vi "Omniax_mDrive_XYZR_MM_BR_RES_2_NC_GR_pxi.vi"() -> ()   [LabVIEW 2009]
uses:
  <vilib>/Instr/_visa.llb/VISA Configure Serial Port (Instr).vi
panel:
  out "XY Graph 2":cluster{"Y":dbl[], "Y":dbl[]}[](graph)
  out "XY Graph":cluster{"Y":dbl[], "Y":dbl[]}[](graph)
  out "X Scan Duration":dbl
  out "Y Scan Duration":dbl
  out "Z Scan Duration":dbl
  out "R Scan Duration":dbl
  out "R Backlash steps/sec":i32
  out "R Backlash":i32
  out "R Holding Current %":i32
  out "R Run Current %":i32
  out "R offset deg":dbl
  out "R deg/rev":dbl
  out "R steps/rev":u32
  out "R velocity PV step/sec":i32
  out "R MINPOS":i32=-94296
  out "R MAXPOS":i32=-34296
  out "R COM PORT":refnum<visa-resource-name>="COM5"
  in  "R Scan set":bool
  in  "R Scan Velocity SP deg/sec":dbl
  in  "R Scan Length SP deg":dbl
  in  "R Move Set":bool
  out "Reset R Motor Steps":i32
  in  "Reset R Position deg":dbl
  out "R Velocity MVdeg/sec":dbl
  in  "R Velocity SP deg/sec":dbl
  in  "R Position SP deg":dbl
  out "R Position MV deg":dbl
  out "R Scan velocity MV deg/sec":dbl format="%#_6f"
  out "R Scan length MV deg":dbl
  in  "R Scan Length SP steps":i32 min=0 max=6144000 step=100
  in  "R Scan OK":bool
  in  "R Velocity SP step/sec":i32 min=1 max=20000
  in  "R Scan Velocity SP steps/sec":i32=1 min=1 max=102400 step=1
  in  "R Go":bool
  in  "R Step SP":i32=-20000 min=-6144000 max=0 step=500
  out "R Position deg PV":dbl
  out "R Step PV":i32 max=2000
  out "R Backlash corr":bool
  out "R in Motion":bool
  out "R Scan":bool
  out "R in Range":bool
  out "Z COM PORT":refnum<visa-resource-name>="COM5"
  out "Z Backlash steps/sec":i32
  out "Z Backlash":i32
  out "Z Holding Current %":i32
  out "Z Run Current %":i32
  out "Z offset mm":dbl
  out "Z mm/rev":dbl
  out "Z steps/rev":u32
  out "Z  velocity PV step/sec":i32
  out "Z MINPOS":i32=-94296
  out "Z MAXPOS":i32=-34296
  in  "Z Scan set":bool
  in  "Z Scan Velocity SP mm/sec":dbl
  in  "Z Scan Length SP mm":dbl
  in  "Z Move Set":bool
  out "Reset Z Motor Steps":i32
  in  "Reset Z Position mm":dbl
  out "Z Velocity MV mm/sec":dbl
  in  "Z Velocity SP mm/sec":dbl
  in  "Z Position SP mm":dbl
  out "Z Position MV mm":dbl
  out "Z Scan velocity MV mm/sec":dbl format="%#_6f"
  out "Z Scan length MV mm":dbl
  in  "Z Scan Length SP steps":i32 min=0 max=2048000 step=100
  in  "Z Scan OK":bool
  in  "Z Velocity SP step/sec":i32 min=1 max=102400
  in  "Z Scan Velocity SP steps/sec":i32=1 min=1 max=102400 step=1
  in  "Z Go":bool
  in  "Z Step SP":i32=-20000 min=0 max=102400000 step=500
  out "Z Position mm PV":dbl
  out "Z Step PV":i32 max=2000
  out "Z Backlash corr":bool
  out "Z in Motion":bool
  out "Z Scan":bool
  out "Z in Range":bool
  out "Reset X Motor Steps":i32
  in  "Reset X Position mm":dbl
  out "X Backlash corr":bool
  out "X  in Motion":bool
  out "X Scan":bool
  out "X  in Range":bool
  out "X Step PV":i32 max=2000
  out "X Position mm PV":dbl
  out "X velocity PV step/sec":i32
  in  "X Scan set":bool
  in  "X Scan Velocity SP mm/sec":dbl
  in  "X Scan Length SP mm":dbl
  in  "X Move Set":bool
  out "X Velocity MV mm/sec":dbl
  in  "X Velocity SP mm/sec":dbl
  in  "X Position SP mm":dbl
  out "X Position MV mm":dbl
  out "X Scan velocity MV mm/sec":dbl format="%#_6f"
  out "X Scan length MV mm":dbl
  in  "X Scan Length SP steps":i32 min=-2304000 max=2304000 step=100
  in  "X Scan OK":bool
  in  "X Velocity SP step/sec":i32 min=1 max=25600
  in  "X Scan Velocity SP steps/sec":i32=1 min=1 max=102400 step=1
  in  "X Go":bool
  in  "X Step SP":i32=-20000 min=-2304000 max=2304000 step=500
  out "X Backlash steps/sec":i32
  out "X Backlash":i32
  out "X Holding Current %":i32
  out "X Run Current %":i32
  out "X offset mm":dbl
  out "X mm/rev":dbl
  out "X steps/rev":u32
  out "X MAXPOS":i32=-34296
  out "X MINPOS":i32=-94296
  out "X COM PORT":refnum<visa-resource-name>="COM5"
  out "Y Backlash corr":bool
  in  "Y Scan set":bool
  in  "Y Scan Velocity SP mm/sec":dbl
  in  "Y Scan Length SP mm":dbl
  in  "Y Move Set":bool
  out "Y Backlash steps/sec":i32
  out "Y Backlash":i32
  out "Y in Motion":bool
  in  "Reset":bool
  out "Reset Y Motor Steps":i32
  in  "Reset Y Position mm":dbl
  out "Y Velocity MV mm/sec":dbl
  in  "Y Velocity SP mm/sec":dbl
  in  "Y Position SP mm":dbl
  out "Y Position MV mm":dbl
  out "Y Holding Current %":i32
  out "Y Run Current %":i32
  out "Y Scan velocity MV mm/sec":dbl format="%#_6f"
  out "Y Scan length MV mm":dbl
  in  "Scan Cancel":bool
  out "Y Position mm PV":dbl
  out "Y offset mm":dbl
  out "Y mm/rev":dbl
  out "Y steps/rev":u32
  out "Y velocity PV step/sec":i32
  in  "Y Scan Length SP steps":i32 min=-2304000 max=2304000 step=100
  out "Y Scan":bool
  in  "Y Scan OK":bool
  in  "Scan Go":bool
  in  "Y Velocity SP step/sec":i32 min=1 max=25600
  in  "Y Scan Velocity SP steps/sec":i32=1 min=1 max=102400 step=1
  in  "Stop":bool
  out "Y in Range":bool
  out "Y Step PV":i32 max=2000
  in  "Y Go":bool
  in  "Y Step SP":i32=-20000 min=-2304000 max=2304000 step=500
  out "Y MINPOS":i32=-94296
  out "Y MAXPOS":i32=-34296
  out "Y COM PORT":refnum<visa-resource-name>="COM5"
  # "L"
  # "M"
  # "B"
  # "S"
  # "MX"
  # "MY"
  # "MZ"
  # "MR"
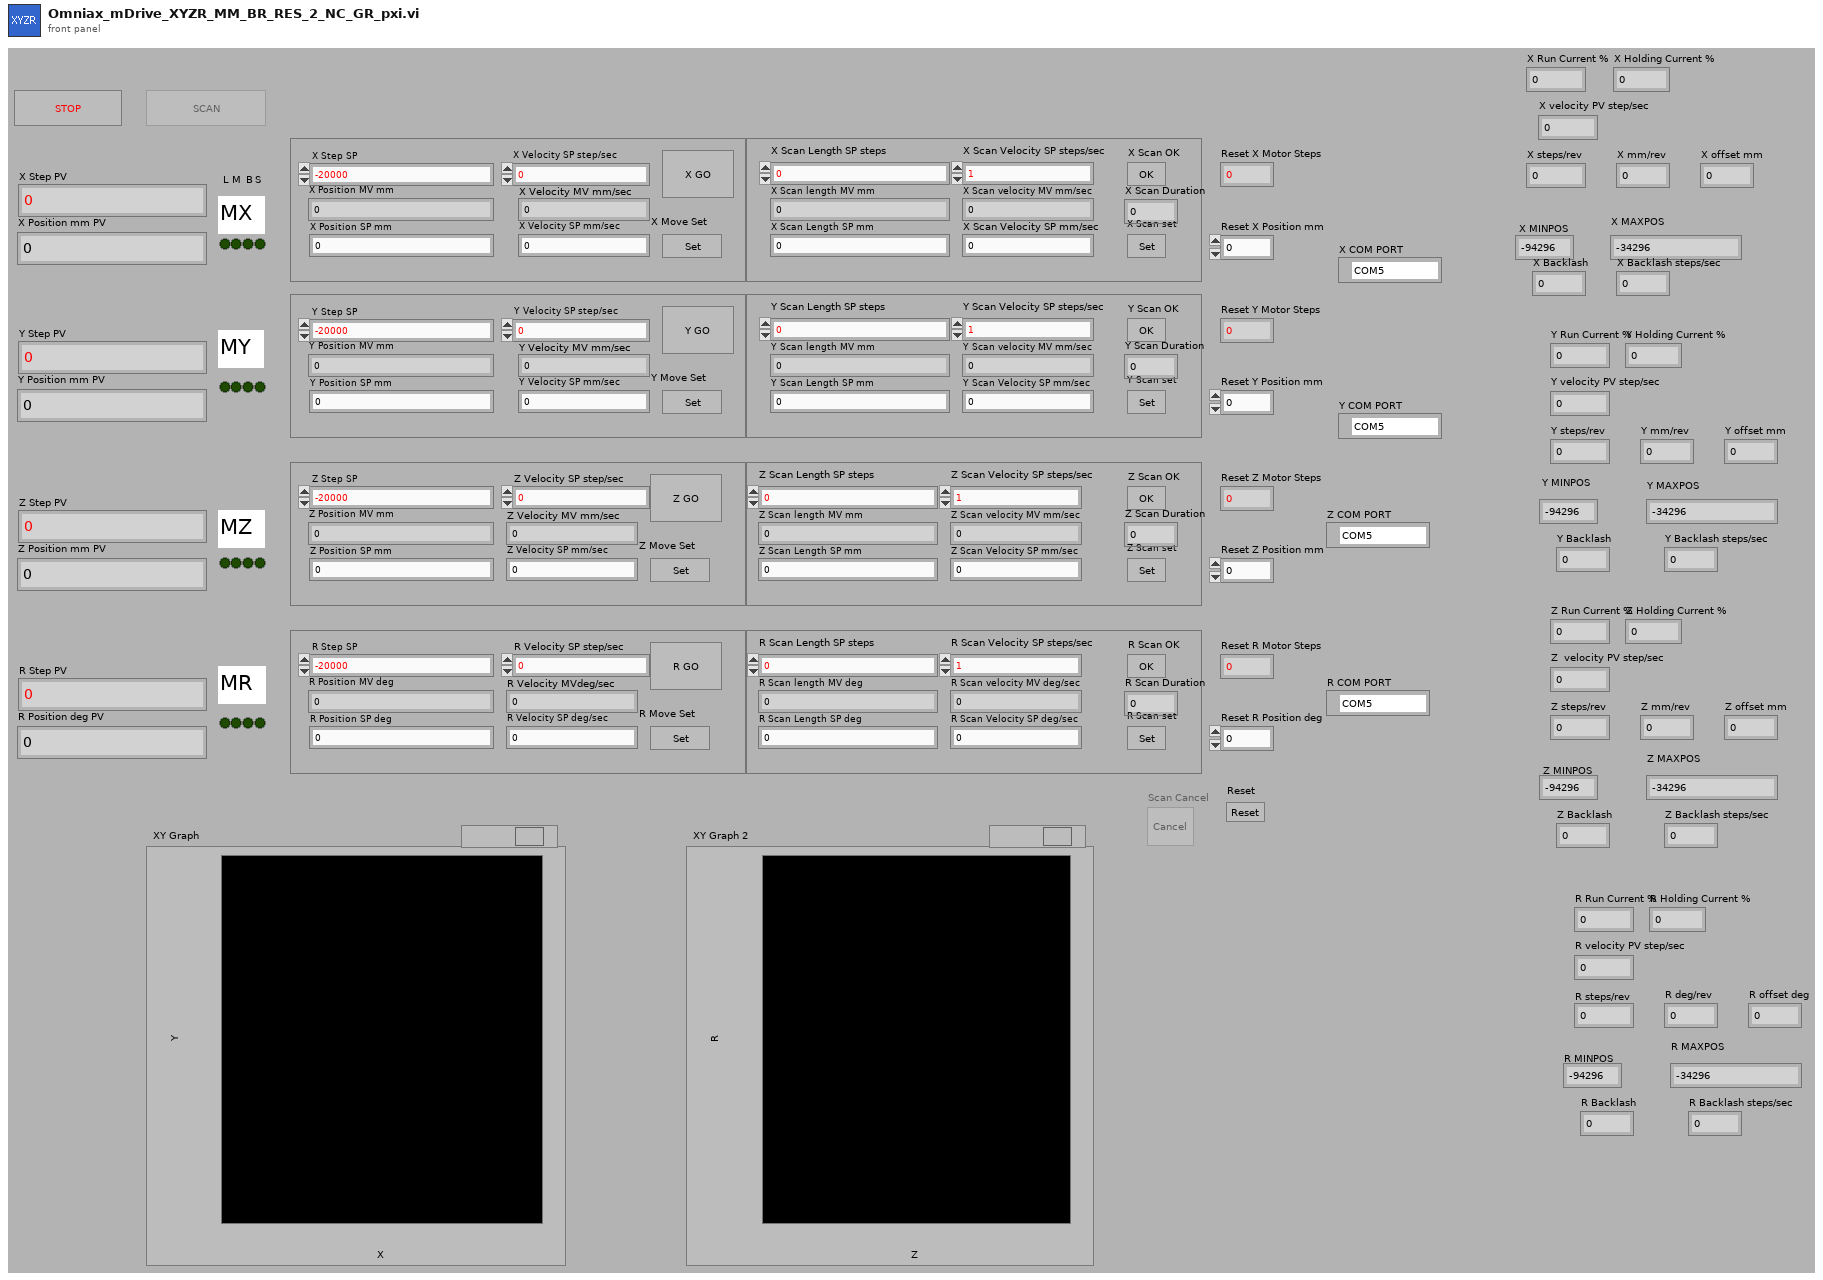
[diagram p1: front panel]
types:
  T1 = enum8{"Enabled", "Disabled", "Disabled and Grayed Out"}
  T2 = enum16{"Stop", "Reset", "Run Current", "Holding Current", "Accel Rate", "Decel Rate", "Move to Relative Position", "Move to Absolute Position", "Echo Mode", "Print Parameter", "Send String", "Microstep Resolution", "Set Current Position", "Max Velocity"}
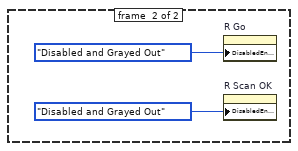
[diagram p2: hidden frame]
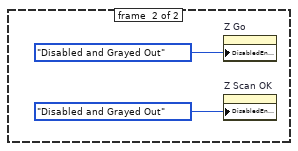
[diagram p5: hidden frame]
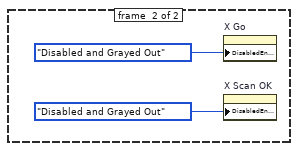
[diagram p8: hidden frame]
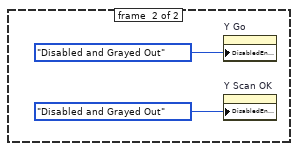
[diagram p11: hidden frame]
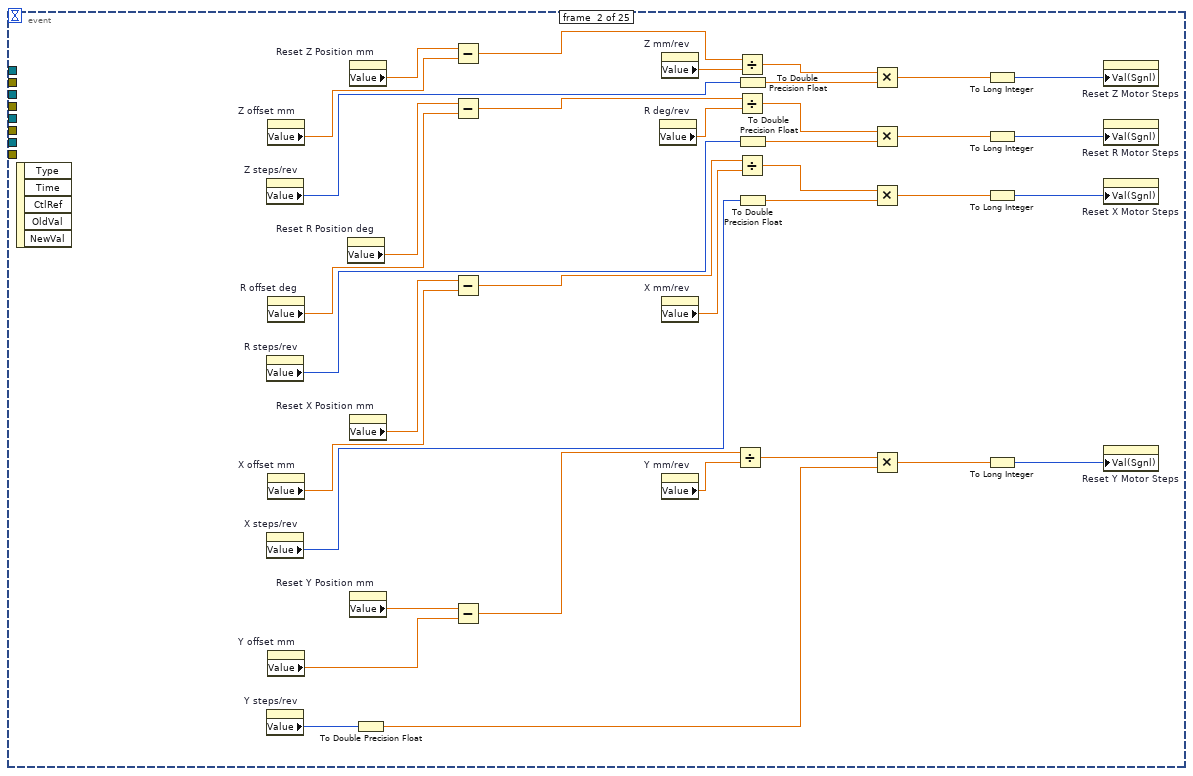
[diagram p14: hidden frame]
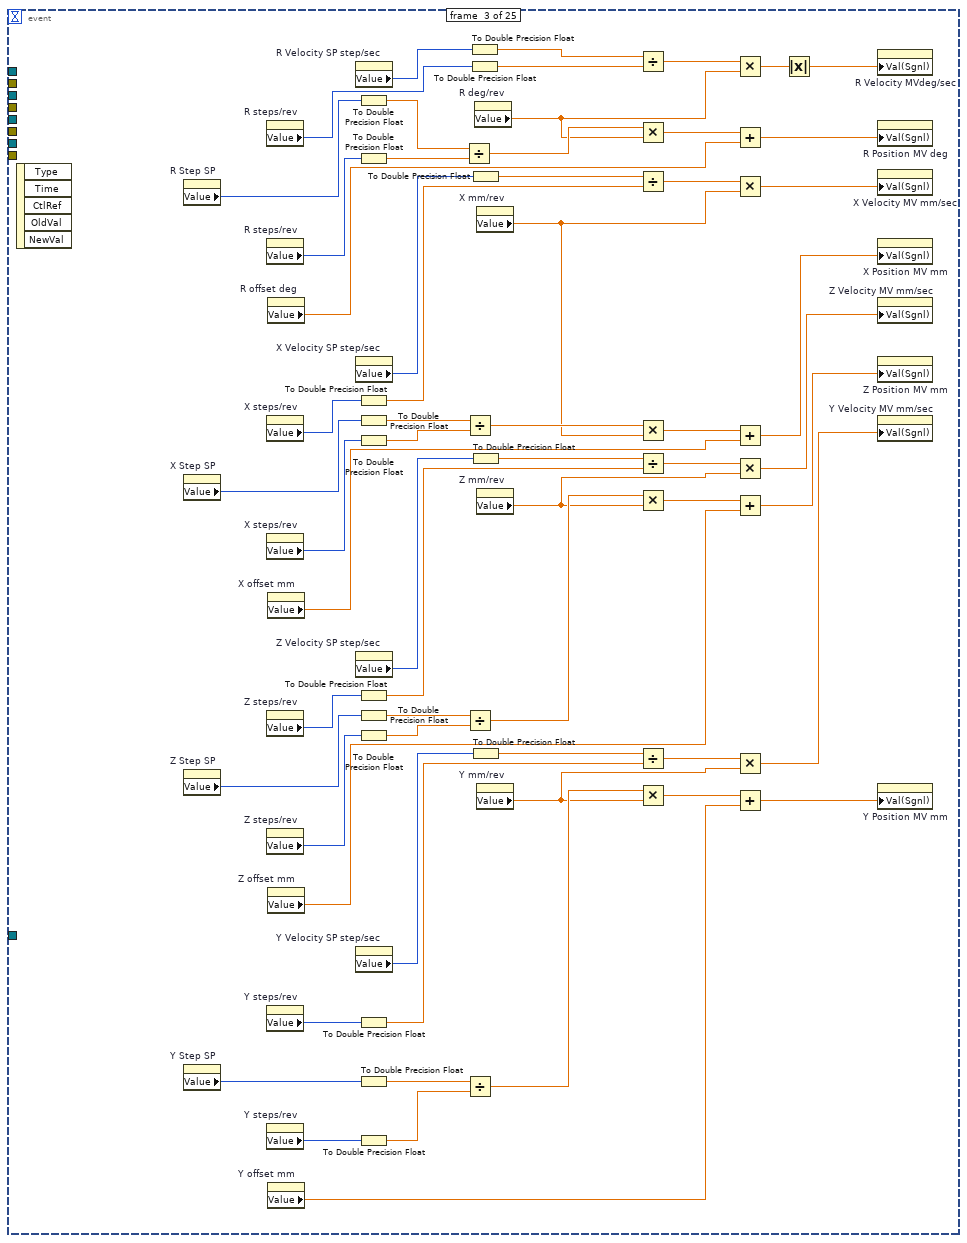
[diagram p15: hidden frame]
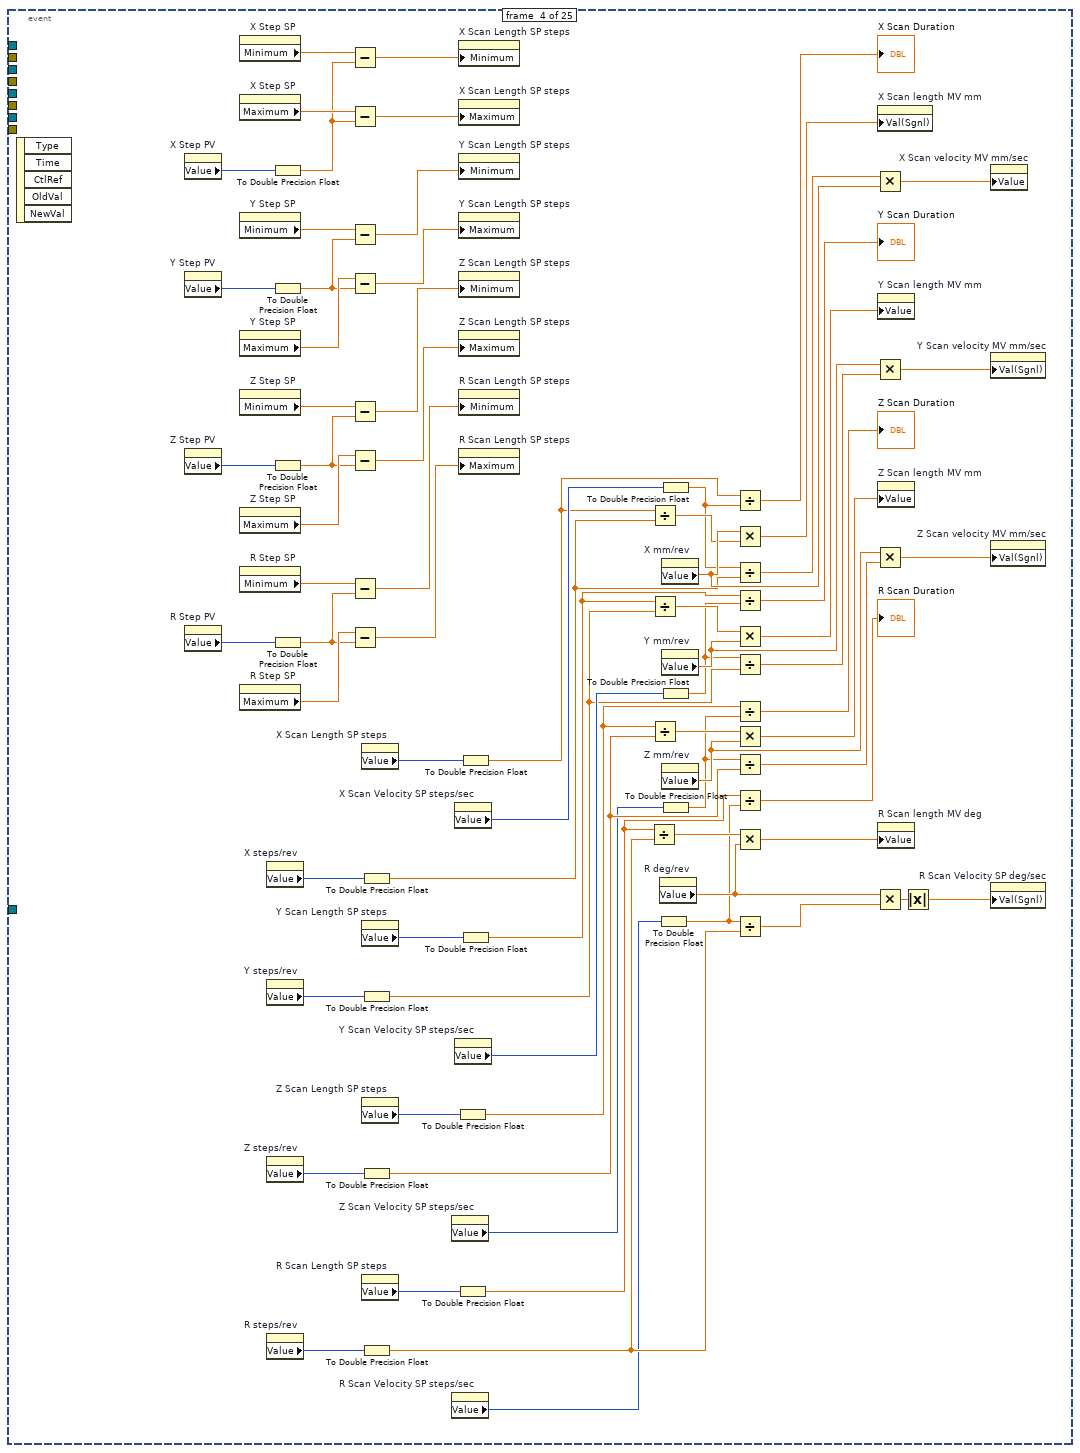
[diagram p16: hidden frame]
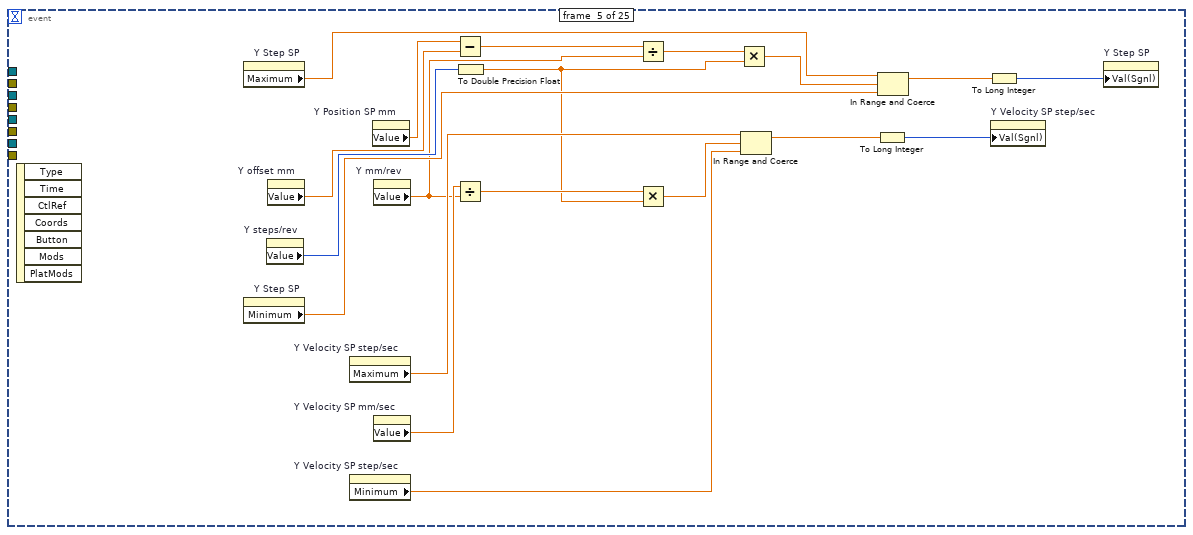
[diagram p17: hidden frame]
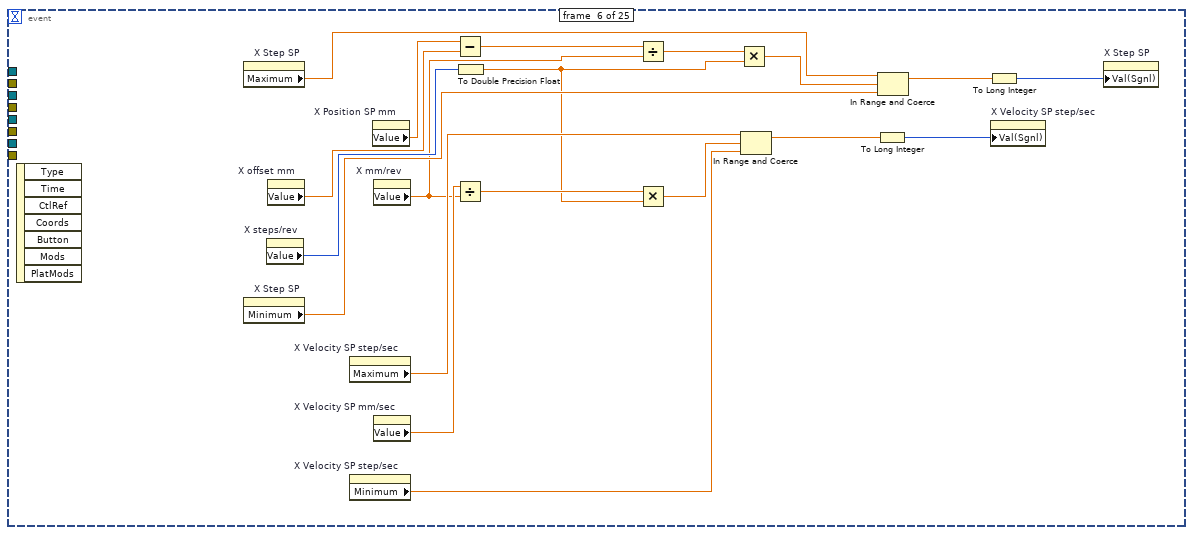
[diagram p18: hidden frame]
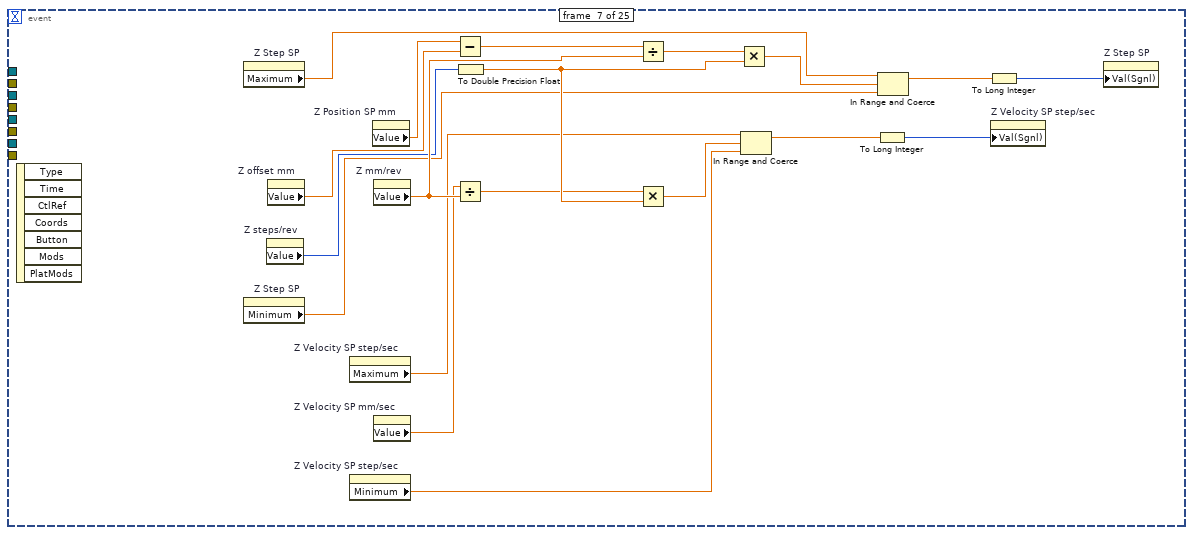
[diagram p19: hidden frame]
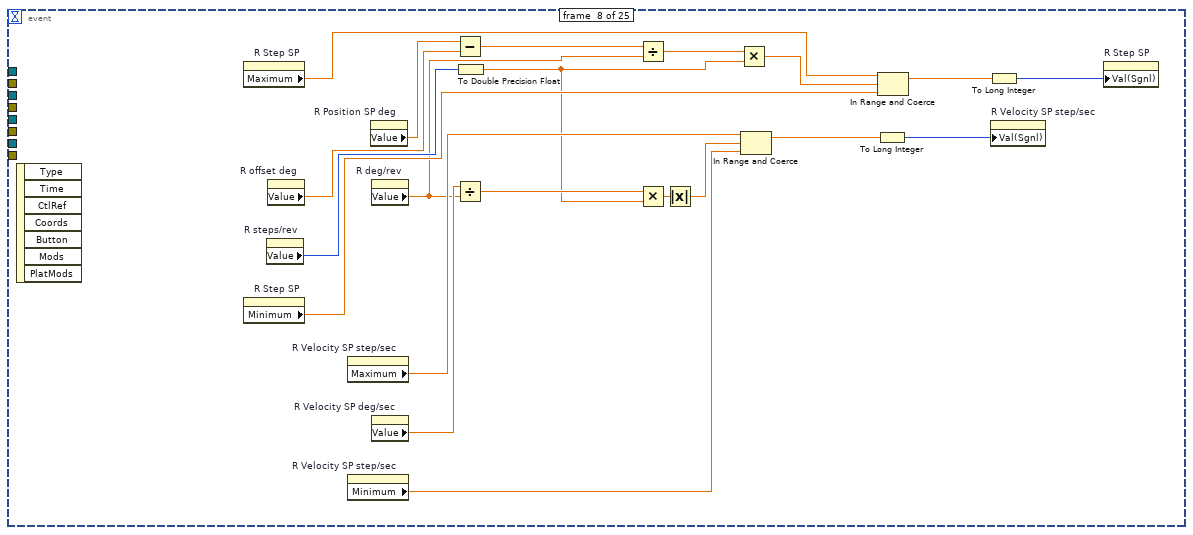
[diagram p20: hidden frame]
diagram:
  w19 = refnum<visa-resource-name> "COM7" ("COM PORT")
  w21 = u16 0 items=["None", "XON/XOFF", "RTS/CTS", "XON/XOFF & RTS/CTS", "DTR/DSR", "XON/XOFF & DTR/DSR"] ("flow control (0:none)")
  w22 = u16 10 items=["1.0"=10, "1.5"=15, "2.0"=20] ("stop bits (10: 1 bit)")
  w52 = refnum<visa-resource-name> "COM6" ("COM PORT")
  w54 = u16 0 items=["None", "XON/XOFF", "RTS/CTS", "XON/XOFF & RTS/CTS", "DTR/DSR", "XON/XOFF & DTR/DSR"] ("flow control (0:none)")
  w55 = u16 10 items=["1.0"=10, "1.5"=15, "2.0"=20] ("stop bits (10: 1 bit)")
  w65 = refnum<visa-resource-name> "COM4" ("COM PORT")
  w67 = u16 0 items=["None", "XON/XOFF", "RTS/CTS", "XON/XOFF & RTS/CTS", "DTR/DSR", "XON/XOFF & DTR/DSR"] ("flow control (0:none)")
  w68 = u16 10 items=["1.0"=10, "1.5"=15, "2.0"=20] ("stop bits (10: 1 bit)")
  w90 = refnum<visa-resource-name> "COM5" ("COM PORT")
  w92 = u16 0 items=["None", "XON/XOFF", "RTS/CTS", "XON/XOFF & RTS/CTS", "DTR/DSR", "XON/XOFF & DTR/DSR"] ("flow control (0:none)")
  w93 = u16 10 items=["1.0"=10, "1.5"=15, "2.0"=20] ("stop bits (10: 1 bit)")
  # "Stop bits"
  # "Stop bits"
  # "Stop bits"
  # "Stop bits"
  n1 = flat-sequence {
    frame #0 {
      "Z Holding Current %" <- 20 ("Z Holding Current %")
      "Z Run Current %" <- 100 ("Z Run Current %")
      "X Run Current %" <- 40 ("Run Current %")
      "X Holding Current %" <- 20 ("Holding Current %")
      "Y Run Current %" <- 40 ("Run Current %")
      "Y Holding Current %" <- 20 ("Holding Current %")
      "R Holding Current %" <- 20 ("R Holding Current %")
      "R Run Current %" <- 100 ("R Run Current %")
    }
  }
  n2 = flat-sequence {
    frame #0 {
      w110 = -3.0 ("R deg/rev")
      w108 = u32 51200 ("step/rev")
      w112 = 20000 ("Value (Signaling)")
      n3 = To Double Precision Float(number=w112) -> (double precision float=w114:dbl)
      n4 = To Double Precision Float(number=w108) -> (double precision float=w109:dbl)
      n5 = property on="R Velocity SP step/sec" class="DigNum (strict)"("Val(Sgnl)"=w112) -> ()  [unwired: 2 in, 2 out]
      n6 = property on="R Velocity SP step/sec" class="DigNum (strict)"("Minimum"=1.0 ("Data Entry Limits:Minimum")) -> ()  [unwired: 2 in, 2 out]
      n7 = Divide(x=w114, y=w109) -> (x/y=w113:dbl)
      n8 = property on="R Velocity SP step/sec" class="DigNum (strict)"("Maximum"=w114) -> ()  [unwired: 2 in, 2 out]
      n9 = Multiply(x=w113, y=w110) -> (x*y=w111:dbl)
      n10 = Absolute Value(x=w111) -> (abs(x)=w105:dbl)
      n11 = property on="R Velocity SP deg/sec" class="DigNum (strict)"("Val(Sgnl)"=w105) -> ()  [unwired: 2 in, 2 out]
      "R offset deg" <- 0.0 ("R offset deg")
      "R deg/rev" <- w110
      "R steps/rev" <- w108
    }
  }
  n12 = flat-sequence {
    frame #0 {
      w116 = 0.2 ("Z mm/rev")
      w115 = u32 51200 ("step/rev")
      w117 = 102400 ("Value (Signaling)")
      n13 = To Double Precision Float(number=w117) -> (double precision float=w121:dbl)
      n14 = To Double Precision Float(number=w115) -> (double precision float=w120:dbl)
      n15 = property on="Z Velocity SP step/sec" class="DigNum (strict)"("Val(Sgnl)"=w117) -> ()  [unwired: 2 in, 2 out]
      n16 = property on="Z Velocity SP step/sec" class="DigNum (strict)"("Minimum"=1.0 ("Data Entry Limits:Minimum")) -> ()  [unwired: 2 in, 2 out]
      n17 = Divide(x=w121, y=w120) -> (x/y=w118:dbl)
      n18 = property on="Z Velocity SP step/sec" class="DigNum (strict)"("Maximum"=w121) -> ()  [unwired: 2 in, 2 out]
      n19 = Multiply(x=w118, y=w116) -> (x*y=w119:dbl)
      n20 = property on="Z Velocity SP mm/sec" class="DigNum (strict)"("Val(Sgnl)"=w119) -> ()  [unwired: 2 in, 2 out]
      "Z offset mm" <- 0.0 ("Z offset mm")
      "Z mm/rev" <- w116
      "Z steps/rev" <- w115
    }
  }
  n21 = flat-sequence {
    frame #0 {
      n22 = property on="R Backlash corr" class="Bool (strict)"("Val(Sgnl)"=FALSE ("Value (Signaling)")) -> ()  [unwired: 2 in, 2 out]
      n23 = property on="Y Backlash corr" class="Bool (strict)"("Val(Sgnl)"=FALSE ("Value (Signaling)")) -> ()  [unwired: 2 in, 2 out]
      n24 = property on="Z Backlash corr" class="Bool (strict)"("Val(Sgnl)"=FALSE ("Value (Signaling)")) -> ()  [unwired: 2 in, 2 out]
      n25 = property on="X Backlash corr" class="Bool (strict)"("Val(Sgnl)"=FALSE ("Value (Signaling)")) -> ()  [unwired: 2 in, 2 out]
      "Z Backlash steps/sec" <- 25600 ("Z Backlash steps/sec")
      "Z Backlash" <- -12800 ("Z Backlash")
      "X Backlash steps/sec" <- 25600 ("Value (Signaling)")
      "X Backlash" <- -5120 ("Backlash2")
      "Y Backlash" <- -5120 ("Backlash2")
      "Y Backlash steps/sec" <- 25600 ("Value (Signaling)")
      "R Backlash steps/sec" <- 6400 ("R Backlash steps/sec")
      "R Backlash" <- -12800 ("R Backlash")
    }
  }
  n26 = flat-sequence {
    frame #0 {
      n27 = property on="X Scan" class="Bool (strict)"("Val(Sgnl)"=FALSE ("Value (Signaling)")) -> ()  [unwired: 2 in, 2 out]
      n28 = property on="R Velocity SP deg/sec" class="DigNum (strict)"("Val(Sgnl)"=0.1 ("Value (Signaling)")) -> ()  [unwired: 2 in, 2 out]
      n29 = property on="Y Scan Velocity SP mm/sec" class="DigNum (strict)"("Val(Sgnl)"=0.1 ("Value (Signaling)")) -> ()  [unwired: 2 in, 2 out]
      n30 = property on="Y Scan" class="Bool (strict)"("Val(Sgnl)"=FALSE ("Value (Signaling)")) -> ()  [unwired: 2 in, 2 out]
      n31 = property on="Z Scan Velocity SP mm/sec" class="DigNum (strict)"("Val(Sgnl)"=0.1 ("Value (Signaling)")) -> ()  [unwired: 2 in, 2 out]
      n32 = property on="Z Scan" class="Bool (strict)"("Val(Sgnl)"=FALSE ("Value (Signaling)")) -> ()  [unwired: 2 in, 2 out]
      n33 = property on="X Scan Velocity SP mm/sec" class="DigNum (strict)"("Val(Sgnl)"=0.1 ("Value (Signaling)")) -> ()  [unwired: 2 in, 2 out]
      n34 = property on="R Scan" class="Bool (strict)"("Val(Sgnl)"=FALSE ("Value (Signaling)")) -> ()  [unwired: 2 in, 2 out]
      n35 = property on="Scan Cancel" class="Bool"("DisabledEnum"=T1."Disabled and Grayed Out" ("Disabled")) -> ()  [unwired: 2 in, 2 out]
      n36 = property on="Scan Go" class="Bool"("DisabledEnum"=T1."Disabled and Grayed Out" ("Disabled")) -> ()  [unwired: 2 in, 2 out]
    }
  }
  n37 = flat-sequence {
    frame #0 {
      w148 = 0.2 ("MM/rev")
      w151 = u32 51200 ("step/rev")
      w146 = 25600 ("Value (Signaling)")
      n38 = To Double Precision Float(number=w146) -> (double precision float=w152:dbl)
      n39 = To Double Precision Float(number=w151) -> (double precision float=w150:dbl)
      n40 = property on="X Velocity SP step/sec" class="DigNum (strict)"("Minimum"=1.0 ("Data Entry Limits:Minimum")) -> ()  [unwired: 2 in, 2 out]
      n41 = property on="X Velocity SP step/sec" class="DigNum (strict)"("Val(Sgnl)"=w146) -> ()  [unwired: 2 in, 2 out]
      n42 = Divide(x=w152, y=w150) -> (x/y=w147:dbl)
      n43 = property on="X Velocity SP step/sec" class="DigNum (strict)"("Maximum"=w152) -> ()  [unwired: 2 in, 2 out]
      n44 = Multiply(x=w147, y=w148) -> (x*y=w149:dbl)
      n45 = property on="X Velocity SP mm/sec" class="DigNum (strict)"("Val(Sgnl)"=w149) -> ()  [unwired: 2 in, 2 out]
      "X offset mm" <- 0.0 ("offset")
      "X steps/rev" <- w151
      "X mm/rev" <- w148
    }
  }
  n46 = flat-sequence {
    frame #0 {
      w157 = 0.2 ("MM/rev")
      w160 = u32 51200 ("step/rev")
      w155 = 25600 ("Value (Signaling)")
      n47 = To Double Precision Float(number=w155) -> (double precision float=w161:dbl)
      n48 = To Double Precision Float(number=w160) -> (double precision float=w159:dbl)
      n49 = property on="Y Velocity SP step/sec" class="DigNum (strict)"("Minimum"=1.0 ("Data Entry Limits:Minimum")) -> ()  [unwired: 2 in, 2 out]
      n50 = property on="Y Velocity SP step/sec" class="DigNum (strict)"("Val(Sgnl)"=w155) -> ()  [unwired: 2 in, 2 out]
      n51 = Divide(x=w161, y=w159) -> (x/y=w156:dbl)
      n52 = property on="Y Velocity SP step/sec" class="DigNum (strict)"("Maximum"=w161) -> ()  [unwired: 2 in, 2 out]
      n53 = Multiply(x=w156, y=w157) -> (x*y=w158:dbl)
      n54 = property on="Y Velocity SP mm/sec" class="DigNum (strict)"("Val(Sgnl)"=w158) -> ()  [unwired: 2 in, 2 out]
      "Y offset mm" <- 0.0 ("offset")
      "Y steps/rev" <- w160
      "Y mm/rev" <- w157
    }
  }
  n55 = call-poly "VISA Configure Serial Port"("VISA resource name"=w90, "timeout (10sec)"=u32 10000, "baud rate (9600)"=u32 9600, "data bits (8)"=u16 8, "parity (0:none)"=enum16{"None", "Odd", "Even", "Mark", "Space"}."None", "stop bits (10: 1 bit)"=w93, "flow control (0:none)"=w92) -> ("VISA resource name out"=w83:refnum<visa-resource-name>, "error out"=w82:errorcluster)  [unwired: 7 in]
  n56 = flat-sequence {
    tunnel: w82 -> [w165]
    tunnel: w83 -> [w167]
    tunnel: [w166] -> w4
    tunnel: [w164] -> w3
    tunnel: [w173] -> w81
    tunnel: [w175] -> w79
    tunnel: w4 -> [w174]
    tunnel: w3 -> [w176]
    tunnel: w81 -> [w183]
    tunnel: [w182] -> w80
    tunnel: w79 -> [w180]
    tunnel: [w181] -> w78
    tunnel: [w193] -> w85
    tunnel: [w194] -> w84
    tunnel: w80 -> [w192]
    tunnel: w78 -> [w191]
    tunnel: w85 -> [w204]
    tunnel: w84 -> [w203]
    tunnel: [w206] -> w51
    tunnel: [w205] -> w50
    tunnel: [w200] -> w49
    tunnel: [w211] -> w88
    tunnel: [w212] -> w89
    tunnel: w51 -> [w212]
    tunnel: w50 -> [w211]
    tunnel: w49 -> [w207]
    frame #0 {
      n57 = call "mDrive Send Command.vi"("error in (no error)"=w165, "Extra"="EM=2", "Command"=T2."Send String", "VISA resource name"=w167) -> ("error out"=w164:errorcluster, "VISA resource name out"=w166:refnum<visa-resource-name>)  [unwired: 3 in, 1 out]
    }
    frame #1 {
      # "Run Current %"
      n58 = property on="Y Run Current %" class="DigNum (strict)"() -> ("Value"=w171:i32)  [unwired: 2 in, 2 out]
      n59 = Number To Decimal String(number=w171) -> (decimal integer string=w172:string)  [unwired: 1 in]
      n60 = call "mDrive Send Command.vi"("error in (no error)"=w176, "Extra"=w172, "Command"=T2."Run Current", "VISA resource name"=w174) -> ("error out"=w175:errorcluster, "VISA resource name out"=w173:refnum<visa-resource-name>)  [unwired: 3 in, 1 out]
    }
    frame #2 {
      # "Holding Current %"
      n61 = property on="Y Holding Current %" class="DigNum (strict)"() -> ("Value"=w178:i32)  [unwired: 2 in, 2 out]
      n62 = Number To Decimal String(number=w178) -> (decimal integer string=w179:string)  [unwired: 1 in]
      n63 = call "mDrive Send Command.vi"("error in (no error)"=w180, "Extra"=w179, "Command"=T2."Holding Current", "VISA resource name"=w183) -> ("error out"=w181:errorcluster, "VISA resource name out"=w182:refnum<visa-resource-name>)  [unwired: 3 in, 1 out]
    }
    frame #3 {
      # "Print Velocity Ma"
      # "Velocity Max"
      n64 = property on="Y Velocity SP step/sec" class="DigNum (strict)"() -> ("Value"=w190:i32)  [unwired: 2 in, 2 out]
      n65 = Number To Decimal String(number=w190) -> (decimal integer string=w189:string)  [unwired: 1 in]
      n66 = call "mDrive Send Command.vi"("error in (no error)"=w191, "Extra"=w189, "Command"=T2."Max Velocity", "VISA resource name"=w192) -> ("error out"=w187:errorcluster, "VISA resource name out"=w197:refnum<visa-resource-name>)  [unwired: 3 in, 1 out]
      n67 = call "mDrive Send Command.vi"("error in (no error)"=w187, "Extra"="VM", "Command"=T2."Print Parameter", "VISA resource name"=w197) -> ("error out"=w194:errorcluster, "read buffer"=w195:string, "VISA resource name out"=w193:refnum<visa-resource-name>)  [unwired: 3 in]
      n68 = Decimal String To Number(string=w195, offset=0) -> (number=w188:i32)  [unwired: 1 in, 1 out]
      n69 = property on="Y scan velocity MV step/sec" class="DigNum (strict)"("Val(Sgnl)"=w188) -> ()  [unwired: 2 in, 2 out]
    }
    frame #4 {
      # "PRINT POSITION"
      n70 = call "mDrive Send Command.vi"("error in (no error)"=w203, "Extra"="P", "Command"=T2."Print Parameter", "VISA resource name"=w204) -> ("error out"=w205:errorcluster, "read buffer"=w202:string, "VISA resource name out"=w206:refnum<visa-resource-name>)  [unwired: 3 in]
      n71 = Decimal String To Number(string=w202, offset=0) -> (number=w200:i32)  [unwired: 1 in, 1 out]
    }
    frame #5 {
      w209 = -2304000 ("lower limit")
      w210 = 2304000 ("upper limit")
      n72 = property on="Y Step SP" class="DigNum (strict)"("Val(Sgnl)"=w207) -> ()  [unwired: 2 in, 2 out]
      n73 = property on="Y Step SP" class="DigNum (strict)"("Maximum"=w210) -> ()  [unwired: 2 in, 2 out]
      n74 = property on="Y Step SP" class="DigNum (strict)"("Minimum"=w209) -> ()  [unwired: 2 in, 2 out]
      n75 = In Range and Coerce(upper limit=w210, x=w207, lower limit=w209) -> (In Range?=w208:bool)  [unwired: 1 out]
      n76 = property on="Y in Range" class="Bool (strict)"("Val(Sgnl)"=w208) -> ()  [unwired: 2 in, 2 out]
      "Y MINPOS" <- w209
      "Y MAXPOS" <- w210
    }
  }
  n77 = call-poly "VISA Configure Serial Port"("VISA resource name"=w19, "timeout (10sec)"=u32 10000, "baud rate (9600)"=u32 9600, "data bits (8)"=u16 8, "parity (0:none)"=enum16{"None", "Odd", "Even", "Mark", "Space"}."None", "stop bits (10: 1 bit)"=w22, "flow control (0:none)"=w21) -> ("VISA resource name out"=w18:refnum<visa-resource-name>, "error out"=w17:errorcluster)  [unwired: 7 in]
  n78 = call-poly "VISA Configure Serial Port"("VISA resource name"=w65, "timeout (10sec)"=u32 10000, "baud rate (9600)"=u32 9600, "data bits (8)"=u16 8, "parity (0:none)"=enum16{"None", "Odd", "Even", "Mark", "Space"}."None", "stop bits (10: 1 bit)"=w68, "flow control (0:none)"=w67) -> ("VISA resource name out"=w64:refnum<visa-resource-name>, "error out"=w63:errorcluster)  [unwired: 7 in]
  n79 = flat-sequence {
    tunnel: w17 -> [w216]
    tunnel: w18 -> [w214]
    tunnel: [w213] -> w8
    tunnel: [w215] -> w7
    tunnel: [w223] -> w34
    tunnel: [w225] -> w33
    tunnel: w8 -> [w224]
    tunnel: w7 -> [w219]
    tunnel: w34 -> [w232]
    tunnel: [w231] -> w32
    tunnel: w33 -> [w229]
    tunnel: [w230] -> w31
    tunnel: [w242] -> w30
    tunnel: [w243] -> w29
    tunnel: w32 -> [w241]
    tunnel: w31 -> [w240]
    tunnel: w30 -> [w253]
    tunnel: w29 -> [w252]
    tunnel: [w255] -> w28
    tunnel: [w254] -> w27
    tunnel: [w249] -> w26
    tunnel: [w260] -> w11
    tunnel: [w261] -> w12
    tunnel: w28 -> [w261]
    tunnel: w27 -> [w260]
    tunnel: w26 -> [w258]
    frame #0 {
      n80 = call "mDrive Send Command.vi"("error in (no error)"=w216, "Extra"="EM=2", "Command"=T2."Send String", "VISA resource name"=w214) -> ("error out"=w215:errorcluster, "VISA resource name out"=w213:refnum<visa-resource-name>)  [unwired: 3 in, 1 out]
    }
    frame #1 {
      # "Run Current %"
      n81 = property on="R Run Current %" class="DigNum (strict)"() -> ("Value"=w221:i32)  [unwired: 2 in, 2 out]
      n82 = Number To Decimal String(number=w221) -> (decimal integer string=w222:string)  [unwired: 1 in]
      n83 = call "mDrive Send Command.vi"("error in (no error)"=w219, "Extra"=w222, "Command"=T2."Run Current", "VISA resource name"=w224) -> ("error out"=w225:errorcluster, "VISA resource name out"=w223:refnum<visa-resource-name>)  [unwired: 3 in, 1 out]
    }
    frame #2 {
      # "Holding Current %"
      n84 = property on="R Holding Current %" class="DigNum (strict)"() -> ("Value"=w227:i32)  [unwired: 2 in, 2 out]
      n85 = Number To Decimal String(number=w227) -> (decimal integer string=w228:string)  [unwired: 1 in]
      n86 = call "mDrive Send Command.vi"("error in (no error)"=w229, "Extra"=w228, "Command"=T2."Holding Current", "VISA resource name"=w232) -> ("error out"=w230:errorcluster, "VISA resource name out"=w231:refnum<visa-resource-name>)  [unwired: 3 in, 1 out]
    }
    frame #3 {
      # "Print Velocity Ma"
      # "Velocity Max"
      n87 = property on="R Velocity SP step/sec" class="DigNum (strict)"() -> ("Value"=w239:i32)  [unwired: 2 in, 2 out]
      n88 = Number To Decimal String(number=w239) -> (decimal integer string=w238:string)  [unwired: 1 in]
      n89 = call "mDrive Send Command.vi"("error in (no error)"=w240, "Extra"=w238, "Command"=T2."Max Velocity", "VISA resource name"=w241) -> ("error out"=w236:errorcluster, "VISA resource name out"=w246:refnum<visa-resource-name>)  [unwired: 3 in, 1 out]
      n90 = call "mDrive Send Command.vi"("error in (no error)"=w236, "Extra"="VM", "Command"=T2."Print Parameter", "VISA resource name"=w246) -> ("error out"=w243:errorcluster, "read buffer"=w244:string, "VISA resource name out"=w242:refnum<visa-resource-name>)  [unwired: 3 in]
      n91 = Decimal String To Number(string=w244, offset=0) -> (number=w237:i32)  [unwired: 1 in, 1 out]
      n92 = property on="R velocity PV step/sec" class="DigNum (strict)"("Val(Sgnl)"=w237) -> ()  [unwired: 2 in, 2 out]
    }
    frame #4 {
      # "PRINT POSITION"
      n93 = call "mDrive Send Command.vi"("error in (no error)"=w252, "Extra"="P", "Command"=T2."Print Parameter", "VISA resource name"=w253) -> ("error out"=w254:errorcluster, "read buffer"=w251:string, "VISA resource name out"=w255:refnum<visa-resource-name>)  [unwired: 3 in]
      n94 = Decimal String To Number(string=w251, offset=0) -> (number=w249:i32)  [unwired: 1 in, 1 out]
    }
    frame #5 {
      w257 = -6144000 ("lower limit")
      w256 = 0 ("upper limit")
      n95 = property on="R Step SP" class="DigNum (strict)"("Val(Sgnl)"=w258) -> ()  [unwired: 2 in, 2 out]
      n96 = property on="R Step SP" class="DigNum (strict)"("Maximum"=w256) -> ()  [unwired: 2 in, 2 out]
      n97 = In Range and Coerce(upper limit=w256, x=w258, lower limit=w257) -> (In Range?=w259:bool)  [unwired: 1 out]
      n98 = property on="R Step SP" class="DigNum (strict)"("Minimum"=w257) -> ()  [unwired: 2 in, 2 out]
      n99 = property on="R in Range" class="Bool (strict)"("Val(Sgnl)"=w259) -> ()  [unwired: 2 in, 2 out]
      "R MINPOS" <- w257
      "R MAXPOS" <- w256
    }
  }
  n100 = flat-sequence {
    tunnel: w63 -> [w263]
    tunnel: w64 -> [w265]
    tunnel: [w264] -> w2
    tunnel: [w262] -> w1
    tunnel: [w271] -> w77
    tunnel: [w273] -> w76
    tunnel: w2 -> [w272]
    tunnel: w1 -> [w274]
    tunnel: w77 -> [w281]
    tunnel: [w280] -> w75
    tunnel: w76 -> [w278]
    tunnel: [w279] -> w74
    tunnel: [w291] -> w73
    tunnel: [w292] -> w72
    tunnel: w75 -> [w290]
    tunnel: w74 -> [w289]
    tunnel: w73 -> [w302]
    tunnel: w72 -> [w301]
    tunnel: [w304] -> w48
    tunnel: [w303] -> w47
    tunnel: [w298] -> w46
    tunnel: [w309] -> w61
    tunnel: [w310] -> w62
    tunnel: w48 -> [w310]
    tunnel: w47 -> [w309]
    tunnel: w46 -> [w305]
    frame #0 {
      n101 = call "mDrive Send Command.vi"("error in (no error)"=w263, "Extra"="EM=2", "Command"=T2."Send String", "VISA resource name"=w265) -> ("error out"=w262:errorcluster, "VISA resource name out"=w264:refnum<visa-resource-name>)  [unwired: 3 in, 1 out]
    }
    frame #1 {
      # "Run Current %"
      n102 = property on="X Run Current %" class="DigNum (strict)"() -> ("Value"=w269:i32)  [unwired: 2 in, 2 out]
      n103 = Number To Decimal String(number=w269) -> (decimal integer string=w270:string)  [unwired: 1 in]
      n104 = call "mDrive Send Command.vi"("error in (no error)"=w274, "Extra"=w270, "Command"=T2."Run Current", "VISA resource name"=w272) -> ("error out"=w273:errorcluster, "VISA resource name out"=w271:refnum<visa-resource-name>)  [unwired: 3 in, 1 out]
    }
    frame #2 {
      # "Holding Current %"
      n105 = property on="X Holding Current %" class="DigNum (strict)"() -> ("Value"=w276:i32)  [unwired: 2 in, 2 out]
      n106 = Number To Decimal String(number=w276) -> (decimal integer string=w277:string)  [unwired: 1 in]
      n107 = call "mDrive Send Command.vi"("error in (no error)"=w278, "Extra"=w277, "Command"=T2."Holding Current", "VISA resource name"=w281) -> ("error out"=w279:errorcluster, "VISA resource name out"=w280:refnum<visa-resource-name>)  [unwired: 3 in, 1 out]
    }
    frame #3 {
      # "Print Velocity Ma"
      # "Velocity Max"
      n108 = property on="X Velocity SP step/sec" class="DigNum (strict)"() -> ("Value"=w288:i32)  [unwired: 2 in, 2 out]
      n109 = Number To Decimal String(number=w288) -> (decimal integer string=w287:string)  [unwired: 1 in]
      n110 = call "mDrive Send Command.vi"("error in (no error)"=w289, "Extra"=w287, "Command"=T2."Max Velocity", "VISA resource name"=w290) -> ("error out"=w285:errorcluster, "VISA resource name out"=w295:refnum<visa-resource-name>)  [unwired: 3 in, 1 out]
      n111 = call "mDrive Send Command.vi"("error in (no error)"=w285, "Extra"="VM", "Command"=T2."Print Parameter", "VISA resource name"=w295) -> ("error out"=w292:errorcluster, "read buffer"=w293:string, "VISA resource name out"=w291:refnum<visa-resource-name>)  [unwired: 3 in]
      n112 = Decimal String To Number(string=w293, offset=0) -> (number=w286:i32)  [unwired: 1 in, 1 out]
      n113 = property on="X velocity PV step/sec" class="DigNum (strict)"("Val(Sgnl)"=w286) -> ()  [unwired: 2 in, 2 out]
    }
    frame #4 {
      # "PRINT POSITION"
      n114 = call "mDrive Send Command.vi"("error in (no error)"=w301, "Extra"="P", "Command"=T2."Print Parameter", "VISA resource name"=w302) -> ("error out"=w303:errorcluster, "read buffer"=w300:string, "VISA resource name out"=w304:refnum<visa-resource-name>)  [unwired: 3 in]
      n115 = Decimal String To Number(string=w300, offset=0) -> (number=w298:i32)  [unwired: 1 in, 1 out]
    }
    frame #5 {
      w307 = -2304000 ("lower limit")
      w308 = 2304000 ("upper limit")
      n116 = property on="X Step SP" class="DigNum (strict)"("Val(Sgnl)"=w305) -> ()  [unwired: 2 in, 2 out]
      n117 = property on="X Step SP" class="DigNum (strict)"("Maximum"=w308) -> ()  [unwired: 2 in, 2 out]
      n118 = In Range and Coerce(upper limit=w308, x=w305, lower limit=w307) -> (In Range?=w306:bool)  [unwired: 1 out]
      n119 = property on="X Step SP" class="DigNum (strict)"("Minimum"=w307) -> ()  [unwired: 2 in, 2 out]
      n120 = property on="X  in Range" class="Bool (strict)"("Val(Sgnl)"=w306) -> ()  [unwired: 2 in, 2 out]
      "X MINPOS" <- w307
      "X MAXPOS" <- w308
    }
  }
  n121 = call-poly "VISA Configure Serial Port"("VISA resource name"=w52, "timeout (10sec)"=u32 10000, "baud rate (9600)"=u32 9600, "data bits (8)"=u16 8, "parity (0:none)"=enum16{"None", "Odd", "Even", "Mark", "Space"}."None", "stop bits (10: 1 bit)"=w55, "flow control (0:none)"=w54) -> ("VISA resource name out"=w36:refnum<visa-resource-name>, "error out"=w35:errorcluster)  [unwired: 7 in]
  n122 = flat-sequence {
    tunnel: w35 -> [w311]
    tunnel: w36 -> [w314]
    tunnel: [w313] -> w6
    tunnel: [w312] -> w5
    tunnel: [w320] -> w45
    tunnel: [w322] -> w44
    tunnel: w6 -> [w321]
    tunnel: w5 -> [w323]
    tunnel: w45 -> [w330]
    tunnel: [w329] -> w43
    tunnel: w44 -> [w327]
    tunnel: [w328] -> w42
    tunnel: [w340] -> w41
    tunnel: [w341] -> w40
    tunnel: w43 -> [w339]
    tunnel: w42 -> [w338]
    tunnel: w41 -> [w351]
    tunnel: w40 -> [w350]
    tunnel: [w353] -> w39
    tunnel: [w352] -> w38
    tunnel: [w347] -> w37
    tunnel: [w358] -> w15
    tunnel: [w359] -> w16
    tunnel: w39 -> [w359]
    tunnel: w38 -> [w358]
    tunnel: w37 -> [w356]
    frame #0 {
      n123 = call "mDrive Send Command.vi"("error in (no error)"=w311, "Extra"="EM=2", "Command"=T2."Send String", "VISA resource name"=w314) -> ("error out"=w312:errorcluster, "VISA resource name out"=w313:refnum<visa-resource-name>)  [unwired: 3 in, 1 out]
    }
    frame #1 {
      # "Run Current %"
      n124 = property on="Z Run Current %" class="DigNum (strict)"() -> ("Value"=w318:i32)  [unwired: 2 in, 2 out]
      n125 = Number To Decimal String(number=w318) -> (decimal integer string=w319:string)  [unwired: 1 in]
      n126 = call "mDrive Send Command.vi"("error in (no error)"=w323, "Extra"=w319, "Command"=T2."Run Current", "VISA resource name"=w321) -> ("error out"=w322:errorcluster, "VISA resource name out"=w320:refnum<visa-resource-name>)  [unwired: 3 in, 1 out]
    }
    frame #2 {
      # "Holding Current %"
      n127 = property on="Z Run Current %" class="DigNum (strict)"() -> ("Value"=w325:i32)  [unwired: 2 in, 2 out]
      n128 = Number To Decimal String(number=w325) -> (decimal integer string=w326:string)  [unwired: 1 in]
      n129 = call "mDrive Send Command.vi"("error in (no error)"=w327, "Extra"=w326, "Command"=T2."Holding Current", "VISA resource name"=w330) -> ("error out"=w328:errorcluster, "VISA resource name out"=w329:refnum<visa-resource-name>)  [unwired: 3 in, 1 out]
    }
    frame #3 {
      # "Print Velocity Ma"
      # "Velocity Max"
      n130 = property on="Z Velocity SP step/sec" class="DigNum (strict)"() -> ("Value"=w337:i32)  [unwired: 2 in, 2 out]
      n131 = Number To Decimal String(number=w337) -> (decimal integer string=w336:string)  [unwired: 1 in]
      n132 = call "mDrive Send Command.vi"("error in (no error)"=w338, "Extra"=w336, "Command"=T2."Max Velocity", "VISA resource name"=w339) -> ("error out"=w334:errorcluster, "VISA resource name out"=w344:refnum<visa-resource-name>)  [unwired: 3 in, 1 out]
      n133 = call "mDrive Send Command.vi"("error in (no error)"=w334, "Extra"="VM", "Command"=T2."Print Parameter", "VISA resource name"=w344) -> ("error out"=w341:errorcluster, "read buffer"=w342:string, "VISA resource name out"=w340:refnum<visa-resource-name>)  [unwired: 3 in]
      n134 = Decimal String To Number(string=w342, offset=0) -> (number=w335:i32)  [unwired: 1 in, 1 out]
      n135 = property on="Z  velocity PV step/sec" class="DigNum (strict)"("Val(Sgnl)"=w335) -> ()  [unwired: 2 in, 2 out]
    }
    frame #4 {
      # "PRINT POSITION"
      n136 = call "mDrive Send Command.vi"("error in (no error)"=w350, "Extra"="P", "Command"=T2."Print Parameter", "VISA resource name"=w351) -> ("error out"=w352:errorcluster, "read buffer"=w349:string, "VISA resource name out"=w353:refnum<visa-resource-name>)  [unwired: 3 in]
      n137 = Decimal String To Number(string=w349, offset=0) -> (number=w347:i32)  [unwired: 1 in, 1 out]
    }
    frame #5 {
      w354 = 0 ("lower limit")
      w355 = 102400000 ("upper limit")
      n138 = property on="Z Step SP" class="DigNum (strict)"("Val(Sgnl)"=w356) -> ()  [unwired: 2 in, 2 out]
      n139 = property on="Z Step SP" class="DigNum (strict)"("Maximum"=w355) -> ()  [unwired: 2 in, 2 out]
      n140 = property on="Z Step SP" class="DigNum (strict)"("Minimum"=w354) -> ()  [unwired: 2 in, 2 out]
      n141 = In Range and Coerce(upper limit=w355, x=w356, lower limit=w354) -> (In Range?=w357:bool)  [unwired: 1 out]
      n142 = property on="Z in Range" class="Bool (strict)"("Val(Sgnl)"=w357) -> ()  [unwired: 2 in, 2 out]
      "Z MINPOS" <- w354
      "Z MAXPOS" <- w355
    }
  }
  n143 = while {
    tunnel: w89 -> [w375]
    tunnel: w88 -> [w378]
    tunnel: [w379] -> w86
    tunnel: [w377] -> w87
    tunnel: w62 -> [w373]
    tunnel: w61 -> [w372]
    tunnel: [w371] -> w60
    tunnel: [w370] -> w59
    tunnel: w16 -> [w369]
    tunnel: w15 -> [w368]
    tunnel: [w367] -> w14
    tunnel: [w366] -> w13
    tunnel: w12 -> [w365]
    tunnel: w11 -> [w364]
    tunnel: [w363] -> w10
    tunnel: [w362] -> w9
    stop <- w374 stop-if-true
    n144 = property on="Y COM PORT" class="VISAName"() -> ("Value"=w360:refnum<visa-resource-name>)  [unwired: 2 in, 2 out]
    n145 = property on="X COM PORT" class="VISAName"() -> ("Value"=w361:refnum<visa-resource-name>)  [unwired: 2 in, 2 out]
    n146 = flat-sequence {
      frame #0 {
      }
    }
    n147 = flat-sequence {
      frame #0 {
      }
    }
    n148 = flat-sequence {
      frame #0 {
      }
    }
    n149 = flat-sequence {
      frame #0 {
      }
    }
    n150 = flat-sequence {
      frame #0 {
      }
    }
    n151 = event shown="[0] Timeout" {
      selector: _ -> [_ _ _ _ _ _ _ _ _ _ _ _ _ _ _ _ _ _ _ _ _ _ _ _ _]
      dyn-events: _ -> [_ _ _ _ _ _ _ _ _ _ _ _ _ _ _ _ _ _ _ _ _ _ _ _ _]
      timeout: 200 -> [_ _ _ _ _ _ _ _ _ _ _ _ _ _ _ _ _ _ _ _ _ _ _ _ _]
      tunnel: w378 -> [w445 _ _ _ _ _ _ _ _ _ _ _ w1274 _ _ _ _ w1523 _ _ w1619 w1635 w1679 w1756 w2000]
      tunnel: [w444 _ _ _ _ _ _ _ _ _ _ _ w1280 _ _ _ _ w1521 _ _ w1619 w1633 w1681 w1745 w1998] -> w379
      tunnel: w375 -> [_ _ _ _ _ _ _ _ _ _ _ _ w1275 _ _ _ _ w1522 _ _ w1620 w1636 w1680 w1758 w2001]
      tunnel: [w443 _ _ _ _ _ _ _ _ _ _ _ w1281 _ _ _ _ w1518 _ _ w1620 w1634 w1682 w1746 w1999] -> w377
      tunnel: [_ _ _ _ _ _ _ _ _ _ _ _ _ _ _ _ _ _ _ _ TRUE _ _ _ _] -> w374
      tunnel: w373 -> [_ _ _ _ _ _ _ _ _ _ _ _ _ _ _ w1432 w1487 _ _ _ _ w1630 w1672 w1762 w1997]
      tunnel: w372 -> [w420 _ _ _ _ _ _ _ _ _ _ _ _ _ _ w1431 w1486 _ _ _ _ w1629 w1671 w1760 w1996]
      tunnel: [w419 _ _ _ _ _ _ _ _ _ _ _ _ _ _ w1430 w1485 _ _ _ _ w1632 w1670 w1738 w1995] -> w371
      tunnel: [w418 _ _ _ _ _ _ _ _ _ _ _ _ _ _ w1429 w1484 _ _ _ _ w1631 w1669 w1736 w1994] -> w370
      tunnel: w369 -> [w392 _ _ _ _ _ _ _ _ _ _ _ _ w1326 _ _ _ _ w1553 _ _ w1628 w1666 w1754 w1993]
      tunnel: w368 -> [w395 _ _ _ _ _ _ _ _ _ _ _ _ w1325 _ _ _ _ w1552 _ _ w1627 w1665 w1752 w1992]
      tunnel: [w394 _ _ _ _ _ _ _ _ _ _ _ _ w1323 _ _ _ _ w1550 _ _ w1626 w1664 w1744 w1989] -> w367
      tunnel: [w393 _ _ _ _ _ _ _ _ _ _ _ _ w1324 _ _ _ _ w1551 _ _ w1625 w1663 w1743 w1988] -> w366
      tunnel: w365 -> [w391 _ _ _ _ _ _ _ _ _ _ _ _ _ w1379 _ _ _ _ w1587 _ w1624 w1660 w1749 w1991]
      tunnel: w364 -> [w390 _ _ _ _ _ _ _ _ _ _ _ _ _ w1378 _ _ _ _ w1586 _ w1623 w1659 w1747 w1990]
      tunnel: [w389 _ _ _ _ _ _ _ _ _ _ _ _ _ w1376 _ _ _ _ w1585 _ w1622 w1658 w1741 w1987] -> w363
      tunnel: [w388 _ _ _ _ _ _ _ _ _ _ _ _ _ w1377 _ _ _ _ w1584 _ w1621 w1657 w1740 w1986] -> w362
      tunnel: w361 -> [w381 _ _ _ _ _ _ _ _ _ _ _ _ _ _ _ _ _ _ _ _ _ _ _ _]
      tunnel: w360 -> [w380 _ _ _ _ _ _ _ _ _ _ _ _ _ _ _ _ _ _ _ _ _ _ _ _]
      event #0 {
        n152 = event-data() -> ()  [unwired: 1 in, 2 out]
        n153 = flat-sequence {
          tunnel: [w481] -> w406
          tunnel: [w457] -> w405
          tunnel: [w470] -> w404
          tunnel: [w448] -> w403
          tunnel: w391 -> [w447]
          tunnel: w390 -> [w446]
          tunnel: w406 -> [w487]
          tunnel: [w487] -> w402
          tunnel: w405 -> [w486]
          tunnel: [w486] -> w401
          tunnel: w404 -> [w485]
          tunnel: [w485] -> w400
          tunnel: w403 -> [w482]
          tunnel: [w482] -> w399
          tunnel: w402 -> [w494]
          tunnel: [w495] -> w398
          tunnel: w401 -> [w497]
          tunnel: [w496] -> w397
          tunnel: w400 -> [w493]
          tunnel: [w492] -> w396
          tunnel: w399 -> [w492]
          tunnel: w398 -> [w507]
          tunnel: w397 -> [w508]
          tunnel: w396 -> [w510]
          tunnel: [w506] -> w388
          tunnel: [w505] -> w389
          frame #0 {
            w452 = 0.05 ("Delay Time (s)")
            n154 = property on="R Step SP" class="DigNum (strict)"() -> ("Maximum"=w472:dbl)  [unwired: 2 in, 2 out]
            n155 = property on="R Step SP" class="DigNum (strict)"() -> ("Minimum"=w474:dbl)  [unwired: 2 in, 2 out]
            n156 = property on="R steps/rev" class="DigNum (strict)"() -> ("Value"=w468:u32)  [unwired: 2 in, 2 out]
            n157 = property on="R offset deg" class="DigNum (strict)"() -> ("Value"=w464:dbl)  [unwired: 2 in, 2 out]
            n158 = To Long Integer(number=w472) -> (32bit integer=w471:i32)
            n159 = To Long Integer(number=w474) -> (32bit integer=w473:i32)
            n160 = To Double Precision Float(number=w468) -> (double precision float=w469:dbl)
            n161 = call "mDrive Send Command.vi"("error in (no error)"=w446, "Extra"="P", "Command"=T2."Print Parameter", "VISA resource name"=w447) -> ("error out"=w476:errorcluster, "read buffer"=w480:string, "VISA resource name out"=w478:refnum<visa-resource-name>)  [unwired: 3 in]
            n162 = call "Time Delay21"("error in (no error)"=w476, "Delay Time (s)"=w452) -> ("error out"=w475:errorcluster)  [unwired: 9 in]
            n163 = Decimal String To Number(string=w480, offset=0) -> (number=w460:i32)  [unwired: 1 in, 1 out]
            n164 = To Long Integer(number=w460) -> (32bit integer=w462:i32)
            n165 = property on="R Step PV" class="DigNum (strict)"("Val(Sgnl)"=w462) -> ()  [unwired: 2 in, 2 out]
            n166 = call "mDrive Send Command.vi"("error in (no error)"=w475, "Extra"="MV", "Command"=T2."Print Parameter", "VISA resource name"=w478) -> ("error out"=w477:errorcluster, "read buffer"=w458:string, "VISA resource name out"=w481:refnum<visa-resource-name>)  [unwired: 3 in]
            n167 = call "Time Delay20"("error in (no error)"=w477, "Delay Time (s)"=w452) -> ("error out"=w457:errorcluster)  [unwired: 9 in]
            n168 = In Range and Coerce(upper limit=w471, x=w462, lower limit=w473) -> (In Range?=w470:bool)  [unwired: 1 out]
            n169 = To Double Precision Float(number=w462) -> (double precision float=w463:dbl)
            n170 = Decimal String To Number(string=w458, offset=0 ("offset (0)")) -> (number=w451:i32)  [unwired: 1 in, 1 out]
            n171 = property on="R in Range" class="Bool (strict)"("Val(Sgnl)"=w470) -> ()  [unwired: 2 in, 2 out]
            n172 = Divide(x=w463, y=w469) -> (x/y=w467:dbl)
            n173 = Number To Boolean Array(number=w451) -> (Boolean array=w450:bool[])
            n174 = property on="R deg/rev" class="DigNum (strict)"() -> ("Value"=w466:dbl)  [unwired: 2 in, 2 out]
            n175 = Index Array(array=w450, index=0) -> (element=w448:bool)
            n176 = Multiply(x=w467, y=w466) -> (x*y=w465:dbl)
            n177 = property on="R in Motion" class="Bool (strict)"("Val(Sgnl)"=w448) -> ()  [unwired: 2 in, 2 out]
            n178 = Add(x=w465, y=w464) -> (x+y=w461:dbl)
            n179 = property on="R Position deg PV" class="DigNum (strict)"("Val(Sgnl)"=w461) -> ()  [unwired: 2 in, 2 out]
          }
          frame #1 {
            n180 = property on="R Scan" class="Bool (strict)"() -> ("Value"=w483:bool)  [unwired: 2 in, 2 out]
            n181 = Or(x=w482, y=w483) -> (x .or. y?=w484:bool)
            n182 = case shown="True" w484 {
              frame #0 {
                n183 = property on="R Go" class="Bool"("DisabledEnum"=T1."Enabled" ("Disabled")) -> ()  [unwired: 2 in, 2 out]
                n184 = property on="R Scan OK" class="Bool"("DisabledEnum"=T1."Enabled" ("Disabled")) -> ()  [unwired: 2 in, 2 out]
              }
              frame #1 {
                n185 = property on="R Go" class="Bool"("DisabledEnum"=T1."Disabled and Grayed Out" ("Disabled")) -> ()  [unwired: 2 in, 2 out]
                n186 = property on="R Scan OK" class="Bool"("DisabledEnum"=T1."Disabled and Grayed Out" ("Disabled")) -> ()  [unwired: 2 in, 2 out]
              }
            }
          }
          frame #2 {
            n187 = case shown="False" w493 {
              tunnel: w494 -> [w500 w504]
              tunnel: [w501 w504] -> w495
              tunnel: [w502 w503] -> w496
              tunnel: w497 -> [w499 w503]
              frame #0 {
                n188 = call "mDrive Send Command.vi"("error in (no error)"=w499, "Command"=T2."Stop", "VISA resource name"=w500) -> ("error out"=w502:errorcluster, "VISA resource name out"=w501:refnum<visa-resource-name>)  [unwired: 4 in, 1 out]
              }
              frame #1 {
              }
            }
          }
          frame #3 {
            n189 = property on="R Backlash corr" class="Bool (strict)"() -> ("Value"=w511:bool)  [unwired: 2 in, 2 out]
            n190 = Implies(1:w510, 2:w511) -> (0:w509:bool)
            n191 = case shown="False" w509 {
              tunnel: w508 -> [w518 w571]
              tunnel: w507 -> [w517 w572]
              tunnel: [w516 w571] -> w506
              tunnel: [w515 w572] -> w505
              frame #0 {
                # "Backlash"
                n192 = flat-sequence {
                  tunnel: [w533] -> w530
                  tunnel: [w535] -> w529
                  tunnel: [w534] -> w528
                  tunnel: w518 -> [w532]
                  tunnel: w517 -> [w531]
                  tunnel: w530 -> [w543]
                  tunnel: [w543] -> w527
                  tunnel: w529 -> [w542]
                  tunnel: w528 -> [w541]
                  tunnel: [w540] -> w526
                  tunnel: [w539] -> w525
                  tunnel: [w538] -> w514
                  tunnel: w527 -> [w553]
                  tunnel: w526 -> [w552]
                  tunnel: w525 -> [w550]
                  tunnel: [w551] -> w524
                  tunnel: [w550] -> w523
                  tunnel: [w549] -> w520
                  tunnel: [w548] -> w519
                  tunnel: w514 -> [w548]
                  tunnel: w524 -> [w564]
                  tunnel: w523 -> [w557]
                  tunnel: [w564] -> w522
                  tunnel: [w563] -> w521
                  tunnel: w520 -> [w563]
                  tunnel: w519 -> [w559]
                  tunnel: [w558] -> w512
                  tunnel: w522 -> [w568]
                  tunnel: w521 -> [w567]
                  tunnel: [w566] -> w516
                  tunnel: [w565] -> w513
                  tunnel: w512 -> [w565]
                  tunnel: [w570] -> w515
                  tunnel: w513 -> [w570]
                  frame #0 {
                    n193 = property on="R Backlash steps/sec" class="DigNum (strict)"() -> ("Value"=w533:i32)  [unwired: 2 in, 2 out]
                    n194 = Number To Decimal String(number=w533) -> (decimal integer string=w536:string)  [unwired: 1 in]
                    n195 = call "mDrive Send Command.vi"("error in (no error)"=w532, "Extra"=w536, "Command"=T2."Max Velocity", "VISA resource name"=w531) -> ("error out"=w534:errorcluster, "VISA resource name out"=w535:refnum<visa-resource-name>)  [unwired: 3 in, 1 out]
                  }
                  frame #1 {
                    n196 = property on="R Backlash" class="DigNum (strict)"() -> ("Value"=w538:i32)  [unwired: 2 in, 2 out]
                    n197 = Number To Decimal String(number=w538) -> (decimal integer string=w544:string)  [unwired: 1 in]
                    n198 = call "mDrive Send Command.vi"("error in (no error)"=w541, "Extra"=w544, "Command"=T2."Move to Relative Position", "VISA resource name"=w542) -> ("error out"=w540:errorcluster, "VISA resource name out"=w539:refnum<visa-resource-name>)  [unwired: 3 in, 1 out]
                  }
                  frame #2 {
                    n199 = To Double Precision Float(number=w548) -> (double precision float=w546:dbl)
                    n200 = To Double Precision Float(number=w553) -> (double precision float=w555:dbl)
                    n201 = Absolute Value(x=w546) -> (abs(x)=w547:dbl)
                    n202 = Divide(x=w547, y=w555) -> (x/y=w556:dbl)
                    n203 = Add(x=w556, y=0.3) -> (x+y=w549:dbl)
                    n204 = call "Time Delay22"("error in (no error)"=w552, "Delay Time (s)"=w549) -> ("error out"=w551:errorcluster)  [unwired: 9 in]
                  }
                  frame #3 {
                    n205 = Negate(x=w559) -> (-x=w560:i32)
                    n206 = Number To Decimal String(number=w560) -> (decimal integer string=w561:string)  [unwired: 1 in]
                    n207 = call "mDrive Send Command.vi"("Extra"=w561, "Command"=T2."Move to Relative Position", "VISA resource name"=w557) -> ("VISA resource name out"=w558:refnum<visa-resource-name>)  [unwired: 4 in, 2 out]
                  }
                  frame #4 {
                    n208 = call "Time Delay23"("error in (no error)"=w568, "Delay Time (s)"=w567) -> ("error out"=w566:errorcluster)  [unwired: 9 in]
                  }
                  frame #5 {
                    n209 = property on="R Backlash corr" class="Bool (strict)"("Val(Sgnl)"=FALSE ("Value (Signaling)")) -> ()  [unwired: 2 in, 2 out]
                  }
                }
              }
              frame #1 {
              }
            }
          }
        }
        n210 = flat-sequence {
          tunnel: w445 -> [w857]
          tunnel: w380 -> [w856]
          tunnel: [w862] -> w442
          tunnel: [w836] -> w440
          tunnel: [w849] -> w438
          tunnel: [w827] -> w436
          tunnel: w442 -> [w868]
          tunnel: [w868] -> w441
          tunnel: w440 -> [w867]
          tunnel: [w867] -> w439
          tunnel: w438 -> [w866]
          tunnel: [w866] -> w437
          tunnel: w436 -> [w863]
          tunnel: [w863] -> w432
          tunnel: w441 -> [w875]
          tunnel: [w876] -> w435
          tunnel: w439 -> [w878]
          tunnel: [w877] -> w434
          tunnel: w437 -> [w874]
          tunnel: [w873] -> w433
          tunnel: w432 -> [w873]
          tunnel: w435 -> [w888]
          tunnel: w434 -> [w889]
          tunnel: w433 -> [w891]
          tunnel: [w887] -> w444
          tunnel: [w886] -> w443
          frame #0 {
            w831 = 0.05 ("Delay Time (s)")
            n211 = property on="Y Step SP" class="DigNum (strict)"() -> ("Maximum"=w851:dbl)  [unwired: 2 in, 2 out]
            n212 = property on="Y Step SP" class="DigNum (strict)"() -> ("Minimum"=w853:dbl)  [unwired: 2 in, 2 out]
            n213 = property on="Y steps/rev" class="DigNum (strict)"() -> ("Value"=w847:u32)  [unwired: 2 in, 2 out]
            n214 = property on="Y offset mm" class="DigNum (strict)"() -> ("Value"=w843:dbl)  [unwired: 2 in, 2 out]
            n215 = To Long Integer(number=w851) -> (32bit integer=w850:i32)
            n216 = To Long Integer(number=w853) -> (32bit integer=w852:i32)
            n217 = To Double Precision Float(number=w847) -> (double precision float=w848:dbl)
            n218 = call "mDrive Send Command.vi"("error in (no error)"=w857, "Extra"="P", "Command"=T2."Print Parameter", "VISA resource name"=w856) -> ("error out"=w855:errorcluster, "read buffer"=w861:string, "VISA resource name out"=w859:refnum<visa-resource-name>)  [unwired: 3 in]
            n219 = call "Time Delay4"("error in (no error)"=w855, "Delay Time (s)"=w831) -> ("error out"=w854:errorcluster)  [unwired: 9 in]
            n220 = Decimal String To Number(string=w861, offset=0) -> (number=w839:i32)  [unwired: 1 in, 1 out]
            n221 = To Long Integer(number=w839) -> (32bit integer=w841:i32)
            n222 = property on="Y Step PV" class="DigNum (strict)"("Val(Sgnl)"=w841) -> ()  [unwired: 2 in, 2 out]
            n223 = call "mDrive Send Command.vi"("error in (no error)"=w854, "Extra"="MV", "Command"=T2."Print Parameter", "VISA resource name"=w859) -> ("error out"=w858:errorcluster, "read buffer"=w837:string, "VISA resource name out"=w862:refnum<visa-resource-name>)  [unwired: 3 in]
            n224 = call "Time Delay3"("error in (no error)"=w858, "Delay Time (s)"=w831) -> ("error out"=w836:errorcluster)  [unwired: 9 in]
            n225 = In Range and Coerce(upper limit=w850, x=w841, lower limit=w852) -> (In Range?=w849:bool)  [unwired: 1 out]
            n226 = To Double Precision Float(number=w841) -> (double precision float=w842:dbl)
            n227 = Decimal String To Number(string=w837, offset=0 ("offset (0)")) -> (number=w830:i32)  [unwired: 1 in, 1 out]
            n228 = property on="Y in Range" class="Bool (strict)"("Val(Sgnl)"=w849) -> ()  [unwired: 2 in, 2 out]
            n229 = Divide(x=w842, y=w848) -> (x/y=w846:dbl)
            n230 = Number To Boolean Array(number=w830) -> (Boolean array=w829:bool[])
            n231 = property on="Y mm/rev" class="DigNum (strict)"() -> ("Value"=w845:dbl)  [unwired: 2 in, 2 out]
            n232 = Index Array(array=w829, index=0) -> (element=w827:bool)
            n233 = Multiply(x=w846, y=w845) -> (x*y=w844:dbl)
            n234 = property on="Y in Motion" class="Bool (strict)"("Val(Sgnl)"=w827) -> ()  [unwired: 2 in, 2 out]
            n235 = Add(x=w844, y=w843) -> (x+y=w840:dbl)
            n236 = property on="Y Position mm PV" class="DigNum (strict)"("Val(Sgnl)"=w840) -> ()  [unwired: 2 in, 2 out]
          }
          frame #1 {
            n237 = property on="Y Scan" class="Bool (strict)"() -> ("Value"=w864:bool)  [unwired: 2 in, 2 out]
            n238 = Or(x=w863, y=w864) -> (x .or. y?=w865:bool)
            n239 = case shown="True" w865 {
              frame #0 {
                n240 = property on="Y Go" class="Bool"("DisabledEnum"=T1."Enabled" ("Disabled")) -> ()  [unwired: 2 in, 2 out]
                n241 = property on="Y Scan OK" class="Bool"("DisabledEnum"=T1."Enabled" ("Disabled")) -> ()  [unwired: 2 in, 2 out]
              }
              frame #1 {
                n242 = property on="Y Go" class="Bool"("DisabledEnum"=T1."Disabled and Grayed Out" ("Disabled")) -> ()  [unwired: 2 in, 2 out]
                n243 = property on="Y Scan OK" class="Bool"("DisabledEnum"=T1."Disabled and Grayed Out" ("Disabled")) -> ()  [unwired: 2 in, 2 out]
              }
            }
          }
          frame #2 {
            n244 = case shown="False" w874 {
              tunnel: w875 -> [w881 w885]
              tunnel: [w882 w885] -> w876
              tunnel: [w883 w884] -> w877
              tunnel: w878 -> [w880 w884]
              frame #0 {
                n245 = call "mDrive Send Command.vi"("error in (no error)"=w880, "Command"=T2."Stop", "VISA resource name"=w881) -> ("error out"=w883:errorcluster, "VISA resource name out"=w882:refnum<visa-resource-name>)  [unwired: 4 in, 1 out]
              }
              frame #1 {
              }
            }
          }
          frame #3 {
            n246 = property on="Y Backlash corr" class="Bool (strict)"() -> ("Value"=w892:bool)  [unwired: 2 in, 2 out]
            n247 = Implies(1:w891, 2:w892) -> (0:w890:bool)
            n248 = case shown="False" w890 {
              tunnel: w889 -> [w899 w952]
              tunnel: w888 -> [w898 w953]
              tunnel: [w897 w952] -> w887
              tunnel: [w896 w953] -> w886
              frame #0 {
                # "Backlash"
                n249 = flat-sequence {
                  tunnel: [w914] -> w911
                  tunnel: [w916] -> w910
                  tunnel: [w915] -> w909
                  tunnel: w899 -> [w913]
                  tunnel: w898 -> [w912]
                  tunnel: w911 -> [w924]
                  tunnel: [w924] -> w908
                  tunnel: w910 -> [w923]
                  tunnel: w909 -> [w922]
                  tunnel: [w921] -> w907
                  tunnel: [w920] -> w906
                  tunnel: [w919] -> w895
                  tunnel: w908 -> [w934]
                  tunnel: w907 -> [w933]
                  tunnel: w906 -> [w931]
                  tunnel: [w932] -> w905
                  tunnel: [w931] -> w904
                  tunnel: [w930] -> w901
                  tunnel: [w929] -> w900
                  tunnel: w895 -> [w929]
                  tunnel: w905 -> [w945]
                  tunnel: w904 -> [w938]
                  tunnel: [w945] -> w903
                  tunnel: [w944] -> w902
                  tunnel: w901 -> [w944]
                  tunnel: w900 -> [w940]
                  tunnel: [w939] -> w893
                  tunnel: w903 -> [w949]
                  tunnel: w902 -> [w948]
                  tunnel: [w947] -> w897
                  tunnel: [w946] -> w894
                  tunnel: w893 -> [w946]
                  tunnel: [w951] -> w896
                  tunnel: w894 -> [w951]
                  frame #0 {
                    n250 = property on="Y Backlash steps/sec" class="DigNum (strict)"() -> ("Value"=w914:i32)  [unwired: 2 in, 2 out]
                    n251 = Number To Decimal String(number=w914) -> (decimal integer string=w917:string)  [unwired: 1 in]
                    n252 = call "mDrive Send Command.vi"("error in (no error)"=w913, "Extra"=w917, "Command"=T2."Max Velocity", "VISA resource name"=w912) -> ("error out"=w915:errorcluster, "VISA resource name out"=w916:refnum<visa-resource-name>)  [unwired: 3 in, 1 out]
                  }
                  frame #1 {
                    n253 = property on="Y Backlash" class="DigNum (strict)"() -> ("Value"=w919:i32)  [unwired: 2 in, 2 out]
                    n254 = Number To Decimal String(number=w919) -> (decimal integer string=w925:string)  [unwired: 1 in]
                    n255 = call "mDrive Send Command.vi"("error in (no error)"=w922, "Extra"=w925, "Command"=T2."Move to Relative Position", "VISA resource name"=w923) -> ("error out"=w921:errorcluster, "VISA resource name out"=w920:refnum<visa-resource-name>)  [unwired: 3 in, 1 out]
                  }
                  frame #2 {
                    n256 = To Double Precision Float(number=w929) -> (double precision float=w927:dbl)
                    n257 = To Double Precision Float(number=w934) -> (double precision float=w936:dbl)
                    n258 = Absolute Value(x=w927) -> (abs(x)=w928:dbl)
                    n259 = Divide(x=w928, y=w936) -> (x/y=w937:dbl)
                    n260 = Add(x=w937, y=0.3) -> (x+y=w930:dbl)
                    n261 = call "Time Delay8"("error in (no error)"=w933, "Delay Time (s)"=w930) -> ("error out"=w932:errorcluster)  [unwired: 9 in]
                  }
                  frame #3 {
                    n262 = Negate(x=w940) -> (-x=w941:i32)
                    n263 = Number To Decimal String(number=w941) -> (decimal integer string=w942:string)  [unwired: 1 in]
                    n264 = call "mDrive Send Command.vi"("Extra"=w942, "Command"=T2."Move to Relative Position", "VISA resource name"=w938) -> ("VISA resource name out"=w939:refnum<visa-resource-name>)  [unwired: 4 in, 2 out]
                  }
                  frame #4 {
                    n265 = call "Time Delay2"("error in (no error)"=w949, "Delay Time (s)"=w948) -> ("error out"=w947:errorcluster)  [unwired: 9 in]
                  }
                  frame #5 {
                    n266 = property on="Y Backlash corr" class="Bool (strict)"("Val(Sgnl)"=FALSE ("Value (Signaling)")) -> ()  [unwired: 2 in, 2 out]
                  }
                }
              }
              frame #1 {
              }
            }
          }
        }
        n267 = flat-sequence {
          tunnel: [w608] -> w417
          tunnel: [w584] -> w416
          tunnel: [w597] -> w415
          tunnel: [w575] -> w414
          tunnel: w392 -> [w574]
          tunnel: w395 -> [w573]
          tunnel: w417 -> [w614]
          tunnel: [w614] -> w413
          tunnel: w416 -> [w613]
          tunnel: [w613] -> w412
          tunnel: w415 -> [w612]
          tunnel: [w612] -> w411
          tunnel: w414 -> [w609]
          tunnel: [w609] -> w410
          tunnel: w413 -> [w621]
          tunnel: [w622] -> w409
          tunnel: w412 -> [w624]
          tunnel: [w623] -> w408
          tunnel: w411 -> [w620]
          tunnel: [w619] -> w407
          tunnel: w410 -> [w619]
          tunnel: w409 -> [w634]
          tunnel: w408 -> [w635]
          tunnel: w407 -> [w637]
          tunnel: [w633] -> w393
          tunnel: [w632] -> w394
          frame #0 {
            w579 = 0.05 ("Delay Time (s)")
            n268 = property on="Z Step SP" class="DigNum (strict)"() -> ("Maximum"=w599:dbl)  [unwired: 2 in, 2 out]
            n269 = property on="Z Step SP" class="DigNum (strict)"() -> ("Minimum"=w601:dbl)  [unwired: 2 in, 2 out]
            n270 = property on="Z steps/rev" class="DigNum (strict)"() -> ("Value"=w595:u32)  [unwired: 2 in, 2 out]
            n271 = property on="Z offset mm" class="DigNum (strict)"() -> ("Value"=w591:dbl)  [unwired: 2 in, 2 out]
            n272 = To Long Integer(number=w599) -> (32bit integer=w598:i32)
            n273 = To Long Integer(number=w601) -> (32bit integer=w600:i32)
            n274 = To Double Precision Float(number=w595) -> (double precision float=w596:dbl)
            n275 = call "mDrive Send Command.vi"("error in (no error)"=w573, "Extra"="P", "Command"=T2."Print Parameter", "VISA resource name"=w574) -> ("error out"=w603:errorcluster, "read buffer"=w607:string, "VISA resource name out"=w605:refnum<visa-resource-name>)  [unwired: 3 in]
            n276 = call "Time Delay17"("error in (no error)"=w603, "Delay Time (s)"=w579) -> ("error out"=w602:errorcluster)  [unwired: 9 in]
            n277 = Decimal String To Number(string=w607, offset=0) -> (number=w587:i32)  [unwired: 1 in, 1 out]
            n278 = To Long Integer(number=w587) -> (32bit integer=w589:i32)
            n279 = property on="Z Step PV" class="DigNum (strict)"("Val(Sgnl)"=w589) -> ()  [unwired: 2 in, 2 out]
            n280 = call "mDrive Send Command.vi"("error in (no error)"=w602, "Extra"="MV", "Command"=T2."Print Parameter", "VISA resource name"=w605) -> ("error out"=w604:errorcluster, "read buffer"=w585:string, "VISA resource name out"=w608:refnum<visa-resource-name>)  [unwired: 3 in]
            n281 = call "Time Delay16"("error in (no error)"=w604, "Delay Time (s)"=w579) -> ("error out"=w584:errorcluster)  [unwired: 9 in]
            n282 = In Range and Coerce(upper limit=w598, x=w589, lower limit=w600) -> (In Range?=w597:bool)  [unwired: 1 out]
            n283 = To Double Precision Float(number=w589) -> (double precision float=w590:dbl)
            n284 = Decimal String To Number(string=w585, offset=0 ("offset (0)")) -> (number=w578:i32)  [unwired: 1 in, 1 out]
            n285 = property on="Z in Range" class="Bool (strict)"("Val(Sgnl)"=w597) -> ()  [unwired: 2 in, 2 out]
            n286 = Divide(x=w590, y=w596) -> (x/y=w594:dbl)
            n287 = Number To Boolean Array(number=w578) -> (Boolean array=w577:bool[])
            n288 = property on="Z mm/rev" class="DigNum (strict)"() -> ("Value"=w593:dbl)  [unwired: 2 in, 2 out]
            n289 = Index Array(array=w577, index=0) -> (element=w575:bool)
            n290 = Multiply(x=w594, y=w593) -> (x*y=w592:dbl)
            n291 = property on="Z in Motion" class="Bool (strict)"("Val(Sgnl)"=w575) -> ()  [unwired: 2 in, 2 out]
            n292 = Add(x=w592, y=w591) -> (x+y=w588:dbl)
            n293 = property on="Z Position mm PV" class="DigNum (strict)"("Val(Sgnl)"=w588) -> ()  [unwired: 2 in, 2 out]
          }
          frame #1 {
            n294 = property on="Z Scan" class="Bool (strict)"() -> ("Value"=w610:bool)  [unwired: 2 in, 2 out]
            n295 = Or(x=w609, y=w610) -> (x .or. y?=w611:bool)
            n296 = case shown="True" w611 {
              frame #0 {
                n297 = property on="Z Go" class="Bool"("DisabledEnum"=T1."Enabled" ("Disabled")) -> ()  [unwired: 2 in, 2 out]
                n298 = property on="Z Scan OK" class="Bool"("DisabledEnum"=T1."Enabled" ("Disabled")) -> ()  [unwired: 2 in, 2 out]
              }
              frame #1 {
                n299 = property on="Z Go" class="Bool"("DisabledEnum"=T1."Disabled and Grayed Out" ("Disabled")) -> ()  [unwired: 2 in, 2 out]
                n300 = property on="Z Scan OK" class="Bool"("DisabledEnum"=T1."Disabled and Grayed Out" ("Disabled")) -> ()  [unwired: 2 in, 2 out]
              }
            }
          }
          frame #2 {
            n301 = case shown="False" w620 {
              tunnel: w621 -> [w627 w631]
              tunnel: [w628 w631] -> w622
              tunnel: [w629 w630] -> w623
              tunnel: w624 -> [w626 w630]
              frame #0 {
                n302 = call "mDrive Send Command.vi"("error in (no error)"=w626, "Command"=T2."Stop", "VISA resource name"=w627) -> ("error out"=w629:errorcluster, "VISA resource name out"=w628:refnum<visa-resource-name>)  [unwired: 4 in, 1 out]
              }
              frame #1 {
              }
            }
          }
          frame #3 {
            n303 = property on="Z Backlash corr" class="Bool (strict)"() -> ("Value"=w638:bool)  [unwired: 2 in, 2 out]
            n304 = Implies(1:w637, 2:w638) -> (0:w636:bool)
            n305 = case shown="False" w636 {
              tunnel: w635 -> [w645 w698]
              tunnel: w634 -> [w644 w699]
              tunnel: [w643 w698] -> w633
              tunnel: [w642 w699] -> w632
              frame #0 {
                # "Backlash"
                n306 = flat-sequence {
                  tunnel: [w660] -> w657
                  tunnel: [w662] -> w656
                  tunnel: [w661] -> w655
                  tunnel: w645 -> [w659]
                  tunnel: w644 -> [w658]
                  tunnel: w657 -> [w670]
                  tunnel: [w670] -> w654
                  tunnel: w656 -> [w669]
                  tunnel: w655 -> [w668]
                  tunnel: [w667] -> w653
                  tunnel: [w666] -> w652
                  tunnel: [w665] -> w641
                  tunnel: w654 -> [w680]
                  tunnel: w653 -> [w679]
                  tunnel: w652 -> [w677]
                  tunnel: [w678] -> w651
                  tunnel: [w677] -> w650
                  tunnel: [w676] -> w647
                  tunnel: [w675] -> w646
                  tunnel: w641 -> [w675]
                  tunnel: w651 -> [w691]
                  tunnel: w650 -> [w684]
                  tunnel: [w691] -> w649
                  tunnel: [w690] -> w648
                  tunnel: w647 -> [w690]
                  tunnel: w646 -> [w686]
                  tunnel: [w685] -> w639
                  tunnel: w649 -> [w695]
                  tunnel: w648 -> [w694]
                  tunnel: [w693] -> w643
                  tunnel: [w692] -> w640
                  tunnel: w639 -> [w692]
                  tunnel: [w697] -> w642
                  tunnel: w640 -> [w697]
                  frame #0 {
                    n307 = property on="Z Backlash steps/sec" class="DigNum (strict)"() -> ("Value"=w660:i32)  [unwired: 2 in, 2 out]
                    n308 = Number To Decimal String(number=w660) -> (decimal integer string=w663:string)  [unwired: 1 in]
                    n309 = call "mDrive Send Command.vi"("error in (no error)"=w659, "Extra"=w663, "Command"=T2."Max Velocity", "VISA resource name"=w658) -> ("error out"=w661:errorcluster, "VISA resource name out"=w662:refnum<visa-resource-name>)  [unwired: 3 in, 1 out]
                  }
                  frame #1 {
                    n310 = property on="Z Backlash" class="DigNum (strict)"() -> ("Value"=w665:i32)  [unwired: 2 in, 2 out]
                    n311 = Number To Decimal String(number=w665) -> (decimal integer string=w671:string)  [unwired: 1 in]
                    n312 = call "mDrive Send Command.vi"("error in (no error)"=w668, "Extra"=w671, "Command"=T2."Move to Relative Position", "VISA resource name"=w669) -> ("error out"=w667:errorcluster, "VISA resource name out"=w666:refnum<visa-resource-name>)  [unwired: 3 in, 1 out]
                  }
                  frame #2 {
                    n313 = To Double Precision Float(number=w675) -> (double precision float=w673:dbl)
                    n314 = To Double Precision Float(number=w680) -> (double precision float=w682:dbl)
                    n315 = Absolute Value(x=w673) -> (abs(x)=w674:dbl)
                    n316 = Divide(x=w674, y=w682) -> (x/y=w683:dbl)
                    n317 = Add(x=w683, y=0.5) -> (x+y=w676:dbl)
                    n318 = call "Time Delay18"("error in (no error)"=w679, "Delay Time (s)"=w676) -> ("error out"=w678:errorcluster)  [unwired: 9 in]
                  }
                  frame #3 {
                    n319 = Negate(x=w686) -> (-x=w687:i32)
                    n320 = Number To Decimal String(number=w687) -> (decimal integer string=w688:string)  [unwired: 1 in]
                    n321 = call "mDrive Send Command.vi"("Extra"=w688, "Command"=T2."Move to Relative Position", "VISA resource name"=w684) -> ("VISA resource name out"=w685:refnum<visa-resource-name>)  [unwired: 4 in, 2 out]
                  }
                  frame #4 {
                    n322 = call "Time Delay19"("error in (no error)"=w695, "Delay Time (s)"=w694) -> ("error out"=w693:errorcluster)  [unwired: 9 in]
                  }
                  frame #5 {
                    n323 = property on="Z Backlash corr" class="Bool (strict)"("Val(Sgnl)"=FALSE ("Value (Signaling)")) -> ()  [unwired: 2 in, 2 out]
                  }
                }
              }
              frame #1 {
              }
            }
          }
        }
        n324 = flat-sequence {
          tunnel: [w735] -> w431
          tunnel: [w711] -> w430
          tunnel: [w724] -> w429
          tunnel: [w702] -> w428
          tunnel: w381 -> [w701]
          tunnel: w420 -> [w700]
          tunnel: w431 -> [w741]
          tunnel: [w741] -> w427
          tunnel: w430 -> [w740]
          tunnel: [w740] -> w426
          tunnel: w429 -> [w739]
          tunnel: [w739] -> w425
          tunnel: w428 -> [w736]
          tunnel: [w736] -> w424
          tunnel: w427 -> [w748]
          tunnel: [w749] -> w423
          tunnel: w426 -> [w751]
          tunnel: [w750] -> w422
          tunnel: w425 -> [w747]
          tunnel: [w746] -> w421
          tunnel: w424 -> [w746]
          tunnel: w423 -> [w761]
          tunnel: w422 -> [w762]
          tunnel: w421 -> [w764]
          tunnel: [w760] -> w418
          tunnel: [w759] -> w419
          frame #0 {
            w706 = 0.05 ("Delay Time (s)")
            n325 = property on="X Step SP" class="DigNum (strict)"() -> ("Maximum"=w726:dbl)  [unwired: 2 in, 2 out]
            n326 = property on="X Step SP" class="DigNum (strict)"() -> ("Minimum"=w728:dbl)  [unwired: 2 in, 2 out]
            n327 = property on="X steps/rev" class="DigNum (strict)"() -> ("Value"=w722:u32)  [unwired: 2 in, 2 out]
            n328 = property on="X offset mm" class="DigNum (strict)"() -> ("Value"=w718:dbl)  [unwired: 2 in, 2 out]
            n329 = To Long Integer(number=w726) -> (32bit integer=w725:i32)
            n330 = To Long Integer(number=w728) -> (32bit integer=w727:i32)
            n331 = To Double Precision Float(number=w722) -> (double precision float=w723:dbl)
            n332 = call "mDrive Send Command.vi"("error in (no error)"=w700, "Extra"="P", "Command"=T2."Print Parameter", "VISA resource name"=w701) -> ("error out"=w730:errorcluster, "read buffer"=w734:string, "VISA resource name out"=w732:refnum<visa-resource-name>)  [unwired: 3 in]
            n333 = call "Time Delay12"("error in (no error)"=w730, "Delay Time (s)"=w706) -> ("error out"=w729:errorcluster)  [unwired: 9 in]
            n334 = Decimal String To Number(string=w734, offset=0) -> (number=w714:i32)  [unwired: 1 in, 1 out]
            n335 = To Long Integer(number=w714) -> (32bit integer=w716:i32)
            n336 = property on="X Step PV" class="DigNum (strict)"("Val(Sgnl)"=w716) -> ()  [unwired: 2 in, 2 out]
            n337 = call "mDrive Send Command.vi"("error in (no error)"=w729, "Extra"="MV", "Command"=T2."Print Parameter", "VISA resource name"=w732) -> ("error out"=w731:errorcluster, "read buffer"=w712:string, "VISA resource name out"=w735:refnum<visa-resource-name>)  [unwired: 3 in]
            n338 = call "Time Delay11"("error in (no error)"=w731, "Delay Time (s)"=w706) -> ("error out"=w711:errorcluster)  [unwired: 9 in]
            n339 = In Range and Coerce(upper limit=w725, x=w716, lower limit=w727) -> (In Range?=w724:bool)  [unwired: 1 out]
            n340 = To Double Precision Float(number=w716) -> (double precision float=w717:dbl)
            n341 = Decimal String To Number(string=w712, offset=0 ("offset (0)")) -> (number=w705:i32)  [unwired: 1 in, 1 out]
            n342 = Divide(x=w717, y=w723) -> (x/y=w721:dbl)
            n343 = Number To Boolean Array(number=w705) -> (Boolean array=w704:bool[])
            n344 = property on="X  in Range" class="Bool (strict)"("Val(Sgnl)"=w724) -> ()  [unwired: 2 in, 2 out]
            n345 = property on="X mm/rev" class="DigNum (strict)"() -> ("Value"=w720:dbl)  [unwired: 2 in, 2 out]
            n346 = Index Array(array=w704, index=0) -> (element=w702:bool)
            n347 = Multiply(x=w721, y=w720) -> (x*y=w719:dbl)
            n348 = property on="X  in Motion" class="Bool (strict)"("Val(Sgnl)"=w702) -> ()  [unwired: 2 in, 2 out]
            n349 = Add(x=w719, y=w718) -> (x+y=w715:dbl)
            n350 = property on="X Position mm PV" class="DigNum (strict)"("Val(Sgnl)"=w715) -> ()  [unwired: 2 in, 2 out]
          }
          frame #1 {
            n351 = property on="X Scan" class="Bool (strict)"() -> ("Value"=w737:bool)  [unwired: 2 in, 2 out]
            n352 = Or(x=w736, y=w737) -> (x .or. y?=w738:bool)
            n353 = case shown="True" w738 {
              frame #0 {
                n354 = property on="X Go" class="Bool"("DisabledEnum"=T1."Enabled" ("Disabled")) -> ()  [unwired: 2 in, 2 out]
                n355 = property on="X Scan OK" class="Bool"("DisabledEnum"=T1."Enabled" ("Disabled")) -> ()  [unwired: 2 in, 2 out]
              }
              frame #1 {
                n356 = property on="X Go" class="Bool"("DisabledEnum"=T1."Disabled and Grayed Out" ("Disabled")) -> ()  [unwired: 2 in, 2 out]
                n357 = property on="X Scan OK" class="Bool"("DisabledEnum"=T1."Disabled and Grayed Out" ("Disabled")) -> ()  [unwired: 2 in, 2 out]
              }
            }
          }
          frame #2 {
            n358 = case shown="False" w747 {
              tunnel: w748 -> [w754 w758]
              tunnel: [w755 w758] -> w749
              tunnel: [w756 w757] -> w750
              tunnel: w751 -> [w753 w757]
              frame #0 {
                n359 = call "mDrive Send Command.vi"("error in (no error)"=w753, "Command"=T2."Stop", "VISA resource name"=w754) -> ("error out"=w756:errorcluster, "VISA resource name out"=w755:refnum<visa-resource-name>)  [unwired: 4 in, 1 out]
              }
              frame #1 {
              }
            }
          }
          frame #3 {
            n360 = property on="X Backlash corr" class="Bool (strict)"() -> ("Value"=w765:bool)  [unwired: 2 in, 2 out]
            n361 = Implies(1:w764, 2:w765) -> (0:w763:bool)
            n362 = case shown="False" w763 {
              tunnel: w762 -> [w772 w825]
              tunnel: w761 -> [w771 w826]
              tunnel: [w770 w825] -> w760
              tunnel: [w769 w826] -> w759
              frame #0 {
                # "Backlash"
                n363 = flat-sequence {
                  tunnel: [w787] -> w784
                  tunnel: [w789] -> w783
                  tunnel: [w788] -> w782
                  tunnel: w772 -> [w786]
                  tunnel: w771 -> [w785]
                  tunnel: w784 -> [w797]
                  tunnel: [w797] -> w781
                  tunnel: w783 -> [w796]
                  tunnel: w782 -> [w795]
                  tunnel: [w794] -> w780
                  tunnel: [w793] -> w779
                  tunnel: [w792] -> w768
                  tunnel: w781 -> [w807]
                  tunnel: w780 -> [w806]
                  tunnel: w779 -> [w804]
                  tunnel: [w805] -> w778
                  tunnel: [w804] -> w777
                  tunnel: [w803] -> w774
                  tunnel: [w802] -> w773
                  tunnel: w768 -> [w802]
                  tunnel: w778 -> [w818]
                  tunnel: w777 -> [w811]
                  tunnel: [w818] -> w776
                  tunnel: [w817] -> w775
                  tunnel: w774 -> [w817]
                  tunnel: w773 -> [w813]
                  tunnel: [w812] -> w766
                  tunnel: w776 -> [w822]
                  tunnel: w775 -> [w821]
                  tunnel: [w820] -> w770
                  tunnel: [w819] -> w767
                  tunnel: w766 -> [w819]
                  tunnel: [w824] -> w769
                  tunnel: w767 -> [w824]
                  frame #0 {
                    n364 = property on="X Backlash steps/sec" class="DigNum (strict)"() -> ("Value"=w787:i32)  [unwired: 2 in, 2 out]
                    n365 = Number To Decimal String(number=w787) -> (decimal integer string=w790:string)  [unwired: 1 in]
                    n366 = call "mDrive Send Command.vi"("error in (no error)"=w786, "Extra"=w790, "Command"=T2."Max Velocity", "VISA resource name"=w785) -> ("error out"=w788:errorcluster, "VISA resource name out"=w789:refnum<visa-resource-name>)  [unwired: 3 in, 1 out]
                  }
                  frame #1 {
                    n367 = property on="X Backlash" class="DigNum (strict)"() -> ("Value"=w792:i32)  [unwired: 2 in, 2 out]
                    n368 = Number To Decimal String(number=w792) -> (decimal integer string=w798:string)  [unwired: 1 in]
                    n369 = call "mDrive Send Command.vi"("error in (no error)"=w795, "Extra"=w798, "Command"=T2."Move to Relative Position", "VISA resource name"=w796) -> ("error out"=w794:errorcluster, "VISA resource name out"=w793:refnum<visa-resource-name>)  [unwired: 3 in, 1 out]
                  }
                  frame #2 {
                    n370 = To Double Precision Float(number=w802) -> (double precision float=w800:dbl)
                    n371 = To Double Precision Float(number=w807) -> (double precision float=w809:dbl)
                    n372 = Absolute Value(x=w800) -> (abs(x)=w801:dbl)
                    n373 = Divide(x=w801, y=w809) -> (x/y=w810:dbl)
                    n374 = Add(x=w810, y=0.3) -> (x+y=w803:dbl)
                    n375 = call "Time Delay13"("error in (no error)"=w806, "Delay Time (s)"=w803) -> ("error out"=w805:errorcluster)  [unwired: 9 in]
                  }
                  frame #3 {
                    n376 = Negate(x=w813) -> (-x=w814:i32)
                    n377 = Number To Decimal String(number=w814) -> (decimal integer string=w815:string)  [unwired: 1 in]
                    n378 = call "mDrive Send Command.vi"("Extra"=w815, "Command"=T2."Move to Relative Position", "VISA resource name"=w811) -> ("VISA resource name out"=w812:refnum<visa-resource-name>)  [unwired: 4 in, 2 out]
                  }
                  frame #4 {
                    n379 = call "Time Delay14"("error in (no error)"=w822, "Delay Time (s)"=w821) -> ("error out"=w820:errorcluster)  [unwired: 9 in]
                  }
                  frame #5 {
                    n380 = property on="X Backlash corr" class="Bool (strict)"("Val(Sgnl)"=FALSE ("Value (Signaling)")) -> ()  [unwired: 2 in, 2 out]
                  }
                }
              }
              frame #1 {
              }
            }
          }
        }
        n381 = property on="X Position mm PV" class="DigNum (strict)"() -> ("Value"=w383:dbl)  [unwired: 2 in, 2 out]
        n382 = property on="Y Position mm PV" class="DigNum (strict)"() -> ("Value"=w385:dbl)  [unwired: 2 in, 2 out]
        n383 = property on="Z Position mm PV" class="DigNum (strict)"() -> ("Value"=w382:dbl)  [unwired: 2 in, 2 out]
        n384 = property on="R Position deg PV" class="DigNum (strict)"() -> ("Value"=w384:dbl)  [unwired: 2 in, 2 out]
        n385 = call "Build XY Graph"("Y Input"=w385, "X Input"=w383) -> ("XY Graph"=→"XY Graph":cluster{"Y":dbl[], "Y":dbl[]}[])  [unwired: 8 in, 1 out]
        n386 = call "Build XY Graph2"("Y Input"=w384, "X Input"=w382) -> ("XY Graph"=→"XY Graph 2":cluster{"Y":dbl[], "Y":dbl[]}[])  [unwired: 8 in, 1 out]
      }
      event #1 {
        n387 = event-data() -> ()  [unwired: 1 in, 5 out]
        n388 = property on="Z steps/rev" class="DigNum (strict)"() -> ("Value"=w965:u32)  [unwired: 2 in, 2 out]
        n389 = property on="R steps/rev" class="DigNum (strict)"() -> ("Value"=w956:u32)  [unwired: 2 in, 2 out]
        n390 = property on="X steps/rev" class="DigNum (strict)"() -> ("Value"=w974:u32)  [unwired: 2 in, 2 out]
        n391 = property on="Y steps/rev" class="DigNum (strict)"() -> ("Value"=w983:u32)  [unwired: 2 in, 2 out]
        n392 = property on="Z offset mm" class="DigNum (strict)"() -> ("Value"=w963:dbl)  [unwired: 2 in, 2 out]
        n393 = property on="R offset deg" class="DigNum (strict)"() -> ("Value"=w954:dbl)  [unwired: 2 in, 2 out]
        n394 = property on="X offset mm" class="DigNum (strict)"() -> ("Value"=w972:dbl)  [unwired: 2 in, 2 out]
        n395 = property on="Y offset mm" class="DigNum (strict)"() -> ("Value"=w981:dbl)  [unwired: 2 in, 2 out]
        n396 = property on="Reset R Position deg" class="DigNum (strict)"() -> ("Value"=w962:dbl)  [unwired: 2 in, 2 out]
        n397 = property on="Reset Z Position mm" class="DigNum (strict)"() -> ("Value"=w971:dbl)  [unwired: 2 in, 2 out]
        n398 = property on="Reset X Position mm" class="DigNum (strict)"() -> ("Value"=w980:dbl)  [unwired: 2 in, 2 out]
        n399 = property on="Reset Y Position mm" class="DigNum (strict)"() -> ("Value"=w989:dbl)  [unwired: 2 in, 2 out]
        n400 = To Double Precision Float(number=w983) -> (double precision float=w986:dbl)
        n401 = Subtract(x=w971, y=w963) -> (x-y=w970:dbl)
        n402 = Subtract(x=w962, y=w954) -> (x-y=w961:dbl)
        n403 = Subtract(x=w980, y=w972) -> (x-y=w979:dbl)
        n404 = Subtract(x=w989, y=w981) -> (x-y=w988:dbl)
        n405 = property on="R deg/rev" class="DigNum (strict)"() -> ("Value"=w955:dbl)  [unwired: 2 in, 2 out]
        n406 = property on="Z mm/rev" class="DigNum (strict)"() -> ("Value"=w964:dbl)  [unwired: 2 in, 2 out]
        n407 = property on="X mm/rev" class="DigNum (strict)"() -> ("Value"=w973:dbl)  [unwired: 2 in, 2 out]
        n408 = property on="Y mm/rev" class="DigNum (strict)"() -> ("Value"=w982:dbl)  [unwired: 2 in, 2 out]
        n409 = Divide(x=w988, y=w982) -> (x/y=w987:dbl)
        n410 = Divide(x=w970, y=w964) -> (x/y=w969:dbl)
        n411 = Divide(x=w961, y=w955) -> (x/y=w960:dbl)
        n412 = Divide(x=w979, y=w973) -> (x/y=w978:dbl)
        n413 = To Double Precision Float(number=w965) -> (double precision float=w968:dbl)
        n414 = To Double Precision Float(number=w956) -> (double precision float=w959:dbl)
        n415 = To Double Precision Float(number=w974) -> (double precision float=w977:dbl)
        n416 = Multiply(x=w969, y=w968) -> (x*y=w967:dbl)
        n417 = Multiply(x=w960, y=w959) -> (x*y=w958:dbl)
        n418 = Multiply(x=w978, y=w977) -> (x*y=w976:dbl)
        n419 = Multiply(x=w987, y=w986) -> (x*y=w985:dbl)
        n420 = To Long Integer(number=w967) -> (32bit integer=w966:i32)
        n421 = To Long Integer(number=w958) -> (32bit integer=w957:i32)
        n422 = To Long Integer(number=w976) -> (32bit integer=w975:i32)
        n423 = To Long Integer(number=w985) -> (32bit integer=w984:i32)
        n424 = property on="Reset Z Motor Steps" class="DigNum (strict)"("Val(Sgnl)"=w966) -> ()  [unwired: 2 in, 2 out]
        n425 = property on="Reset R Motor Steps" class="DigNum (strict)"("Val(Sgnl)"=w957) -> ()  [unwired: 2 in, 2 out]
        n426 = property on="Reset X Motor Steps" class="DigNum (strict)"("Val(Sgnl)"=w975) -> ()  [unwired: 2 in, 2 out]
        n427 = property on="Reset Y Motor Steps" class="DigNum (strict)"("Val(Sgnl)"=w984) -> ()  [unwired: 2 in, 2 out]
      }
      event #2 {
        n428 = event-data() -> ()  [unwired: 1 in, 5 out]
        n429 = property on="R Step SP" class="DigNum (strict)"() -> ("Value"=w998:i32)  [unwired: 2 in, 2 out]
        n430 = property on="X Step SP" class="DigNum (strict)"() -> ("Value"=w1014:i32)  [unwired: 2 in, 2 out]
        n431 = property on="Z Step SP" class="DigNum (strict)"() -> ("Value"=w1006:i32)  [unwired: 2 in, 2 out]
        n432 = property on="Y Step SP" class="DigNum (strict)"() -> ("Value"=w1022:i32)  [unwired: 2 in, 2 out]
        n433 = property on="R steps/rev" class="DigNum (strict)"() -> ("Value"=w1027:u32)  [unwired: 2 in, 2 out]
        n434 = property on="R steps/rev" class="DigNum (strict)"() -> ("Value"=w996:u32)  [unwired: 2 in, 2 out]
        n435 = property on="X steps/rev" class="DigNum (strict)"() -> ("Value"=w1039:u32)  [unwired: 2 in, 2 out]
        n436 = property on="X steps/rev" class="DigNum (strict)"() -> ("Value"=w1012:u32)  [unwired: 2 in, 2 out]
        n437 = property on="Z steps/rev" class="DigNum (strict)"() -> ("Value"=w1033:u32)  [unwired: 2 in, 2 out]
        n438 = property on="Z steps/rev" class="DigNum (strict)"() -> ("Value"=w1004:u32)  [unwired: 2 in, 2 out]
        n439 = property on="Y steps/rev" class="DigNum (strict)"() -> ("Value"=w1045:u32)  [unwired: 2 in, 2 out]
        n440 = property on="Y steps/rev" class="DigNum (strict)"() -> ("Value"=w1020:u32)  [unwired: 2 in, 2 out]
        n441 = property on="R offset deg" class="DigNum (strict)"() -> ("Value"=w995:dbl)  [unwired: 2 in, 2 out]
        n442 = property on="X offset mm" class="DigNum (strict)"() -> ("Value"=w1011:dbl)  [unwired: 2 in, 2 out]
        n443 = property on="Z offset mm" class="DigNum (strict)"() -> ("Value"=w1003:dbl)  [unwired: 2 in, 2 out]
        n444 = property on="Y offset mm" class="DigNum (strict)"() -> ("Value"=w1019:dbl)  [unwired: 2 in, 2 out]
        n445 = property on="R Velocity SP step/sec" class="DigNum (strict)"() -> ("Value"=w1029:i32)  [unwired: 2 in, 2 out]
        n446 = property on="X Velocity SP step/sec" class="DigNum (strict)"() -> ("Value"=w1041:i32)  [unwired: 2 in, 2 out]
        n447 = property on="Z Velocity SP step/sec" class="DigNum (strict)"() -> ("Value"=w1035:i32)  [unwired: 2 in, 2 out]
        n448 = property on="Y Velocity SP step/sec" class="DigNum (strict)"() -> ("Value"=w1047:i32)  [unwired: 2 in, 2 out]
        n449 = To Double Precision Float(number=w998) -> (double precision float=w999:dbl)
        n450 = To Double Precision Float(number=w996) -> (double precision float=w1002:dbl)
        n451 = To Double Precision Float(number=w1039) -> (double precision float=w1044:dbl)
        n452 = To Double Precision Float(number=w1014) -> (double precision float=w1015:dbl)
        n453 = To Double Precision Float(number=w1012) -> (double precision float=w1018:dbl)
        n454 = To Double Precision Float(number=w1033) -> (double precision float=w1038:dbl)
        n455 = To Double Precision Float(number=w1006) -> (double precision float=w1007:dbl)
        n456 = To Double Precision Float(number=w1004) -> (double precision float=w1010:dbl)
        n457 = To Double Precision Float(number=w1045) -> (double precision float=w1050:dbl)
        n458 = To Double Precision Float(number=w1022) -> (double precision float=w1023:dbl)
        n459 = To Double Precision Float(number=w1020) -> (double precision float=w1026:dbl)
        n460 = Divide(x=w999, y=w1002) -> (x/y=w1001:dbl)
        n461 = Divide(x=w1015, y=w1018) -> (x/y=w1017:dbl)
        n462 = Divide(x=w1007, y=w1010) -> (x/y=w1009:dbl)
        n463 = Divide(x=w1023, y=w1026) -> (x/y=w1025:dbl)
        n464 = To Double Precision Float(number=w1029) -> (double precision float=w1030:dbl)
        n465 = To Double Precision Float(number=w1027) -> (double precision float=w1032:dbl)
        n466 = To Double Precision Float(number=w1041) -> (double precision float=w1042:dbl)
        n467 = To Double Precision Float(number=w1035) -> (double precision float=w1036:dbl)
        n468 = To Double Precision Float(number=w1047) -> (double precision float=w1048:dbl)
        n469 = property on="R deg/rev" class="DigNum (strict)"() -> ("Value"=w994:dbl)  [unwired: 2 in, 2 out]
        n470 = property on="X mm/rev" class="DigNum (strict)"() -> ("Value"=w992:dbl)  [unwired: 2 in, 2 out]
        n471 = property on="Z mm/rev" class="DigNum (strict)"() -> ("Value"=w993:dbl)  [unwired: 2 in, 2 out]
        n472 = property on="Y mm/rev" class="DigNum (strict)"() -> ("Value"=w991:dbl)  [unwired: 2 in, 2 out]
        n473 = Divide(x=w1030, y=w1032) -> (x/y=w1031:dbl)
        n474 = Multiply(x=w1001, y=w994) -> (x*y=w1000:dbl)
        n475 = Divide(x=w1042, y=w1044) -> (x/y=w1043:dbl)
        n476 = Multiply(x=w1017, y=w992) -> (x*y=w1016:dbl)
        n477 = Divide(x=w1036, y=w1038) -> (x/y=w1037:dbl)
        n478 = Multiply(x=w1009, y=w993) -> (x*y=w1008:dbl)
        n479 = Divide(x=w1048, y=w1050) -> (x/y=w1049:dbl)
        n480 = Multiply(x=w1025, y=w991) -> (x*y=w1024:dbl)
        n481 = Multiply(x=w1031, y=w994) -> (x*y=w1028:dbl)
        n482 = Add(x=w1000, y=w995) -> (x+y=w997:dbl)
        n483 = Multiply(x=w1043, y=w992) -> (x*y=w1040:dbl)
        n484 = Add(x=w1016, y=w1011) -> (x+y=w1013:dbl)
        n485 = Multiply(x=w1037, y=w993) -> (x*y=w1034:dbl)
        n486 = Add(x=w1008, y=w1003) -> (x+y=w1005:dbl)
        n487 = Multiply(x=w1049, y=w991) -> (x*y=w1046:dbl)
        n488 = Add(x=w1024, y=w1019) -> (x+y=w1021:dbl)
        n489 = Absolute Value(x=w1028) -> (abs(x)=w990:dbl)
        n490 = property on="R Velocity MVdeg/sec" class="DigNum (strict)"("Val(Sgnl)"=w990) -> ()  [unwired: 2 in, 2 out]
        n491 = property on="R Position MV deg" class="DigNum (strict)"("Val(Sgnl)"=w997) -> ()  [unwired: 2 in, 2 out]
        n492 = property on="X Velocity MV mm/sec" class="DigNum (strict)"("Val(Sgnl)"=w1040) -> ()  [unwired: 2 in, 2 out]
        n493 = property on="X Position MV mm" class="DigNum (strict)"("Val(Sgnl)"=w1013) -> ()  [unwired: 2 in, 2 out]
        n494 = property on="Z Velocity MV mm/sec" class="DigNum (strict)"("Val(Sgnl)"=w1034) -> ()  [unwired: 2 in, 2 out]
        n495 = property on="Z Position MV mm" class="DigNum (strict)"("Val(Sgnl)"=w1005) -> ()  [unwired: 2 in, 2 out]
        n496 = property on="Y Velocity MV mm/sec" class="DigNum (strict)"("Val(Sgnl)"=w1046) -> ()  [unwired: 2 in, 2 out]
        n497 = property on="Y Position MV mm" class="DigNum (strict)"("Val(Sgnl)"=w1021) -> ()  [unwired: 2 in, 2 out]
      }
      event #3 {
        n498 = event-data() -> ()  [unwired: 1 in, 5 out]
        n499 = property on="X Step PV" class="DigNum (strict)"() -> ("Value"=w1115:i32)  [unwired: 2 in, 2 out]
        n500 = property on="Y Step PV" class="DigNum (strict)"() -> ("Value"=w1101:i32)  [unwired: 2 in, 2 out]
        n501 = property on="Z Step PV" class="DigNum (strict)"() -> ("Value"=w1088:i32)  [unwired: 2 in, 2 out]
        n502 = property on="R Step PV" class="DigNum (strict)"() -> ("Value"=w1074:i32)  [unwired: 2 in, 2 out]
        n503 = property on="X Step SP" class="DigNum (strict)"() -> ("Minimum"=w1122:dbl)  [unwired: 2 in, 2 out]
        n504 = property on="X Step SP" class="DigNum (strict)"() -> ("Maximum"=w1121:dbl)  [unwired: 2 in, 2 out]
        n505 = property on="Y Step SP" class="DigNum (strict)"() -> ("Minimum"=w1108:dbl)  [unwired: 2 in, 2 out]
        n506 = property on="Y Step SP" class="DigNum (strict)"() -> ("Maximum"=w1107:dbl)  [unwired: 2 in, 2 out]
        n507 = property on="Z Step SP" class="DigNum (strict)"() -> ("Minimum"=w1095:dbl)  [unwired: 2 in, 2 out]
        n508 = property on="Z Step SP" class="DigNum (strict)"() -> ("Maximum"=w1094:dbl)  [unwired: 2 in, 2 out]
        n509 = property on="R Step SP" class="DigNum (strict)"() -> ("Minimum"=w1079:dbl)  [unwired: 2 in, 2 out]
        n510 = property on="R Step SP" class="DigNum (strict)"() -> ("Maximum"=w1082:dbl)  [unwired: 2 in, 2 out]
        n511 = property on="X steps/rev" class="DigNum (strict)"() -> ("Value"=w1117:u32)  [unwired: 2 in, 2 out]
        n512 = property on="Y steps/rev" class="DigNum (strict)"() -> ("Value"=w1103:u32)  [unwired: 2 in, 2 out]
        n513 = property on="Z steps/rev" class="DigNum (strict)"() -> ("Value"=w1090:u32)  [unwired: 2 in, 2 out]
        n514 = property on="R steps/rev" class="DigNum (strict)"() -> ("Value"=w1076:u32)  [unwired: 2 in, 2 out]
        n515 = To Double Precision Float(number=w1115) -> (double precision float=w1068:dbl)
        n516 = To Double Precision Float(number=w1101) -> (double precision float=w1067:dbl)
        n517 = To Double Precision Float(number=w1088) -> (double precision float=w1066:dbl)
        n518 = To Double Precision Float(number=w1074) -> (double precision float=w1065:dbl)
        n519 = Subtract(x=w1122, y=w1068) -> (x-y=w1123:dbl)
        n520 = Subtract(x=w1121, y=w1068) -> (x-y=w1120:dbl)
        n521 = Subtract(x=w1108, y=w1067) -> (x-y=w1109:dbl)
        n522 = Subtract(x=w1107, y=w1067) -> (x-y=w1106:dbl)
        n523 = Subtract(x=w1095, y=w1066) -> (x-y=w1096:dbl)
        n524 = Subtract(x=w1094, y=w1066) -> (x-y=w1093:dbl)
        n525 = Subtract(x=w1079, y=w1065) -> (x-y=w1080:dbl)
        n526 = Subtract(x=w1082, y=w1065) -> (x-y=w1081:dbl)
        n527 = property on="X Scan Length SP steps" class="DigNum (strict)"() -> ("Value"=w1113:i32)  [unwired: 2 in, 2 out]
        n528 = To Double Precision Float(number=w1117) -> (double precision float=w1114:dbl)
        n529 = property on="Y Scan Length SP steps" class="DigNum (strict)"() -> ("Value"=w1104:i32)  [unwired: 2 in, 2 out]
        n530 = To Double Precision Float(number=w1103) -> (double precision float=w1058:dbl)
        n531 = property on="Z Scan Length SP steps" class="DigNum (strict)"() -> ("Value"=w1091:i32)  [unwired: 2 in, 2 out]
        n532 = To Double Precision Float(number=w1090) -> (double precision float=w1087:dbl)
        n533 = property on="R Scan Length SP steps" class="DigNum (strict)"() -> ("Value"=w1077:i32)  [unwired: 2 in, 2 out]
        n534 = To Double Precision Float(number=w1076) -> (double precision float=w1073:dbl)
        n535 = property on="Z Scan Velocity SP steps/sec" class="DigNum (strict)"() -> ("Value"=w1086:i32)  [unwired: 2 in, 2 out]
        n536 = property on="R Scan Velocity SP steps/sec" class="DigNum (strict)"() -> ("Value"=w1072:i32)  [unwired: 2 in, 2 out]
        n537 = property on="X Scan Velocity SP steps/sec" class="DigNum (strict)"() -> ("Value"=w1118:i32)  [unwired: 2 in, 2 out]
        n538 = property on="Y Scan Velocity SP steps/sec" class="DigNum (strict)"() -> ("Value"=w1100:i32)  [unwired: 2 in, 2 out]
        n539 = To Double Precision Float(number=w1091) -> (double precision float=w1064:dbl)
        n540 = To Double Precision Float(number=w1077) -> (double precision float=w1062:dbl)
        n541 = property on="X Scan Length SP steps" class="DigNum (strict)"("Minimum"=w1123) -> ()  [unwired: 2 in, 2 out]
        n542 = property on="X Scan Length SP steps" class="DigNum (strict)"("Maximum"=w1120) -> ()  [unwired: 2 in, 2 out]
        n543 = property on="Y Scan Length SP steps" class="DigNum (strict)"("Minimum"=w1109) -> ()  [unwired: 2 in, 2 out]
        n544 = property on="Y Scan Length SP steps" class="DigNum (strict)"("Maximum"=w1106) -> ()  [unwired: 2 in, 2 out]
        n545 = property on="Z Scan Length SP steps" class="DigNum (strict)"("Minimum"=w1096) -> ()  [unwired: 2 in, 2 out]
        n546 = property on="Z Scan Length SP steps" class="DigNum (strict)"("Maximum"=w1093) -> ()  [unwired: 2 in, 2 out]
        n547 = property on="R Scan Length SP steps" class="DigNum (strict)"("Minimum"=w1080) -> ()  [unwired: 2 in, 2 out]
        n548 = property on="R Scan Length SP steps" class="DigNum (strict)"("Maximum"=w1081) -> ()  [unwired: 2 in, 2 out]
        n549 = To Double Precision Float(number=w1113) -> (double precision float=w1053:dbl)
        n550 = To Double Precision Float(number=w1104) -> (double precision float=w1057:dbl)
        n551 = Divide(x=w1062, y=w1073) -> (x/y=w1078:dbl)
        n552 = Divide(x=w1053, y=w1114) -> (x/y=w1112:dbl)
        n553 = Divide(x=w1057, y=w1058) -> (x/y=w1105:dbl)
        n554 = Divide(x=w1064, y=w1087) -> (x/y=w1092:dbl)
        n555 = To Double Precision Float(number=w1072) -> (double precision float=w1061:dbl)
        n556 = property on="R deg/rev" class="DigNum (strict)"() -> ("Value"=w1075:dbl)  [unwired: 2 in, 2 out]
        n557 = To Double Precision Float(number=w1118) -> (double precision float=w1052:dbl)
        n558 = To Double Precision Float(number=w1100) -> (double precision float=w1056:dbl)
        n559 = To Double Precision Float(number=w1086) -> (double precision float=w1063:dbl)
        n560 = property on="X mm/rev" class="DigNum (strict)"() -> ("Value"=w1116:dbl)  [unwired: 2 in, 2 out]
        n561 = property on="Y mm/rev" class="DigNum (strict)"() -> ("Value"=w1102:dbl)  [unwired: 2 in, 2 out]
        n562 = property on="Z mm/rev" class="DigNum (strict)"() -> ("Value"=w1089:dbl)  [unwired: 2 in, 2 out]
        n563 = Divide(x=w1053, y=w1052) -> (x/y=→"X Scan Duration":dbl)
        n564 = Multiply(x=w1116, y=w1112) -> (x*y=w1110:dbl)
        n565 = Divide(x=w1052, y=w1114) -> (x/y=w1119:dbl)
        n566 = Divide(x=w1057, y=w1056) -> (x/y=→"Y Scan Duration":dbl)
        n567 = Multiply(x=w1105, y=w1102) -> (x*y=w1098:dbl)
        n568 = Divide(x=w1056, y=w1058) -> (x/y=w1099:dbl)
        n569 = Divide(x=w1064, y=w1063) -> (x/y=→"Z Scan Duration":dbl)
        n570 = Multiply(x=w1092, y=w1089) -> (x*y=w1084:dbl)
        n571 = Divide(x=w1063, y=w1087) -> (x/y=w1085:dbl)
        n572 = Divide(x=w1062, y=w1061) -> (x/y=→"R Scan Duration":dbl)
        n573 = Multiply(x=w1078, y=w1075) -> (x*y=w1070:dbl)
        n574 = Divide(x=w1061, y=w1073) -> (x/y=w1071:dbl)
        n575 = Multiply(x=w1119, y=w1116) -> (x*y=w1111:dbl)
        n576 = Multiply(x=w1102, y=w1099) -> (x*y=w1097:dbl)
        n577 = Multiply(x=w1089, y=w1085) -> (x*y=w1083:dbl)
        n578 = Multiply(x=w1075, y=w1071) -> (x*y=w1069:dbl)
        n579 = property on="X Scan length MV mm" class="DigNum (strict)"("Val(Sgnl)"=w1110) -> ()  [unwired: 2 in, 2 out]
        n580 = property on="Y Scan length MV mm" class="DigNum (strict)"("Value"=w1098) -> ()  [unwired: 2 in, 2 out]
        n581 = property on="Z Scan length MV mm" class="DigNum (strict)"("Value"=w1084) -> ()  [unwired: 2 in, 2 out]
        n582 = property on="R Scan length MV deg" class="DigNum (strict)"("Value"=w1070) -> ()  [unwired: 2 in, 2 out]
        n583 = Absolute Value(x=w1069) -> (abs(x)=w1051:dbl)
        n584 = property on="X Scan velocity MV mm/sec" class="DigNum (strict)"("Value"=w1111) -> ()  [unwired: 2 in, 2 out]
        n585 = property on="Y Scan velocity MV mm/sec" class="DigNum (strict)"("Val(Sgnl)"=w1097) -> ()  [unwired: 2 in, 2 out]
        n586 = property on="Z Scan velocity MV mm/sec" class="DigNum (strict)"("Val(Sgnl)"=w1083) -> ()  [unwired: 2 in, 2 out]
        n587 = property on="R Scan Velocity SP deg/sec" class="DigNum (strict)"("Val(Sgnl)"=w1051) -> ()  [unwired: 2 in, 2 out]
      }
      event #4 {
        n588 = event-data() -> ()  [unwired: 1 in, 7 out]
        n589 = property on="Y Step SP" class="DigNum (strict)"() -> ("Maximum"=w1134:dbl)  [unwired: 2 in, 2 out]
        n590 = property on="Y Step SP" class="DigNum (strict)"() -> ("Minimum"=w1133:dbl)  [unwired: 2 in, 2 out]
        n591 = property on="Y steps/rev" class="DigNum (strict)"() -> ("Value"=w1140:u32)  [unwired: 2 in, 2 out]
        n592 = property on="Y offset mm" class="DigNum (strict)"() -> ("Value"=w1138:dbl)  [unwired: 2 in, 2 out]
        n593 = property on="Y Velocity SP step/sec" class="DigNum (strict)"() -> ("Maximum"=w1127:dbl)  [unwired: 2 in, 2 out]
        n594 = property on="Y Velocity SP step/sec" class="DigNum (strict)"() -> ("Minimum"=w1126:dbl)  [unwired: 2 in, 2 out]
        n595 = property on="Y Position SP mm" class="DigNum (strict)"() -> ("Value"=w1137:dbl)  [unwired: 2 in, 2 out]
        n596 = property on="Y mm/rev" class="DigNum (strict)"() -> ("Value"=w1124:dbl)  [unwired: 2 in, 2 out]
        n597 = property on="Y Velocity SP mm/sec" class="DigNum (strict)"() -> ("Value"=w1131:dbl)  [unwired: 2 in, 2 out]
        n598 = Subtract(x=w1137, y=w1138) -> (x-y=w1141:dbl)
        n599 = Divide(x=w1131, y=w1124) -> (x/y=w1132:dbl)
        n600 = To Double Precision Float(number=w1140) -> (double precision float=w1125:dbl)
        n601 = Divide(x=w1141, y=w1124) -> (x/y=w1142:dbl)
        n602 = Multiply(x=w1132, y=w1125) -> (x*y=w1129:dbl)
        n603 = Multiply(x=w1142, y=w1125) -> (x*y=w1136:dbl)
        n604 = In Range and Coerce(upper limit=w1127, x=w1129, lower limit=w1126) -> (coerced(x)=w1128:dbl)  [unwired: 1 out]
        n605 = To Long Integer(number=w1128) -> (32bit integer=w1130:i32)
        n606 = In Range and Coerce(upper limit=w1134, x=w1136, lower limit=w1133) -> (coerced(x)=w1135:dbl)  [unwired: 1 out]
        n607 = To Long Integer(number=w1135) -> (32bit integer=w1139:i32)
        n608 = property on="Y Velocity SP step/sec" class="DigNum (strict)"("Val(Sgnl)"=w1130) -> ()  [unwired: 2 in, 2 out]
        n609 = property on="Y Step SP" class="DigNum (strict)"("Val(Sgnl)"=w1139) -> ()  [unwired: 2 in, 2 out]
      }
      event #5 {
        n610 = event-data() -> ()  [unwired: 1 in, 7 out]
        n611 = property on="X Step SP" class="DigNum (strict)"() -> ("Maximum"=w1153:dbl)  [unwired: 2 in, 2 out]
        n612 = property on="X Step SP" class="DigNum (strict)"() -> ("Minimum"=w1152:dbl)  [unwired: 2 in, 2 out]
        n613 = property on="X steps/rev" class="DigNum (strict)"() -> ("Value"=w1159:u32)  [unwired: 2 in, 2 out]
        n614 = property on="X offset mm" class="DigNum (strict)"() -> ("Value"=w1157:dbl)  [unwired: 2 in, 2 out]
        n615 = property on="X Velocity SP step/sec" class="DigNum (strict)"() -> ("Maximum"=w1146:dbl)  [unwired: 2 in, 2 out]
        n616 = property on="X Velocity SP step/sec" class="DigNum (strict)"() -> ("Minimum"=w1145:dbl)  [unwired: 2 in, 2 out]
        n617 = property on="X Position SP mm" class="DigNum (strict)"() -> ("Value"=w1156:dbl)  [unwired: 2 in, 2 out]
        n618 = property on="X mm/rev" class="DigNum (strict)"() -> ("Value"=w1143:dbl)  [unwired: 2 in, 2 out]
        n619 = property on="X Velocity SP mm/sec" class="DigNum (strict)"() -> ("Value"=w1150:dbl)  [unwired: 2 in, 2 out]
        n620 = Subtract(x=w1156, y=w1157) -> (x-y=w1160:dbl)
        n621 = Divide(x=w1150, y=w1143) -> (x/y=w1151:dbl)
        n622 = To Double Precision Float(number=w1159) -> (double precision float=w1144:dbl)
        n623 = Divide(x=w1160, y=w1143) -> (x/y=w1161:dbl)
        n624 = Multiply(x=w1151, y=w1144) -> (x*y=w1148:dbl)
        n625 = Multiply(x=w1161, y=w1144) -> (x*y=w1155:dbl)
        n626 = In Range and Coerce(upper limit=w1146, x=w1148, lower limit=w1145) -> (coerced(x)=w1147:dbl)  [unwired: 1 out]
        n627 = To Long Integer(number=w1147) -> (32bit integer=w1149:i32)
        n628 = In Range and Coerce(upper limit=w1153, x=w1155, lower limit=w1152) -> (coerced(x)=w1154:dbl)  [unwired: 1 out]
        n629 = To Long Integer(number=w1154) -> (32bit integer=w1158:i32)
        n630 = property on="X Velocity SP step/sec" class="DigNum (strict)"("Val(Sgnl)"=w1149) -> ()  [unwired: 2 in, 2 out]
        n631 = property on="X Step SP" class="DigNum (strict)"("Val(Sgnl)"=w1158) -> ()  [unwired: 2 in, 2 out]
      }
      event #6 {
        n632 = event-data() -> ()  [unwired: 1 in, 7 out]
        n633 = property on="Z Step SP" class="DigNum (strict)"() -> ("Maximum"=w1170:dbl)  [unwired: 2 in, 2 out]
        n634 = property on="Z Step SP" class="DigNum (strict)"() -> ("Minimum"=w1169:dbl)  [unwired: 2 in, 2 out]
        n635 = property on="Z steps/rev" class="DigNum (strict)"() -> ("Value"=w1176:u32)  [unwired: 2 in, 2 out]
        n636 = property on="Z offset mm" class="DigNum (strict)"() -> ("Value"=w1174:dbl)  [unwired: 2 in, 2 out]
        n637 = property on="Z Velocity SP step/sec" class="DigNum (strict)"() -> ("Maximum"=w1163:dbl)  [unwired: 2 in, 2 out]
        n638 = property on="Z Velocity SP step/sec" class="DigNum (strict)"() -> ("Minimum"=w1162:dbl)  [unwired: 2 in, 2 out]
        n639 = property on="Z Position SP mm" class="DigNum (strict)"() -> ("Value"=w1173:dbl)  [unwired: 2 in, 2 out]
        n640 = property on="Z mm/rev" class="DigNum (strict)"() -> ("Value"=w1179:dbl)  [unwired: 2 in, 2 out]
        n641 = property on="Z Velocity SP mm/sec" class="DigNum (strict)"() -> ("Value"=w1167:dbl)  [unwired: 2 in, 2 out]
        n642 = Subtract(x=w1173, y=w1174) -> (x-y=w1177:dbl)
        n643 = Divide(x=w1167, y=w1179) -> (x/y=w1168:dbl)
        n644 = To Double Precision Float(number=w1176) -> (double precision float=w1180:dbl)
        n645 = Divide(x=w1177, y=w1179) -> (x/y=w1178:dbl)
        n646 = Multiply(x=w1168, y=w1180) -> (x*y=w1165:dbl)
        n647 = Multiply(x=w1178, y=w1180) -> (x*y=w1172:dbl)
        n648 = In Range and Coerce(upper limit=w1163, x=w1165, lower limit=w1162) -> (coerced(x)=w1164:dbl)  [unwired: 1 out]
        n649 = To Long Integer(number=w1164) -> (32bit integer=w1166:i32)
        n650 = In Range and Coerce(upper limit=w1170, x=w1172, lower limit=w1169) -> (coerced(x)=w1171:dbl)  [unwired: 1 out]
        n651 = To Long Integer(number=w1171) -> (32bit integer=w1175:i32)
        n652 = property on="Z Velocity SP step/sec" class="DigNum (strict)"("Val(Sgnl)"=w1166) -> ()  [unwired: 2 in, 2 out]
        n653 = property on="Z Step SP" class="DigNum (strict)"("Val(Sgnl)"=w1175) -> ()  [unwired: 2 in, 2 out]
      }
      event #7 {
        n654 = event-data() -> ()  [unwired: 1 in, 7 out]
        n655 = property on="R Step SP" class="DigNum (strict)"() -> ("Maximum"=w1192:dbl)  [unwired: 2 in, 2 out]
        n656 = property on="R Step SP" class="DigNum (strict)"() -> ("Minimum"=w1191:dbl)  [unwired: 2 in, 2 out]
        n657 = property on="R steps/rev" class="DigNum (strict)"() -> ("Value"=w1198:u32)  [unwired: 2 in, 2 out]
        n658 = property on="R offset deg" class="DigNum (strict)"() -> ("Value"=w1196:dbl)  [unwired: 2 in, 2 out]
        n659 = property on="R Velocity SP step/sec" class="DigNum (strict)"() -> ("Maximum"=w1185:dbl)  [unwired: 2 in, 2 out]
        n660 = property on="R Velocity SP step/sec" class="DigNum (strict)"() -> ("Minimum"=w1184:dbl)  [unwired: 2 in, 2 out]
        n661 = property on="R Position SP deg" class="DigNum (strict)"() -> ("Value"=w1195:dbl)  [unwired: 2 in, 2 out]
        n662 = property on="R deg/rev" class="DigNum (strict)"() -> ("Value"=w1182:dbl)  [unwired: 2 in, 2 out]
        n663 = property on="R Velocity SP deg/sec" class="DigNum (strict)"() -> ("Value"=w1189:dbl)  [unwired: 2 in, 2 out]
        n664 = Subtract(x=w1195, y=w1196) -> (x-y=w1199:dbl)
        n665 = Divide(x=w1189, y=w1182) -> (x/y=w1190:dbl)
        n666 = To Double Precision Float(number=w1198) -> (double precision float=w1183:dbl)
        n667 = Divide(x=w1199, y=w1182) -> (x/y=w1200:dbl)
        n668 = Multiply(x=w1190, y=w1183) -> (x*y=w1187:dbl)
        n669 = Absolute Value(x=w1187) -> (abs(x)=w1181:dbl)
        n670 = Multiply(x=w1200, y=w1183) -> (x*y=w1194:dbl)
        n671 = In Range and Coerce(upper limit=w1185, x=w1181, lower limit=w1184) -> (coerced(x)=w1186:dbl)  [unwired: 1 out]
        n672 = To Long Integer(number=w1186) -> (32bit integer=w1188:i32)
        n673 = In Range and Coerce(upper limit=w1192, x=w1194, lower limit=w1191) -> (coerced(x)=w1193:dbl)  [unwired: 1 out]
        n674 = To Long Integer(number=w1193) -> (32bit integer=w1197:i32)
        n675 = property on="R Velocity SP step/sec" class="DigNum (strict)"("Val(Sgnl)"=w1188) -> ()  [unwired: 2 in, 2 out]
        n676 = property on="R Step SP" class="DigNum (strict)"("Val(Sgnl)"=w1197) -> ()  [unwired: 2 in, 2 out]
      }
      event #8 {
        n677 = event-data() -> ()  [unwired: 1 in, 7 out]
        n678 = property on="Y Step SP" class="DigNum (strict)"() -> ("Maximum"=w1210:dbl)  [unwired: 2 in, 2 out]
        n679 = property on="Y Step SP" class="DigNum (strict)"() -> ("Minimum"=w1211:dbl)  [unwired: 2 in, 2 out]
        n680 = property on="Y steps/rev" class="DigNum (strict)"() -> ("Value"=w1216:u32)  [unwired: 2 in, 2 out]
        n681 = property on="Y Scan Length SP mm" class="DigNum (strict)"() -> ("Value"=w1214:dbl)  [unwired: 2 in, 2 out]
        n682 = property on="Y mm/rev" class="DigNum (strict)"() -> ("Value"=w1201:dbl)  [unwired: 2 in, 2 out]
        n683 = property on="Y Scan Velocity SP steps/sec" class="DigNum (strict)"() -> ("Maximum"=w1204:dbl)  [unwired: 2 in, 2 out]
        n684 = property on="Y Scan Velocity SP steps/sec" class="DigNum (strict)"() -> ("Minimum"=w1203:dbl)  [unwired: 2 in, 2 out]
        n685 = property on="Y Scan Velocity SP mm/sec" class="DigNum (strict)"() -> ("Value"=w1208:dbl)  [unwired: 2 in, 2 out]
        n686 = Divide(x=w1214, y=w1201) -> (x/y=w1217:dbl)
        n687 = To Double Precision Float(number=w1216) -> (double precision float=w1202:dbl)
        n688 = Multiply(x=w1217, y=w1202) -> (x*y=w1213:dbl)
        n689 = Divide(x=w1208, y=w1201) -> (x/y=w1209:dbl)
        n690 = Multiply(x=w1209, y=w1202) -> (x*y=w1206:dbl)
        n691 = In Range and Coerce(upper limit=w1210, x=w1213, lower limit=w1211) -> (coerced(x)=w1212:dbl)  [unwired: 1 out]
        n692 = To Long Integer(number=w1212) -> (32bit integer=w1215:i32)
        n693 = In Range and Coerce(upper limit=w1204, x=w1206, lower limit=w1203) -> (coerced(x)=w1205:dbl)  [unwired: 1 out]
        n694 = To Long Integer(number=w1205) -> (32bit integer=w1207:i32)
        n695 = property on="Y Scan Length SP steps" class="DigNum (strict)"("Val(Sgnl)"=w1215) -> ()  [unwired: 2 in, 2 out]
        n696 = property on="Y Scan Velocity SP steps/sec" class="DigNum (strict)"("Val(Sgnl)"=w1207) -> ()  [unwired: 2 in, 2 out]
      }
      event #9 {
        n697 = event-data() -> ()  [unwired: 1 in, 7 out]
        n698 = property on="X Step SP" class="DigNum (strict)"() -> ("Maximum"=w1227:dbl)  [unwired: 2 in, 2 out]
        n699 = property on="X Step SP" class="DigNum (strict)"() -> ("Minimum"=w1228:dbl)  [unwired: 2 in, 2 out]
        n700 = property on="X steps/rev" class="DigNum (strict)"() -> ("Value"=w1233:u32)  [unwired: 2 in, 2 out]
        n701 = property on="X Scan Length SP mm" class="DigNum (strict)"() -> ("Value"=w1231:dbl)  [unwired: 2 in, 2 out]
        n702 = property on="X mm/rev" class="DigNum (strict)"() -> ("Value"=w1218:dbl)  [unwired: 2 in, 2 out]
        n703 = property on="X Scan Velocity SP steps/sec" class="DigNum (strict)"() -> ("Maximum"=w1221:dbl)  [unwired: 2 in, 2 out]
        n704 = property on="X Scan Velocity SP steps/sec" class="DigNum (strict)"() -> ("Minimum"=w1220:dbl)  [unwired: 2 in, 2 out]
        n705 = property on="X Scan Velocity SP mm/sec" class="DigNum (strict)"() -> ("Value"=w1225:dbl)  [unwired: 2 in, 2 out]
        n706 = Divide(x=w1231, y=w1218) -> (x/y=w1234:dbl)
        n707 = To Double Precision Float(number=w1233) -> (double precision float=w1219:dbl)
        n708 = Multiply(x=w1234, y=w1219) -> (x*y=w1230:dbl)
        n709 = Divide(x=w1225, y=w1218) -> (x/y=w1226:dbl)
        n710 = Multiply(x=w1226, y=w1219) -> (x*y=w1223:dbl)
        n711 = In Range and Coerce(upper limit=w1227, x=w1230, lower limit=w1228) -> (coerced(x)=w1229:dbl)  [unwired: 1 out]
        n712 = To Long Integer(number=w1229) -> (32bit integer=w1232:i32)
        n713 = In Range and Coerce(upper limit=w1221, x=w1223, lower limit=w1220) -> (coerced(x)=w1222:dbl)  [unwired: 1 out]
        n714 = To Long Integer(number=w1222) -> (32bit integer=w1224:i32)
        n715 = property on="X Scan Length SP steps" class="DigNum (strict)"("Val(Sgnl)"=w1232) -> ()  [unwired: 2 in, 2 out]
        n716 = property on="X Scan Velocity SP steps/sec" class="DigNum (strict)"("Val(Sgnl)"=w1224) -> ()  [unwired: 2 in, 2 out]
      }
      event #10 {
        n717 = event-data() -> ()  [unwired: 1 in, 7 out]
        n718 = property on="Z Step SP" class="DigNum (strict)"() -> ("Maximum"=w1244:dbl)  [unwired: 2 in, 2 out]
        n719 = property on="Z Step SP" class="DigNum (strict)"() -> ("Minimum"=w1245:dbl)  [unwired: 2 in, 2 out]
        n720 = property on="Z steps/rev" class="DigNum (strict)"() -> ("Value"=w1250:u32)  [unwired: 2 in, 2 out]
        n721 = property on="Z Scan Length SP mm" class="DigNum (strict)"() -> ("Value"=w1248:dbl)  [unwired: 2 in, 2 out]
        n722 = property on="Z mm/rev" class="DigNum (strict)"() -> ("Value"=w1235:dbl)  [unwired: 2 in, 2 out]
        n723 = property on="Z Scan Velocity SP steps/sec" class="DigNum (strict)"() -> ("Maximum"=w1238:dbl)  [unwired: 2 in, 2 out]
        n724 = property on="Z Scan Velocity SP steps/sec" class="DigNum (strict)"() -> ("Minimum"=w1237:dbl)  [unwired: 2 in, 2 out]
        n725 = property on="Z Scan Velocity SP mm/sec" class="DigNum (strict)"() -> ("Value"=w1242:dbl)  [unwired: 2 in, 2 out]
        n726 = Divide(x=w1248, y=w1235) -> (x/y=w1251:dbl)
        n727 = To Double Precision Float(number=w1250) -> (double precision float=w1236:dbl)
        n728 = Multiply(x=w1251, y=w1236) -> (x*y=w1247:dbl)
        n729 = Divide(x=w1242, y=w1235) -> (x/y=w1243:dbl)
        n730 = Multiply(x=w1243, y=w1236) -> (x*y=w1240:dbl)
        n731 = In Range and Coerce(upper limit=w1244, x=w1247, lower limit=w1245) -> (coerced(x)=w1246:dbl)  [unwired: 1 out]
        n732 = To Long Integer(number=w1246) -> (32bit integer=w1249:i32)
        n733 = In Range and Coerce(upper limit=w1238, x=w1240, lower limit=w1237) -> (coerced(x)=w1239:dbl)  [unwired: 1 out]
        n734 = To Long Integer(number=w1239) -> (32bit integer=w1241:i32)
        n735 = property on="Z Scan Length SP steps" class="DigNum (strict)"("Val(Sgnl)"=w1249) -> ()  [unwired: 2 in, 2 out]
        n736 = property on="Z Scan Velocity SP steps/sec" class="DigNum (strict)"("Val(Sgnl)"=w1241) -> ()  [unwired: 2 in, 2 out]
      }
      event #11 {
        n737 = event-data() -> ()  [unwired: 1 in, 7 out]
        n738 = property on="R Step SP" class="DigNum (strict)"() -> ("Maximum"=w1262:dbl)  [unwired: 2 in, 2 out]
        n739 = property on="R Step SP" class="DigNum (strict)"() -> ("Minimum"=w1263:dbl)  [unwired: 2 in, 2 out]
        n740 = property on="R steps/rev" class="DigNum (strict)"() -> ("Value"=w1268:u32)  [unwired: 2 in, 2 out]
        n741 = property on="R Velocity SP step/sec" class="DigNum (strict)"() -> ("Maximum"=w1256:dbl)  [unwired: 2 in, 2 out]
        n742 = property on="R Scan Length SP deg" class="DigNum (strict)"() -> ("Value"=w1266:dbl)  [unwired: 2 in, 2 out]
        n743 = property on="R deg/rev" class="DigNum (strict)"() -> ("Value"=w1253:dbl)  [unwired: 2 in, 2 out]
        n744 = property on="R Scan Velocity SP steps/sec" class="DigNum (strict)"() -> ("Minimum"=w1255:dbl)  [unwired: 2 in, 2 out]
        n745 = property on="R Scan Velocity SP deg/sec" class="DigNum (strict)"() -> ("Value"=w1260:dbl)  [unwired: 2 in, 2 out]
        n746 = Divide(x=w1266, y=w1253) -> (x/y=w1269:dbl)
        n747 = To Double Precision Float(number=w1268) -> (double precision float=w1254:dbl)
        n748 = Multiply(x=w1269, y=w1254) -> (x*y=w1265:dbl)
        n749 = Divide(x=w1260, y=w1253) -> (x/y=w1261:dbl)
        n750 = Multiply(x=w1261, y=w1254) -> (x*y=w1258:dbl)
        n751 = In Range and Coerce(upper limit=w1262, x=w1265, lower limit=w1263) -> (coerced(x)=w1264:dbl)  [unwired: 1 out]
        n752 = Absolute Value(x=w1258) -> (abs(x)=w1252:dbl)
        n753 = To Long Integer(number=w1264) -> (32bit integer=w1267:i32)
        n754 = In Range and Coerce(upper limit=w1256, x=w1252, lower limit=w1255) -> (coerced(x)=w1257:dbl)  [unwired: 1 out]
        n755 = To Long Integer(number=w1257) -> (32bit integer=w1259:i32)
        n756 = property on="R Scan Length SP steps" class="DigNum (strict)"("Val(Sgnl)"=w1267) -> ()  [unwired: 2 in, 2 out]
        n757 = property on="R Scan Velocity SP steps/sec" class="DigNum (strict)"("Val(Sgnl)"=w1259) -> ()  [unwired: 2 in, 2 out]
      }
      event #12 {
        n758 = event-data() -> ()  [unwired: 1 in, 7 out]
        n759 = flat-sequence {
          tunnel: w1274 -> [w1284]
          tunnel: w1275 -> [w1285]
          tunnel: [w1285] -> w1271
          tunnel: [w1284] -> w1270
          tunnel: [w1288] -> w1273
          tunnel: [w1287] -> w1272
          tunnel: w1271 -> [w1290]
          tunnel: w1270 -> [w1289]
          tunnel: [w1308] -> w1277
          tunnel: [w1307] -> w1276
          tunnel: w1273 -> [w1306]
          tunnel: w1272 -> [w1305]
          tunnel: [w1315] -> w1279
          tunnel: [w1314] -> w1278
          tunnel: w1277 -> [w1313]
          tunnel: w1276 -> [w1312]
          tunnel: [w1321] -> w1280
          tunnel: [w1322] -> w1281
          tunnel: w1279 -> [w1322]
          tunnel: w1278 -> [w1320]
          frame #0 {
            n760 = property on="Y Go" class="Bool"("DisabledEnum"=T1."Disabled and Grayed Out" ("Disabled")) -> ()  [unwired: 2 in, 2 out]
            n761 = property on="Scan Go" class="Bool"("DisabledEnum"=T1."Disabled and Grayed Out" ("Disabled")) -> ()  [unwired: 2 in, 2 out]
          }
          frame #1 {
            n762 = property on="Y Step SP" class="DigNum (strict)"() -> ("Value"=w1298:i32)  [unwired: 2 in, 2 out]
            n763 = property on="Y Step PV" class="DigNum (strict)"() -> ("Value"=w1297:i32)  [unwired: 2 in, 2 out]
            n764 = property on="Y Backlash" class="DigNum (strict)"() -> ("Value"=w1286:i32)  [unwired: 2 in, 2 out]
            n765 = Subtract(x=w1298, y=w1297) -> (x-y=w1296:i32)
            n766 = Sign(1:w1286) -> (0:w1294:i32)
            n767 = Sign(1:w1296) -> (0:w1295:i32)
            n768 = Multiply(x=w1295, y=w1294) -> (x*y=w1293:i32)
            n769 = Equal?(x=w1293, y=1) -> (x = y?=w1291:bool)
            n770 = case shown="False" w1291 {
              tunnel: w1290 -> [w1301 w1303]
              tunnel: w1289 -> [w1300 w1302]
              tunnel: [w1300 w1302] -> w1288
              tunnel: [w1301 w1303] -> w1287
              frame #0 {
                n771 = property on="Y Backlash corr" class="Bool (strict)"("Val(Sgnl)"=FALSE ("Value (Signaling)")) -> ()  [unwired: 2 in, 2 out]
              }
              frame #1 {
                n772 = property on="Y Backlash corr" class="Bool (strict)"("Val(Sgnl)"=TRUE ("Value (Signaling)")) -> ()  [unwired: 2 in, 2 out]
              }
            }
          }
          frame #2 {
            # "Velocity Setting"
            n773 = property on="Y Velocity SP step/sec" class="DigNum (strict)"() -> ("Value"=w1309:i32)  [unwired: 2 in, 2 out]
            n774 = Number To Decimal String(number=w1309) -> (decimal integer string=w1310:string)  [unwired: 1 in]
            n775 = call "mDrive Send Command.vi"("error in (no error)"=w1306, "Extra"=w1310, "Command"=T2."Max Velocity", "VISA resource name"=w1305) -> ("error out"=w1307:errorcluster, "VISA resource name out"=w1308:refnum<visa-resource-name>)  [unwired: 3 in, 1 out]
          }
          frame #3 {
            # "Move to Abs Position"
            n776 = property on="Y Step SP" class="DigNum (strict)"() -> ("Value"=w1318:i32)  [unwired: 2 in, 2 out]
            n777 = Number To Decimal String(number=w1318) -> (decimal integer string=w1317:string)  [unwired: 1 in]
            n778 = call "mDrive Send Command.vi"("error in (no error)"=w1312, "Extra"=w1317, "Command"=T2."Move to Absolute Position", "VISA resource name"=w1313) -> ("error out"=w1314:errorcluster, "VISA resource name out"=w1315:refnum<visa-resource-name>)  [unwired: 3 in, 1 out]
          }
          frame #4 {
            n779 = call "Time Delay"("error in (no error)"=w1320, "Delay Time (s)"=0.1) -> ("error out"=w1321:errorcluster)  [unwired: 9 in]
          }
        }
      }
      event #13 {
        n780 = event-data() -> ()  [unwired: 1 in, 7 out]
        n781 = flat-sequence {
          tunnel: w1325 -> [w1337]
          tunnel: w1326 -> [w1338]
          tunnel: [w1338] -> w1328
          tunnel: [w1337] -> w1327
          tunnel: [w1341] -> w1330
          tunnel: [w1340] -> w1329
          tunnel: w1328 -> [w1343]
          tunnel: w1327 -> [w1342]
          tunnel: [w1361] -> w1332
          tunnel: [w1360] -> w1331
          tunnel: w1330 -> [w1359]
          tunnel: w1329 -> [w1358]
          tunnel: [w1368] -> w1334
          tunnel: [w1367] -> w1333
          tunnel: w1332 -> [w1366]
          tunnel: w1331 -> [w1365]
          tunnel: [w1374] -> w1324
          tunnel: [w1375] -> w1323
          tunnel: w1334 -> [w1375]
          tunnel: w1333 -> [w1373]
          frame #0 {
            n782 = property on="Z Go" class="Bool"("DisabledEnum"=T1."Disabled and Grayed Out" ("Disabled")) -> ()  [unwired: 2 in, 2 out]
            n783 = property on="Scan Go" class="Bool"("DisabledEnum"=T1."Disabled and Grayed Out" ("Disabled")) -> ()  [unwired: 2 in, 2 out]
          }
          frame #1 {
            n784 = property on="Z Step SP" class="DigNum (strict)"() -> ("Value"=w1351:i32)  [unwired: 2 in, 2 out]
            n785 = property on="Z Step PV" class="DigNum (strict)"() -> ("Value"=w1350:i32)  [unwired: 2 in, 2 out]
            n786 = property on="Z Backlash" class="DigNum (strict)"() -> ("Value"=w1339:i32)  [unwired: 2 in, 2 out]
            n787 = Subtract(x=w1351, y=w1350) -> (x-y=w1349:i32)
            n788 = Sign(1:w1339) -> (0:w1347:i32)
            n789 = Sign(1:w1349) -> (0:w1348:i32)
            n790 = Multiply(x=w1348, y=w1347) -> (x*y=w1346:i32)
            n791 = Equal?(x=w1346, y=1) -> (x = y?=w1344:bool)
            n792 = case shown="True" w1344 {
              tunnel: w1343 -> [w1354 w1356]
              tunnel: w1342 -> [w1353 w1355]
              tunnel: [w1353 w1355] -> w1341
              tunnel: [w1354 w1356] -> w1340
              frame #0 {
                n793 = property on="Z Backlash corr" class="Bool (strict)"("Val(Sgnl)"=FALSE ("Value (Signaling)")) -> ()  [unwired: 2 in, 2 out]
              }
              frame #1 {
                n794 = property on="Z Backlash corr" class="Bool (strict)"("Val(Sgnl)"=TRUE ("Value (Signaling)")) -> ()  [unwired: 2 in, 2 out]
              }
            }
          }
          frame #2 {
            # "Velocity Setting"
            n795 = property on="Z Velocity SP step/sec" class="DigNum (strict)"() -> ("Value"=w1362:i32)  [unwired: 2 in, 2 out]
            n796 = Number To Decimal String(number=w1362) -> (decimal integer string=w1363:string)  [unwired: 1 in]
            n797 = call "mDrive Send Command.vi"("error in (no error)"=w1359, "Extra"=w1363, "Command"=T2."Max Velocity", "VISA resource name"=w1358) -> ("error out"=w1360:errorcluster, "VISA resource name out"=w1361:refnum<visa-resource-name>)  [unwired: 3 in, 1 out]
          }
          frame #3 {
            # "Move to Abs Position"
            n798 = property on="Z Step SP" class="DigNum (strict)"() -> ("Value"=w1371:i32)  [unwired: 2 in, 2 out]
            n799 = Number To Decimal String(number=w1371) -> (decimal integer string=w1370:string)  [unwired: 1 in]
            n800 = call "mDrive Send Command.vi"("error in (no error)"=w1365, "Extra"=w1370, "Command"=T2."Move to Absolute Position", "VISA resource name"=w1366) -> ("error out"=w1367:errorcluster, "VISA resource name out"=w1368:refnum<visa-resource-name>)  [unwired: 3 in, 1 out]
          }
          frame #4 {
            n801 = call "Time Delay28"("error in (no error)"=w1373, "Delay Time (s)"=0.1) -> ("error out"=w1374:errorcluster)  [unwired: 9 in]
          }
        }
      }
      event #14 {
        n802 = event-data() -> ()  [unwired: 1 in, 7 out]
        n803 = flat-sequence {
          tunnel: w1378 -> [w1390]
          tunnel: w1379 -> [w1391]
          tunnel: [w1391] -> w1381
          tunnel: [w1390] -> w1380
          tunnel: [w1394] -> w1383
          tunnel: [w1393] -> w1382
          tunnel: w1381 -> [w1396]
          tunnel: w1380 -> [w1395]
          tunnel: [w1414] -> w1385
          tunnel: [w1413] -> w1384
          tunnel: w1383 -> [w1412]
          tunnel: w1382 -> [w1411]
          tunnel: [w1421] -> w1387
          tunnel: [w1420] -> w1386
          tunnel: w1385 -> [w1419]
          tunnel: w1384 -> [w1418]
          tunnel: [w1427] -> w1377
          tunnel: [w1428] -> w1376
          tunnel: w1387 -> [w1428]
          tunnel: w1386 -> [w1426]
          frame #0 {
            n804 = property on="R Go" class="Bool"("DisabledEnum"=T1."Disabled and Grayed Out" ("Disabled")) -> ()  [unwired: 2 in, 2 out]
            n805 = property on="Scan Go" class="Bool"("DisabledEnum"=T1."Disabled and Grayed Out" ("Disabled")) -> ()  [unwired: 2 in, 2 out]
          }
          frame #1 {
            n806 = property on="R Step SP" class="DigNum (strict)"() -> ("Value"=w1404:i32)  [unwired: 2 in, 2 out]
            n807 = property on="R Step PV" class="DigNum (strict)"() -> ("Value"=w1403:i32)  [unwired: 2 in, 2 out]
            n808 = property on="R Backlash" class="DigNum (strict)"() -> ("Value"=w1392:i32)  [unwired: 2 in, 2 out]
            n809 = Subtract(x=w1404, y=w1403) -> (x-y=w1402:i32)
            n810 = Sign(1:w1392) -> (0:w1400:i32)
            n811 = Sign(1:w1402) -> (0:w1401:i32)
            n812 = Multiply(x=w1401, y=w1400) -> (x*y=w1399:i32)
            n813 = Equal?(x=w1399, y=1) -> (x = y?=w1397:bool)
            n814 = case shown="True" w1397 {
              tunnel: w1396 -> [w1407 w1409]
              tunnel: w1395 -> [w1406 w1408]
              tunnel: [w1406 w1408] -> w1394
              tunnel: [w1407 w1409] -> w1393
              frame #0 {
                n815 = property on="R Backlash corr" class="Bool (strict)"("Val(Sgnl)"=FALSE ("Value (Signaling)")) -> ()  [unwired: 2 in, 2 out]
              }
              frame #1 {
                n816 = property on="R Backlash corr" class="Bool (strict)"("Val(Sgnl)"=TRUE ("Value (Signaling)")) -> ()  [unwired: 2 in, 2 out]
              }
            }
          }
          frame #2 {
            # "Velocity Setting"
            n817 = property on="R Velocity SP step/sec" class="DigNum (strict)"() -> ("Value"=w1415:i32)  [unwired: 2 in, 2 out]
            n818 = Number To Decimal String(number=w1415) -> (decimal integer string=w1416:string)  [unwired: 1 in]
            n819 = call "mDrive Send Command.vi"("error in (no error)"=w1412, "Extra"=w1416, "Command"=T2."Max Velocity", "VISA resource name"=w1411) -> ("error out"=w1413:errorcluster, "VISA resource name out"=w1414:refnum<visa-resource-name>)  [unwired: 3 in, 1 out]
          }
          frame #3 {
            # "Move to Abs Position"
            n820 = property on="R Step SP" class="DigNum (strict)"() -> ("Value"=w1424:i32)  [unwired: 2 in, 2 out]
            n821 = Number To Decimal String(number=w1424) -> (decimal integer string=w1423:string)  [unwired: 1 in]
            n822 = call "mDrive Send Command.vi"("error in (no error)"=w1418, "Extra"=w1423, "Command"=T2."Move to Absolute Position", "VISA resource name"=w1419) -> ("error out"=w1420:errorcluster, "VISA resource name out"=w1421:refnum<visa-resource-name>)  [unwired: 3 in, 1 out]
          }
          frame #4 {
            n823 = call "Time Delay29"("error in (no error)"=w1426, "Delay Time (s)"=0.1) -> ("error out"=w1427:errorcluster)  [unwired: 9 in]
          }
        }
      }
      event #15 {
        n824 = event-data() -> ()  [unwired: 1 in, 7 out]
        n825 = flat-sequence {
          tunnel: [w1442] -> w1434
          tunnel: [w1441] -> w1433
          tunnel: w1432 -> [w1442]
          tunnel: w1431 -> [w1441]
          tunnel: [w1447] -> w1436
          tunnel: [w1446] -> w1435
          tunnel: w1434 -> [w1449]
          tunnel: w1433 -> [w1448]
          tunnel: [w1467] -> w1438
          tunnel: [w1466] -> w1437
          tunnel: w1436 -> [w1465]
          tunnel: w1435 -> [w1464]
          tunnel: [w1474] -> w1440
          tunnel: [w1473] -> w1439
          tunnel: w1438 -> [w1472]
          tunnel: w1437 -> [w1471]
          tunnel: [w1480] -> w1429
          tunnel: [w1481] -> w1430
          tunnel: w1440 -> [w1481]
          tunnel: w1439 -> [w1479]
          frame #0 {
            n826 = property on="X Go" class="Bool"("DisabledEnum"=T1."Disabled and Grayed Out" ("Disabled")) -> ()  [unwired: 2 in, 2 out]
            n827 = property on="Scan Go" class="Bool"("DisabledEnum"=T1."Disabled and Grayed Out" ("Disabled")) -> ()  [unwired: 2 in, 2 out]
          }
          frame #1 {
            n828 = property on="X Step SP" class="DigNum (strict)"() -> ("Value"=w1457:i32)  [unwired: 2 in, 2 out]
            n829 = property on="X Step PV" class="DigNum (strict)"() -> ("Value"=w1456:i32)  [unwired: 2 in, 2 out]
            n830 = property on="X Backlash" class="DigNum (strict)"() -> ("Value"=w1445:i32)  [unwired: 2 in, 2 out]
            n831 = Subtract(x=w1457, y=w1456) -> (x-y=w1455:i32)
            n832 = Sign(1:w1445) -> (0:w1453:i32)
            n833 = Sign(1:w1455) -> (0:w1454:i32)
            n834 = Multiply(x=w1454, y=w1453) -> (x*y=w1452:i32)
            n835 = Equal?(x=w1452, y=1) -> (x = y?=w1450:bool)
            n836 = case shown="True" w1450 {
              tunnel: w1449 -> [w1460 w1462]
              tunnel: w1448 -> [w1459 w1461]
              tunnel: [w1459 w1461] -> w1447
              tunnel: [w1460 w1462] -> w1446
              frame #0 {
                n837 = property on="X Backlash corr" class="Bool (strict)"("Val(Sgnl)"=FALSE ("Value (Signaling)")) -> ()  [unwired: 2 in, 2 out]
              }
              frame #1 {
                n838 = property on="X Backlash corr" class="Bool (strict)"("Val(Sgnl)"=TRUE ("Value (Signaling)")) -> ()  [unwired: 2 in, 2 out]
              }
            }
          }
          frame #2 {
            # "Velocity Setting"
            n839 = property on="X Velocity SP step/sec" class="DigNum (strict)"() -> ("Value"=w1468:i32)  [unwired: 2 in, 2 out]
            n840 = Number To Decimal String(number=w1468) -> (decimal integer string=w1469:string)  [unwired: 1 in]
            n841 = call "mDrive Send Command.vi"("error in (no error)"=w1465, "Extra"=w1469, "Command"=T2."Max Velocity", "VISA resource name"=w1464) -> ("error out"=w1466:errorcluster, "VISA resource name out"=w1467:refnum<visa-resource-name>)  [unwired: 3 in, 1 out]
          }
          frame #3 {
            # "Move to Abs Position"
            n842 = property on="X Step SP" class="DigNum (strict)"() -> ("Value"=w1477:i32)  [unwired: 2 in, 2 out]
            n843 = Number To Decimal String(number=w1477) -> (decimal integer string=w1476:string)  [unwired: 1 in]
            n844 = call "mDrive Send Command.vi"("error in (no error)"=w1471, "Extra"=w1476, "Command"=T2."Move to Absolute Position", "VISA resource name"=w1472) -> ("error out"=w1473:errorcluster, "VISA resource name out"=w1474:refnum<visa-resource-name>)  [unwired: 3 in, 1 out]
          }
          frame #4 {
            n845 = call "Time Delay15"("error in (no error)"=w1479, "Delay Time (s)"=0.1) -> ("error out"=w1480:errorcluster)  [unwired: 9 in]
          }
        }
      }
      event #16 {
        n846 = event-data() -> ()  [unwired: 1 in, 7 out]
        n847 = flat-sequence {
          tunnel: [w1497] -> w1489
          tunnel: [w1495] -> w1488
          tunnel: w1487 -> [w1491]
          tunnel: w1486 -> [w1490]
          tunnel: w1489 -> [w1512]
          tunnel: w1488 -> [w1511]
          tunnel: [w1512] -> w1483
          tunnel: [w1511] -> w1482
          tunnel: [w1514] -> w1484
          tunnel: [w1515] -> w1485
          tunnel: w1483 -> [w1515]
          tunnel: w1482 -> [w1514]
          frame #0 {
            # "VELOCITY"
            n848 = property on="X Scan Velocity SP steps/sec" class="DigNum (strict)"() -> ("Value"=w1498:i32)  [unwired: 2 in, 2 out]
            n849 = Number To Decimal String(number=w1498) -> (decimal integer string=w1499:string)  [unwired: 1 in]
            n850 = call "mDrive Send Command.vi"("error in (no error)"=w1490, "Extra"=w1499, "Command"=T2."Max Velocity", "VISA resource name"=w1491) -> ("error out"=w1500:errorcluster, "VISA resource name out"=w1505:refnum<visa-resource-name>)  [unwired: 3 in, 1 out]
            n851 = call "Time Delay9"("error in (no error)"=w1500) -> ("error out"=w1503:errorcluster)  [unwired: 10 in]
            n852 = call "mDrive Send Command.vi"("error in (no error)"=w1503, "Extra"="VM", "Command"=T2."Print Parameter", "VISA resource name"=w1505) -> ("error out"=w1496:errorcluster, "read buffer"=w1501:string, "VISA resource name out"=w1497:refnum<visa-resource-name>)  [unwired: 3 in]
            n853 = call "Time Delay10"("error in (no error)"=w1496) -> ("error out"=w1495:errorcluster)  [unwired: 10 in]
            n854 = Decimal String To Number(string=w1501, offset=0) -> (number=w1504:i32)  [unwired: 1 in, 1 out]
            n855 = property on="X velocity PV step/sec" class="DigNum (strict)"("Val(Sgnl)"=w1504) -> ()  [unwired: 2 in, 2 out]
          }
          frame #1 {
            n856 = property on="X Scan" class="Bool (strict)"("Val(Sgnl)"=TRUE ("Slew Ready 2")) -> ()  [unwired: 2 in, 2 out]
            n857 = property on="Scan Go" class="Bool"("DisabledEnum"=T1."Enabled" ("Disabled")) -> ()  [unwired: 2 in, 2 out]
            n858 = property on="Scan Cancel" class="Bool"("DisabledEnum"=T1."Enabled" ("Disabled")) -> ()  [unwired: 2 in, 2 out]
            n859 = property on="X Scan Length SP steps" class="DigNum (strict)"("DisabledEnum"=T1."Disabled and Grayed Out" ("Disabled")) -> ()  [unwired: 2 in, 2 out]
            n860 = property on="X Scan Velocity SP steps/sec" class="DigNum (strict)"("DisabledEnum"=T1."Disabled and Grayed Out" ("Disabled")) -> ()  [unwired: 2 in, 2 out]
          }
          frame #2 {
            n861 = property on="X Go" class="Bool"("DisabledEnum"=T1."Disabled and Grayed Out" ("Disabled")) -> ()  [unwired: 2 in, 2 out]
          }
        }
      }
      event #17 {
        n862 = event-data() -> ()  [unwired: 1 in, 7 out]
        n863 = flat-sequence {
          tunnel: w1523 -> [w1533]
          tunnel: w1522 -> [w1532]
          tunnel: [w1529] -> w1520
          tunnel: [w1527] -> w1519
          tunnel: w1520 -> [w1546]
          tunnel: w1519 -> [w1545]
          tunnel: [w1546] -> w1517
          tunnel: [w1545] -> w1516
          tunnel: [w1548] -> w1521
          tunnel: [w1549] -> w1518
          tunnel: w1517 -> [w1549]
          tunnel: w1516 -> [w1548]
          frame #0 {
            # "VELOCITY"
            n864 = property on="Y Scan Velocity SP steps/sec" class="DigNum (strict)"() -> ("Value"=w1530:i32)  [unwired: 2 in, 2 out]
            n865 = Number To Decimal String(number=w1530) -> (decimal integer string=w1531:string)  [unwired: 1 in]
            n866 = call "mDrive Send Command.vi"("error in (no error)"=w1533, "Extra"=w1531, "Command"=T2."Max Velocity", "VISA resource name"=w1532) -> ("error out"=w1534:errorcluster, "VISA resource name out"=w1539:refnum<visa-resource-name>)  [unwired: 3 in, 1 out]
            n867 = call "Time Delay5"("error in (no error)"=w1534) -> ("error out"=w1537:errorcluster)  [unwired: 10 in]
            n868 = call "mDrive Send Command.vi"("error in (no error)"=w1537, "Extra"="VM", "Command"=T2."Print Parameter", "VISA resource name"=w1539) -> ("error out"=w1528:errorcluster, "read buffer"=w1535:string, "VISA resource name out"=w1529:refnum<visa-resource-name>)  [unwired: 3 in]
            n869 = Decimal String To Number(string=w1535, offset=0) -> (number=w1538:i32)  [unwired: 1 in, 1 out]
            n870 = property on="Y velocity PV step/sec" class="DigNum (strict)"("Val(Sgnl)"=w1538) -> ()  [unwired: 2 in, 2 out]
            n871 = call "Time Delay6"("error in (no error)"=w1528) -> ("error out"=w1527:errorcluster)  [unwired: 10 in]
          }
          frame #1 {
            n872 = property on="Y Scan" class="Bool (strict)"("Val(Sgnl)"=TRUE ("Slew Ready 2")) -> ()  [unwired: 2 in, 2 out]
            n873 = property on="Scan Go" class="Bool"("DisabledEnum"=T1."Enabled" ("Disabled")) -> ()  [unwired: 2 in, 2 out]
            n874 = property on="Scan Cancel" class="Bool"("DisabledEnum"=T1."Enabled" ("Disabled")) -> ()  [unwired: 2 in, 2 out]
            n875 = property on="Y Scan Length SP steps" class="DigNum (strict)"("DisabledEnum"=T1."Disabled and Grayed Out" ("Disabled")) -> ()  [unwired: 2 in, 2 out]
            n876 = property on="Y Scan Velocity SP steps/sec" class="DigNum (strict)"("DisabledEnum"=T1."Disabled and Grayed Out" ("Disabled")) -> ()  [unwired: 2 in, 2 out]
          }
          frame #2 {
            n877 = property on="Y Go" class="Bool"("DisabledEnum"=T1."Disabled and Grayed Out" ("Disabled")) -> ()  [unwired: 2 in, 2 out]
          }
        }
      }
      event #18 {
        n878 = event-data() -> ()  [unwired: 1 in, 7 out]
        n879 = flat-sequence {
          tunnel: [w1565] -> w1557
          tunnel: [w1563] -> w1556
          tunnel: w1553 -> [w1559]
          tunnel: w1552 -> [w1558]
          tunnel: w1557 -> [w1580]
          tunnel: w1556 -> [w1579]
          tunnel: [w1580] -> w1555
          tunnel: [w1579] -> w1554
          tunnel: [w1582] -> w1551
          tunnel: [w1583] -> w1550
          tunnel: w1555 -> [w1583]
          tunnel: w1554 -> [w1582]
          frame #0 {
            # "VELOCITY"
            n880 = property on="Z Scan Velocity SP steps/sec" class="DigNum (strict)"() -> ("Value"=w1566:i32)  [unwired: 2 in, 2 out]
            n881 = Number To Decimal String(number=w1566) -> (decimal integer string=w1567:string)  [unwired: 1 in]
            n882 = call "mDrive Send Command.vi"("error in (no error)"=w1558, "Extra"=w1567, "Command"=T2."Max Velocity", "VISA resource name"=w1559) -> ("error out"=w1568:errorcluster, "VISA resource name out"=w1573:refnum<visa-resource-name>)  [unwired: 3 in, 1 out]
            n883 = call "Time Delay24"("error in (no error)"=w1568) -> ("error out"=w1571:errorcluster)  [unwired: 10 in]
            n884 = call "mDrive Send Command.vi"("error in (no error)"=w1571, "Extra"="VM", "Command"=T2."Print Parameter", "VISA resource name"=w1573) -> ("error out"=w1564:errorcluster, "read buffer"=w1569:string, "VISA resource name out"=w1565:refnum<visa-resource-name>)  [unwired: 3 in]
            n885 = Decimal String To Number(string=w1569, offset=0) -> (number=w1572:i32)  [unwired: 1 in, 1 out]
            n886 = property on="Z  velocity PV step/sec" class="DigNum (strict)"("Val(Sgnl)"=w1572) -> ()  [unwired: 2 in, 2 out]
            n887 = call "Time Delay25"("error in (no error)"=w1564) -> ("error out"=w1563:errorcluster)  [unwired: 10 in]
          }
          frame #1 {
            n888 = property on="Z Scan" class="Bool (strict)"("Val(Sgnl)"=TRUE ("Slew Ready 2")) -> ()  [unwired: 2 in, 2 out]
            n889 = property on="Scan Go" class="Bool"("DisabledEnum"=T1."Enabled" ("Disabled")) -> ()  [unwired: 2 in, 2 out]
            n890 = property on="Scan Cancel" class="Bool"("DisabledEnum"=T1."Enabled" ("Disabled")) -> ()  [unwired: 2 in, 2 out]
            n891 = property on="Z Scan Length SP steps" class="DigNum (strict)"("DisabledEnum"=T1."Disabled and Grayed Out" ("Disabled")) -> ()  [unwired: 2 in, 2 out]
            n892 = property on="Z Scan Velocity SP steps/sec" class="DigNum (strict)"("DisabledEnum"=T1."Disabled and Grayed Out" ("Disabled")) -> ()  [unwired: 2 in, 2 out]
          }
          frame #2 {
            n893 = property on="Z Go" class="Bool"("DisabledEnum"=T1."Disabled and Grayed Out" ("Disabled")) -> ()  [unwired: 2 in, 2 out]
          }
        }
      }
      event #19 {
        n894 = event-data() -> ()  [unwired: 1 in, 7 out]
        n895 = flat-sequence {
          tunnel: [w1599] -> w1591
          tunnel: [w1597] -> w1590
          tunnel: w1587 -> [w1593]
          tunnel: w1586 -> [w1592]
          tunnel: w1591 -> [w1614]
          tunnel: w1590 -> [w1613]
          tunnel: [w1614] -> w1589
          tunnel: [w1613] -> w1588
          tunnel: [w1616] -> w1584
          tunnel: [w1617] -> w1585
          tunnel: w1589 -> [w1617]
          tunnel: w1588 -> [w1616]
          frame #0 {
            # "VELOCITY"
            n896 = property on="R Scan Velocity SP steps/sec" class="DigNum (strict)"() -> ("Value"=w1600:i32)  [unwired: 2 in, 2 out]
            n897 = Number To Decimal String(number=w1600) -> (decimal integer string=w1601:string)  [unwired: 1 in]
            n898 = call "mDrive Send Command.vi"("error in (no error)"=w1592, "Extra"=w1601, "Command"=T2."Max Velocity", "VISA resource name"=w1593) -> ("error out"=w1602:errorcluster, "VISA resource name out"=w1607:refnum<visa-resource-name>)  [unwired: 3 in, 1 out]
            n899 = call "Time Delay26"("error in (no error)"=w1602) -> ("error out"=w1605:errorcluster)  [unwired: 10 in]
            n900 = call "mDrive Send Command.vi"("error in (no error)"=w1605, "Extra"="VM", "Command"=T2."Print Parameter", "VISA resource name"=w1607) -> ("error out"=w1598:errorcluster, "read buffer"=w1603:string, "VISA resource name out"=w1599:refnum<visa-resource-name>)  [unwired: 3 in]
            n901 = Decimal String To Number(string=w1603, offset=0) -> (number=w1606:i32)  [unwired: 1 in, 1 out]
            n902 = property on="R velocity PV step/sec" class="DigNum (strict)"("Val(Sgnl)"=w1606) -> ()  [unwired: 2 in, 2 out]
            n903 = call "Time Delay27"("error in (no error)"=w1598) -> ("error out"=w1597:errorcluster)  [unwired: 10 in]
          }
          frame #1 {
            n904 = property on="R Scan" class="Bool (strict)"("Val(Sgnl)"=TRUE ("Slew Ready 2")) -> ()  [unwired: 2 in, 2 out]
            n905 = property on="Scan Go" class="Bool"("DisabledEnum"=T1."Enabled" ("Disabled")) -> ()  [unwired: 2 in, 2 out]
            n906 = property on="Scan Cancel" class="Bool"("DisabledEnum"=T1."Enabled" ("Disabled")) -> ()  [unwired: 2 in, 2 out]
            n907 = property on="R Scan Length SP steps" class="DigNum (strict)"("DisabledEnum"=T1."Disabled and Grayed Out" ("Disabled")) -> ()  [unwired: 2 in, 2 out]
            n908 = property on="R Scan Velocity SP steps/sec" class="DigNum (strict)"("DisabledEnum"=T1."Disabled and Grayed Out" ("Disabled")) -> ()  [unwired: 2 in, 2 out]
          }
          frame #2 {
            n909 = property on="R Go" class="Bool"("DisabledEnum"=T1."Disabled and Grayed Out" ("Disabled")) -> ()  [unwired: 2 in, 2 out]
          }
        }
      }
      event #20 {
        n910 = event-data() -> ()  [unwired: 1 in, 4 out]
        n911 = event-data() -> ()  [unwired: 3 in, 1 out]
      }
      event #21 {
        n912 = event-data() -> ()  [unwired: 1 in, 7 out]
        n913 = flat-sequence {
          tunnel: w1624 -> [w1641]
          tunnel: w1623 -> [w1640]
          tunnel: [w1639] -> w1622
          tunnel: [w1637] -> _
          tunnel: [w1637] -> w1621
          frame #0 {
            n914 = call "mDrive Send Command.vi"("error in (no error)"=w1640, "Command"=T2."Stop", "VISA resource name"=w1641) -> ("error out"=w1637:errorcluster, "VISA resource name out"=w1639:refnum<visa-resource-name>)  [unwired: 4 in, 1 out]
          }
        }
        n915 = flat-sequence {
          tunnel: w1636 -> [w1656]
          tunnel: w1635 -> [w1655]
          tunnel: [w1654] -> w1634
          tunnel: [w1653] -> w1633
          frame #0 {
            n916 = call "mDrive Send Command.vi"("error in (no error)"=w1655, "Command"=T2."Stop", "VISA resource name"=w1656) -> ("error out"=w1653:errorcluster, "VISA resource name out"=w1654:refnum<visa-resource-name>)  [unwired: 4 in, 1 out]
          }
        }
        n917 = flat-sequence {
          tunnel: [w1645] -> w1626
          tunnel: [w1644] -> w1625
          tunnel: w1628 -> [w1643]
          tunnel: w1627 -> [w1642]
          frame #0 {
            n918 = call "mDrive Send Command.vi"("error in (no error)"=w1642, "Command"=T2."Stop", "VISA resource name"=w1643) -> ("error out"=w1644:errorcluster, "VISA resource name out"=w1645:refnum<visa-resource-name>)  [unwired: 4 in, 1 out]
          }
        }
        n919 = flat-sequence {
          tunnel: [w1650] -> w1632
          tunnel: [w1649] -> w1631
          tunnel: w1630 -> [w1648]
          tunnel: w1629 -> [w1647]
          frame #0 {
            n920 = call "mDrive Send Command.vi"("error in (no error)"=w1647, "Command"=T2."Stop", "VISA resource name"=w1648) -> ("error out"=w1649:errorcluster, "VISA resource name out"=w1650:refnum<visa-resource-name>)  [unwired: 4 in, 1 out]
          }
        }
      }
      event #22 {
        n921 = event-data() -> ()  [unwired: 1 in, 7 out]
        n922 = flat-sequence {
          tunnel: [w1687] -> w1662
          tunnel: [w1686] -> w1661
          tunnel: w1660 -> [w1684]
          tunnel: w1659 -> [w1683]
          tunnel: [w1694] -> w1657
          tunnel: [w1695] -> w1658
          tunnel: w1662 -> [w1695]
          tunnel: w1661 -> [w1694]
          frame #0 {
            n923 = call "mDrive Send Command.vi"("error in (no error)"=w1683, "Command"=T2."Stop", "VISA resource name"=w1684) -> ("error out"=w1686:errorcluster, "VISA resource name out"=w1687:refnum<visa-resource-name>)  [unwired: 4 in, 1 out]
          }
          frame #1 {
            n924 = property on="R Scan" class="Bool (strict)"("Value"=FALSE ("Slew Ready")) -> ()  [unwired: 2 in, 2 out]
            n925 = property on="R Scan OK" class="Bool"("DisabledEnum"=T1."Enabled" ("Disabled")) -> ()  [unwired: 2 in, 2 out]
            n926 = property on="R Scan Length SP steps" class="DigNum (strict)"("DisabledEnum"=T1."Enabled" ("Disabled")) -> ()  [unwired: 2 in, 2 out]
            n927 = property on="R Scan set" class="Bool"("DisabledEnum"=T1."Enabled" ("Disabled")) -> ()  [unwired: 2 in, 2 out]
            n928 = property on="R Scan Velocity SP steps/sec" class="DigNum (strict)"("DisabledEnum"=T1."Enabled" ("Disabled")) -> ()  [unwired: 2 in, 2 out]
            n929 = property on="R Go" class="Bool"("DisabledEnum"=T1."Enabled" ("Disabled")) -> ()  [unwired: 2 in, 2 out]
          }
        }
        n930 = flat-sequence {
          tunnel: w1680 -> [w1724]
          tunnel: w1679 -> [w1723]
          tunnel: [w1726] -> w1676
          tunnel: [w1725] -> w1675
          tunnel: [w1733] -> w1681
          tunnel: [w1734] -> w1682
          tunnel: w1676 -> [w1734]
          tunnel: w1675 -> [w1733]
          frame #0 {
            n931 = call "mDrive Send Command.vi"("error in (no error)"=w1723, "Command"=T2."Stop", "VISA resource name"=w1724) -> ("error out"=w1725:errorcluster, "VISA resource name out"=w1726:refnum<visa-resource-name>)  [unwired: 4 in, 1 out]
          }
          frame #1 {
            n932 = property on="Y Scan" class="Bool (strict)"("Value"=FALSE ("Slew Ready")) -> ()  [unwired: 2 in, 2 out]
            n933 = property on="Y Scan Velocity SP steps/sec" class="DigNum (strict)"("DisabledEnum"=T1."Enabled" ("Disabled")) -> ()  [unwired: 2 in, 2 out]
            n934 = property on="Y Go" class="Bool"("DisabledEnum"=T1."Enabled" ("Disabled")) -> ()  [unwired: 2 in, 2 out]
            n935 = property on="Y Scan OK" class="Bool"("DisabledEnum"=T1."Enabled" ("Disabled")) -> ()  [unwired: 2 in, 2 out]
            n936 = property on="Y Scan Length SP steps" class="DigNum (strict)"("DisabledEnum"=T1."Enabled" ("Disabled")) -> ()  [unwired: 2 in, 2 out]
            n937 = property on="Y Scan set" class="Bool"("DisabledEnum"=T1."Enabled" ("Disabled")) -> ()  [unwired: 2 in, 2 out]
          }
        }
        n938 = flat-sequence {
          tunnel: [w1700] -> w1668
          tunnel: [w1699] -> w1667
          tunnel: w1666 -> [w1697]
          tunnel: w1665 -> [w1696]
          tunnel: [w1707] -> w1663
          tunnel: [w1708] -> w1664
          tunnel: w1668 -> [w1708]
          tunnel: w1667 -> [w1707]
          frame #0 {
            n939 = call "mDrive Send Command.vi"("error in (no error)"=w1696, "Command"=T2."Stop", "VISA resource name"=w1697) -> ("error out"=w1699:errorcluster, "VISA resource name out"=w1700:refnum<visa-resource-name>)  [unwired: 4 in, 1 out]
          }
          frame #1 {
            n940 = property on="Z Scan" class="Bool (strict)"("Value"=FALSE ("Slew Ready")) -> ()  [unwired: 2 in, 2 out]
            n941 = property on="Z Scan set" class="Bool"("DisabledEnum"=T1."Enabled" ("Disabled")) -> ()  [unwired: 2 in, 2 out]
            n942 = property on="Z Scan Velocity SP steps/sec" class="DigNum (strict)"("DisabledEnum"=T1."Enabled" ("Disabled")) -> ()  [unwired: 2 in, 2 out]
            n943 = property on="Z Scan Length SP steps" class="DigNum (strict)"("DisabledEnum"=T1."Enabled" ("Disabled")) -> ()  [unwired: 2 in, 2 out]
            n944 = property on="Z Go" class="Bool"("DisabledEnum"=T1."Enabled" ("Disabled")) -> ()  [unwired: 2 in, 2 out]
            n945 = property on="Z Scan OK" class="Bool"("DisabledEnum"=T1."Enabled" ("Disabled")) -> ()  [unwired: 2 in, 2 out]
          }
        }
        n946 = flat-sequence {
          tunnel: w1672 -> [w1711]
          tunnel: w1671 -> [w1710]
          tunnel: [w1713] -> w1674
          tunnel: [w1712] -> w1673
          tunnel: [w1720] -> w1669
          tunnel: [w1721] -> w1670
          tunnel: w1674 -> [w1721]
          tunnel: w1673 -> [w1720]
          frame #0 {
            n947 = call "mDrive Send Command.vi"("error in (no error)"=w1710, "Command"=T2."Stop", "VISA resource name"=w1711) -> ("error out"=w1712:errorcluster, "VISA resource name out"=w1713:refnum<visa-resource-name>)  [unwired: 4 in, 1 out]
          }
          frame #1 {
            n948 = property on="X Scan" class="Bool (strict)"("Value"=FALSE ("Slew Ready")) -> ()  [unwired: 2 in, 2 out]
            n949 = property on="X Scan set" class="Bool"("DisabledEnum"=T1."Enabled" ("Disabled")) -> ()  [unwired: 2 in, 2 out]
            n950 = property on="X Scan Velocity SP steps/sec" class="DigNum (strict)"("DisabledEnum"=T1."Enabled" ("Disabled")) -> ()  [unwired: 2 in, 2 out]
            n951 = property on="X Scan Length SP steps" class="DigNum (strict)"("DisabledEnum"=T1."Enabled" ("Disabled")) -> ()  [unwired: 2 in, 2 out]
            n952 = property on="X Go" class="Bool"("DisabledEnum"=T1."Enabled" ("Disabled")) -> ()  [unwired: 2 in, 2 out]
            n953 = property on="X Scan OK" class="Bool"("DisabledEnum"=T1."Enabled" ("Disabled")) -> ()  [unwired: 2 in, 2 out]
          }
        }
        n954 = property on="Scan Go" class="Bool"("DisabledEnum"=T1."Disabled and Grayed Out" ("Disabled")) -> ()  [unwired: 2 in, 2 out]
        n955 = property on="Scan Cancel" class="Bool"("DisabledEnum"=T1."Disabled and Grayed Out" ("Disabled")) -> ()  [unwired: 2 in, 2 out]
      }
      event #23 {
        n956 = event-data() -> ()  [unwired: 1 in, 7 out]
        n957 = flat-sequence {
          tunnel: [w1814] -> w1798
          tunnel: [w1812] -> w1791
          tunnel: [w1813] -> w1788
          tunnel: [w1807] -> w1787
          tunnel: [w1811] -> w1786
          tunnel: [w1810] -> w1785
          tunnel: [w1809] -> w1784
          tunnel: [w1808] -> w1783
          tunnel: w1762 -> [w1806]
          tunnel: [w1806] -> w1761
          tunnel: w1760 -> [w1805]
          tunnel: [w1805] -> w1759
          tunnel: w1758 -> [w1804]
          tunnel: [w1804] -> w1757
          tunnel: w1756 -> [w1803]
          tunnel: [w1803] -> w1755
          tunnel: w1754 -> [w1802]
          tunnel: [w1802] -> w1753
          tunnel: w1752 -> [w1801]
          tunnel: [w1801] -> w1751
          tunnel: [w1800] -> w1750
          tunnel: w1749 -> [w1800]
          tunnel: [w1799] -> w1748
          tunnel: w1747 -> [w1799]
          tunnel: [w1866] -> w1795
          tunnel: [w1865] -> w1793
          tunnel: w1798 -> [w1864]
          tunnel: w1791 -> [w1863]
          tunnel: [w1863] -> w1789
          tunnel: w1788 -> [w1862]
          tunnel: w1787 -> [w1851]
          tunnel: w1786 -> [w1861]
          tunnel: w1785 -> [w1857]
          tunnel: w1784 -> [w1854]
          tunnel: w1783 -> [w1860]
          tunnel: [w1859] -> w1781
          tunnel: [w1858] -> w1779
          tunnel: [w1857] -> w1776
          tunnel: [w1856] -> w1774
          tunnel: [w1855] -> w1772
          tunnel: [w1854] -> w1770
          tunnel: [w1853] -> w1768
          tunnel: [w1852] -> w1766
          tunnel: [w1851] -> w1765
          tunnel: w1761 -> [w1850]
          tunnel: w1759 -> [w1849]
          tunnel: w1757 -> [w1848]
          tunnel: w1755 -> [w1847]
          tunnel: w1753 -> [w1846]
          tunnel: w1751 -> [w1845]
          tunnel: w1750 -> [w1844]
          tunnel: w1748 -> [w1843]
          tunnel: w1795 -> [w1907]
          tunnel: [w1907] -> w1794
          tunnel: w1793 -> [w1906]
          tunnel: [w1906] -> w1792
          tunnel: [w1904] -> w1790
          tunnel: w1789 -> [w1904]
          tunnel: [w1903] -> w1782
          tunnel: w1781 -> [w1903]
          tunnel: [w1902] -> w1780
          tunnel: w1779 -> [w1902]
          tunnel: [w1901] -> w1778
          tunnel: [w1900] -> w1777
          tunnel: w1776 -> [w1900]
          tunnel: [w1899] -> w1775
          tunnel: w1774 -> [w1899]
          tunnel: [w1898] -> w1773
          tunnel: w1772 -> [w1898]
          tunnel: [w1897] -> w1771
          tunnel: w1770 -> [w1897]
          tunnel: [w1896] -> w1769
          tunnel: w1768 -> [w1896]
          tunnel: [w1895] -> w1767
          tunnel: w1766 -> [w1895]
          tunnel: w1765 -> [w1901]
          tunnel: w1794 -> [w1927]
          tunnel: [w1925] -> w1797
          tunnel: w1792 -> [w1926]
          tunnel: [w1924] -> w1796
          tunnel: w1790 -> [w1923]
          tunnel: w1782 -> [w1922]
          tunnel: w1780 -> [w1921]
          tunnel: w1778 -> [w1920]
          tunnel: w1777 -> [w1919]
          tunnel: w1775 -> [w1918]
          tunnel: w1773 -> [w1917]
          tunnel: w1771 -> [w1916]
          tunnel: w1769 -> [w1915]
          tunnel: w1767 -> [w1914]
          tunnel: [w1913] -> w1764
          tunnel: [w1912] -> w1763
          tunnel: [w1911] -> w1742
          tunnel: [w1910] -> w1739
          tunnel: [w1909] -> w1737
          tunnel: [w1908] -> w1735
          tunnel: w1797 -> [w1985]
          tunnel: w1796 -> [w1984]
          tunnel: [w1985] -> w1746
          tunnel: [w1984] -> w1745
          tunnel: [w1978] -> w1744
          tunnel: w1764 -> [w1978]
          tunnel: [w1977] -> w1743
          tunnel: w1763 -> [w1977]
          tunnel: w1742 -> [w1967]
          tunnel: [w1967] -> w1741
          tunnel: [w1966] -> w1740
          tunnel: w1739 -> [w1966]
          tunnel: [w1965] -> w1738
          tunnel: w1737 -> [w1965]
          tunnel: [w1964] -> w1736
          tunnel: w1735 -> [w1964]
          frame #0 {
            n958 = property on="R Scan" class="Bool (strict)"() -> ("Value"=w1810:bool)  [unwired: 2 in, 2 out]
            n959 = property on="Y Scan" class="Bool (strict)"() -> ("Value"=w1812:bool)  [unwired: 2 in, 2 out]
            n960 = property on="Z Scan" class="Bool (strict)"() -> ("Value"=w1809:bool)  [unwired: 2 in, 2 out]
            n961 = property on="X Scan" class="Bool (strict)"() -> ("Value"=w1807:bool)  [unwired: 2 in, 2 out]
            n962 = case shown="True" w1810 {
              tunnel: ["" w1816] -> w1808
              frame #0 {
              }
              frame #1 {
                n963 = property on="R Scan Length SP steps" class="DigNum (strict)"() -> ("Value"=w1821:i32)  [unwired: 2 in, 2 out]
                n964 = Number To Decimal String(number=w1821) -> (decimal integer string=w1818:string)  [unwired: 1 in]
                n965 = call <vilib>:"Space Constant.vi"() -> ("String"=w1819:string)
                n966 = Concatenate Strings("MR", w1819, w1818, "\r") -> (w1816:string)
              }
            }
            n967 = case shown="True" w1812 {
              tunnel: ["" w1837] -> w1814
              frame #0 {
              }
              frame #1 {
                n968 = property on="Y Scan Length SP steps" class="DigNum (strict)"() -> ("Value"=w1842:i32)  [unwired: 2 in, 2 out]
                n969 = Number To Decimal String(number=w1842) -> (decimal integer string=w1839:string)  [unwired: 1 in]
                n970 = call <vilib>:"Space Constant.vi"() -> ("String"=w1840:string)
                n971 = Concatenate Strings("MR", w1840, w1839, "\r") -> (w1837:string)
              }
            }
            n972 = case shown="True" w1809 {
              tunnel: ["" w1823] -> w1811
              frame #0 {
              }
              frame #1 {
                n973 = property on="Z Scan Length SP steps" class="DigNum (strict)"() -> ("Value"=w1828:i32)  [unwired: 2 in, 2 out]
                n974 = Number To Decimal String(number=w1828) -> (decimal integer string=w1825:string)  [unwired: 1 in]
                n975 = call <vilib>:"Space Constant.vi"() -> ("String"=w1826:string)
                n976 = Concatenate Strings("MR", w1826, w1825, "\r") -> (w1823:string)
              }
            }
            n977 = case shown="True" w1807 {
              tunnel: ["" w1830] -> w1813
              frame #0 {
              }
              frame #1 {
                n978 = property on="X Scan Length SP steps" class="DigNum (strict)"() -> ("Value"=w1835:i32)  [unwired: 2 in, 2 out]
                n979 = Number To Decimal String(number=w1835) -> (decimal integer string=w1832:string)  [unwired: 1 in]
                n980 = call <vilib>:"Space Constant.vi"() -> ("String"=w1833:string)
                n981 = Concatenate Strings("MR", w1833, w1832, "\r") -> (w1830:string)
              }
            }
          }
          frame #1 {
            n982 = case shown="False" w1857 {
              tunnel: [w1868 w1873] -> w1856
              tunnel: [w1867 w1872] -> w1855
              tunnel: w1860 -> [_ w1871]
              tunnel: w1844 -> [w1868 w1870]
              tunnel: w1843 -> [w1867 w1869]
              frame #0 {
              }
              frame #1 {
                n983 = VISA Write(VISA resource name=w1870, write buffer=w1871, error in (no error)=w1869) -> (VISA resource name out=w1873:refnum<visa-resource-name>, error out=w1872:errorcluster)  [unwired: 1 out]
              }
            }
            n984 = case shown="False" w1863 {
              tunnel: [w1889 w1894] -> w1866
              tunnel: [w1888 w1893] -> w1865
              tunnel: w1864 -> [_ w1892]
              tunnel: w1848 -> [w1889 w1891]
              tunnel: w1847 -> [w1888 w1890]
              frame #0 {
              }
              frame #1 {
                n985 = VISA Write(VISA resource name=w1891, write buffer=w1892, error in (no error)=w1890) -> (VISA resource name out=w1894:refnum<visa-resource-name>, error out=w1893:errorcluster)  [unwired: 1 out]
              }
            }
            n986 = case shown="False" w1854 {
              tunnel: [w1875 w1880] -> w1853
              tunnel: [w1874 w1879] -> w1852
              tunnel: w1861 -> [_ w1878]
              tunnel: w1846 -> [w1875 w1877]
              tunnel: w1845 -> [w1874 w1876]
              frame #0 {
              }
              frame #1 {
                n987 = VISA Write(VISA resource name=w1877, write buffer=w1878, error in (no error)=w1876) -> (VISA resource name out=w1880:refnum<visa-resource-name>, error out=w1879:errorcluster)  [unwired: 1 out]
              }
            }
            n988 = case shown="False" w1851 {
              tunnel: [w1882 w1887] -> w1859
              tunnel: [w1881 w1886] -> w1858
              tunnel: w1862 -> [_ w1885]
              tunnel: w1850 -> [w1882 w1884]
              tunnel: w1849 -> [w1881 w1883]
              frame #0 {
              }
              frame #1 {
                n989 = VISA Write(VISA resource name=w1884, write buffer=w1885, error in (no error)=w1883) -> (VISA resource name out=w1887:refnum<visa-resource-name>, error out=w1886:errorcluster)  [unwired: 1 out]
              }
            }
          }
          frame #2 {
            n990 = call "Time Delay7"("Delay Time (s)"=0.1) -> ()  [unwired: 10 in, 1 out]
          }
          frame #3 {
            n991 = case shown="True" w1919 {
              tunnel: w1918 -> [w1938 w1942]
              tunnel: w1917 -> [w1937 w1941]
              tunnel: [w1938 w1940] -> w1911
              tunnel: [w1937 w1939] -> w1910
              frame #0 {
              }
              frame #1 {
                n992 = property class="Instr"(reference=w1942, error in=w1941) -> (reference out=w1944:refnum<visa-resource-name>, error out=w1943:errorcluster, "Serial Settings:Number of Bytes at Serial Port"=w1945:u32)
                n993 = VISA Read(VISA resource name=w1944, byte count=w1945, error in (no error)=w1943) -> (VISA resource name out=w1940:refnum<visa-resource-name>, error out=w1939:errorcluster)  [unwired: 2 out]
              }
            }
            n994 = case shown="True" w1923 {
              tunnel: w1927 -> [w1956 w1960]
              tunnel: w1926 -> [w1955 w1959]
              tunnel: [w1956 w1958] -> w1925
              tunnel: [w1955 w1957] -> w1924
              frame #0 {
              }
              frame #1 {
                n995 = property class="Instr"(reference=w1960, error in=w1959) -> (reference out=w1962:refnum<visa-resource-name>, error out=w1961:errorcluster, "Serial Settings:Number of Bytes at Serial Port"=w1963:u32)
                n996 = VISA Read(VISA resource name=w1962, byte count=w1963, error in (no error)=w1961) -> (VISA resource name out=w1958:refnum<visa-resource-name>, error out=w1957:errorcluster)  [unwired: 2 out]
              }
            }
            n997 = case shown="True" w1916 {
              tunnel: w1915 -> [w1929 w1933]
              tunnel: w1914 -> [w1928 w1932]
              tunnel: [w1929 w1931] -> w1913
              tunnel: [w1928 w1930] -> w1912
              frame #0 {
              }
              frame #1 {
                n998 = property class="Instr"(reference=w1933, error in=w1932) -> (reference out=w1935:refnum<visa-resource-name>, error out=w1934:errorcluster, "Serial Settings:Number of Bytes at Serial Port"=w1936:u32)
                n999 = VISA Read(VISA resource name=w1935, byte count=w1936, error in (no error)=w1934) -> (VISA resource name out=w1931:refnum<visa-resource-name>, error out=w1930:errorcluster)  [unwired: 2 out]
              }
            }
            n1000 = case shown="True" w1920 {
              tunnel: w1922 -> [w1947 w1951]
              tunnel: w1921 -> [w1946 w1950]
              tunnel: [w1947 w1949] -> w1909
              tunnel: [w1946 w1948] -> w1908
              frame #0 {
              }
              frame #1 {
                n1001 = property class="Instr"(reference=w1951, error in=w1950) -> (reference out=w1953:refnum<visa-resource-name>, error out=w1952:errorcluster, "Serial Settings:Number of Bytes at Serial Port"=w1954:u32)
                n1002 = VISA Read(VISA resource name=w1953, byte count=w1954, error in (no error)=w1952) -> (VISA resource name out=w1949:refnum<visa-resource-name>, error out=w1948:errorcluster)  [unwired: 2 out]
              }
            }
          }
          frame #4 {
            n1003 = property on="R Scan" class="Bool (strict)"("Val(Sgnl)"=FALSE ("Slew Ready 2")) -> ()  [unwired: 2 in, 2 out]
            n1004 = property on="Z Scan" class="Bool (strict)"("Val(Sgnl)"=FALSE ("Slew Ready 2")) -> ()  [unwired: 2 in, 2 out]
            n1005 = property on="X Scan" class="Bool (strict)"("Val(Sgnl)"=FALSE ("Slew Ready 2")) -> ()  [unwired: 2 in, 2 out]
            n1006 = property on="Y Scan" class="Bool (strict)"("Val(Sgnl)"=FALSE ("Slew Ready 2")) -> ()  [unwired: 2 in, 2 out]
            n1007 = property on="R Scan Length SP steps" class="DigNum (strict)"("DisabledEnum"=T1."Enabled" ("Disabled")) -> ()  [unwired: 2 in, 2 out]
            n1008 = property on="X Scan Length SP steps" class="DigNum (strict)"("DisabledEnum"=T1."Enabled" ("Disabled")) -> ()  [unwired: 2 in, 2 out]
            n1009 = property on="Y Scan Selocity SP steps/sec" class="DigNum (strict)"("DisabledEnum"=T1."Enabled" ("Disabled")) -> ()  [unwired: 2 in, 2 out]
            n1010 = property on="Y Scan Length SP steps" class="DigNum (strict)"("DisabledEnum"=T1."Enabled" ("Disabled")) -> ()  [unwired: 2 in, 2 out]
            n1011 = property on="Z Scan Length SP steps" class="DigNum (strict)"("DisabledEnum"=T1."Enabled" ("Disabled")) -> ()  [unwired: 2 in, 2 out]
            n1012 = property on="X Scan Velocity SP steps/sec" class="DigNum (strict)"("DisabledEnum"=T1."Enabled" ("Disabled")) -> ()  [unwired: 2 in, 2 out]
            n1013 = property on="R Scan Velocity SP steps/sec" class="DigNum (strict)"("DisabledEnum"=T1."Enabled" ("Disabled")) -> ()  [unwired: 2 in, 2 out]
            n1014 = property on="Z Scan Velocity SP steps/sec" class="DigNum (strict)"("DisabledEnum"=T1."Enabled" ("Disabled")) -> ()  [unwired: 2 in, 2 out]
            n1015 = property on="Scan Go" class="Bool"("DisabledEnum"=T1."Disabled and Grayed Out" ("Disabled")) -> ()  [unwired: 2 in, 2 out]
            n1016 = property on="Scan Cancel" class="Bool"("DisabledEnum"=T1."Disabled and Grayed Out" ("Disabled")) -> ()  [unwired: 2 in, 2 out]
          }
        }
      }
      event #24 {
        n1017 = event-data() -> ()  [unwired: 1 in, 7 out]
        n1018 = flat-sequence {
          tunnel: [w2012] -> w1987
          tunnel: [w2011] -> w1986
          tunnel: w1993 -> [w2010]
          tunnel: w1992 -> [w2009]
          frame #0 {
            n1019 = property on="Reset Z Motor Steps" class="DigNum (strict)"() -> ("Value"=w2013:i32)  [unwired: 2 in, 2 out]
            n1020 = Number To Decimal String(number=w2013) -> (decimal integer string=w2014:string)  [unwired: 1 in]
            n1021 = call "mDrive Send Command.vi"("error in (no error)"=w2009, "Extra"=w2014, "Command"=T2."Set Current Position", "VISA resource name"=w2010) -> ("error out"=w2011:errorcluster, "VISA resource name out"=w2012:refnum<visa-resource-name>)  [unwired: 3 in, 1 out]
          }
        }
        n1022 = flat-sequence {
          tunnel: w2001 -> [w2026]
          tunnel: w2000 -> [w2025]
          tunnel: [w2024] -> w1999
          tunnel: [w2023] -> w1998
          frame #0 {
            n1023 = property on="Reset Y Motor Steps" class="DigNum (strict)"() -> ("Value"=w2027:i32)  [unwired: 2 in, 2 out]
            n1024 = Number To Decimal String(number=w2027) -> (decimal integer string=w2028:string)  [unwired: 1 in]
            n1025 = call "mDrive Send Command.vi"("error in (no error)"=w2025, "Extra"=w2028, "Command"=T2."Set Current Position", "VISA resource name"=w2026) -> ("error out"=w2023:errorcluster, "VISA resource name out"=w2024:refnum<visa-resource-name>)  [unwired: 3 in, 1 out]
          }
        }
        n1026 = flat-sequence {
          tunnel: [w2003] -> w1989
          tunnel: [w2005] -> w1988
          tunnel: w1991 -> [w2004]
          tunnel: w1990 -> [w2002]
          frame #0 {
            n1027 = property on="Reset R Motor Steps" class="DigNum (strict)"() -> ("Value"=w2006:i32)  [unwired: 2 in, 2 out]
            n1028 = Number To Decimal String(number=w2006) -> (decimal integer string=w2007:string)  [unwired: 1 in]
            n1029 = call "mDrive Send Command.vi"("error in (no error)"=w2002, "Extra"=w2007, "Command"=T2."Set Current Position", "VISA resource name"=w2004) -> ("error out"=w2005:errorcluster, "VISA resource name out"=w2003:refnum<visa-resource-name>)  [unwired: 3 in, 1 out]
          }
        }
        n1030 = flat-sequence {
          tunnel: [w2016] -> w1995
          tunnel: w1996 -> [w2019]
          tunnel: [w2018] -> w1994
          tunnel: w1997 -> [w2017]
          frame #0 {
            n1031 = property on="Reset X Motor Steps" class="DigNum (strict)"() -> ("Value"=w2020:i32)  [unwired: 2 in, 2 out]
            n1032 = Number To Decimal String(number=w2020) -> (decimal integer string=w2021:string)  [unwired: 1 in]
            n1033 = call "mDrive Send Command.vi"("error in (no error)"=w2019, "Extra"=w2021, "Command"=T2."Set Current Position", "VISA resource name"=w2017) -> ("error out"=w2018:errorcluster, "VISA resource name out"=w2016:refnum<visa-resource-name>)  [unwired: 3 in, 1 out]
          }
        }
      }
    }
  }
  n1034 = flat-sequence {
    tunnel: w10 -> [w2034]
    tunnel: w9 -> [w2031]
    frame #0 {
      n1035 = call "mDrive Send Command.vi"("error in (no error)"=w2031, "Command"=T2."Stop", "VISA resource name"=w2034) -> ("error out"=w2032:errorcluster, "VISA resource name out"=w2033:refnum<visa-resource-name>)  [unwired: 4 in, 1 out]
      n1036 = VISA Close(VISA resource name=w2033, error in (no error)=w2032) -> ()  [unwired: 1 out]
    }
  }
  n1037 = flat-sequence {
    tunnel: w87 -> [w2039]
    tunnel: w86 -> [w2036]
    frame #0 {
      n1038 = call "mDrive Send Command.vi"("error in (no error)"=w2036, "Command"=T2."Stop", "VISA resource name"=w2039) -> ("error out"=w2037:errorcluster, "VISA resource name out"=w2038:refnum<visa-resource-name>)  [unwired: 4 in, 1 out]
      n1039 = VISA Close(VISA resource name=w2038, error in (no error)=w2037) -> ()  [unwired: 1 out]
    }
  }
  n1040 = flat-sequence {
    tunnel: w14 -> [w2044]
    tunnel: w13 -> [w2041]
    frame #0 {
      n1041 = call "mDrive Send Command.vi"("error in (no error)"=w2041, "Command"=T2."Stop", "VISA resource name"=w2044) -> ("error out"=w2042:errorcluster, "VISA resource name out"=w2043:refnum<visa-resource-name>)  [unwired: 4 in, 1 out]
      n1042 = VISA Close(VISA resource name=w2043, error in (no error)=w2042) -> ()  [unwired: 1 out]
    }
  }
  n1043 = flat-sequence {
    tunnel: w60 -> [w2049]
    tunnel: w59 -> [w2046]
    frame #0 {
      n1044 = call "mDrive Send Command.vi"("error in (no error)"=w2046, "Command"=T2."Stop", "VISA resource name"=w2049) -> ("error out"=w2047:errorcluster, "VISA resource name out"=w2048:refnum<visa-resource-name>)  [unwired: 4 in, 1 out]
      n1045 = VISA Close(VISA resource name=w2048, error in (no error)=w2047) -> ()  [unwired: 1 out]
    }
  }
  "Y COM PORT" <- w90
  "X COM PORT" <- w65
  "Z COM PORT" <- w52
  "R COM PORT" <- w19
